vi "myRIO_BRig_RT_v0,53__PortC.vi"() -> ()   [LabVIEW 2014]
uses:
  myRIO_BRig_RT__Case_Exp_stateList.ctl
  myRIO_BRig_RT__Case_NonExp_stateList.ctl
  <vilib>/Platform/TimedLoop/XDataNode/timing_clust.ctl
  <vilib>/Platform/TimedLoop/XDataNode/nitl_modes.ctl
  <vilib>/Platform/TimedLoop/XDataNode/wakeup.ctl
  <vilib>/WebDAVClient/Advanced/SessionHandle.ctl
  <vilib>/myRIO/Common/Instrument Driver Framework/myRIO v1.0/UART/vis/myRIO v1.0 Close UART.vi
  <vilib>/FPGAPlugInAG/myRIO-1900/niLvFpga_Open_myRIO-1900.vi
  <vilib>/rvi/interface/common/dynamic/niFpgaDynamicAddResources.vi
  <vilib>/Utility/error.llb/Error Cluster From Error Code.vi
  <vilib>/rvi/errors/niLvFpgaAdjustHostInterfaceError.vi
  <vilib>/FPGAPlugInAG/Dynamic/niLvFpga_Close_Dynamic.vi
  <vilib>/myRIO/Common/Instrument Driver Framework/Utilities/vis/FPGA Ref Manager.vi
  <vilib>/myRIO/Common/Instrument Driver Framework/myRIO v1.0/myRIO v1.0 Reset FPGA.vi
  <vilib>/myRIO/Common/Instrument Driver Framework/myRIO v1.0/IRQ/vis/myRIO v1.0 IRQ Info FGV.vi
  <vilib>/myRIO/Common/Instrument Driver Framework/myRIO v1.0/IRQ/vis/myRIO v1.0 Timer IRQ Info FGV.vi
  <vilib>/myRIO/Common/Instrument Driver Framework/myRIO v1.0/IRQ/vis/myRIO v1.0 ISR Agent.vi
  <vilib>/rvi/interface/nirviOpenFPGA/nirviOpenFPGA.xnode
  myRIO_BRig_FPGA_v3,41__PortC__v2__build.lvbitx
  myRIO_BRig_FPGA_v3,41__PortC__v2.vi
  <vilib>/rvi/interface/nirviReadWriteControl/nirviReadWriteControl.xnode
  <vilib>/Platform/TimedLoop/XDataNode/XDataNode.xnode
  <vilib>/rvi/interface/nirviCloseFPGA/nirviCloseFPGA.xnode
  <vilib>/Platform/TimedLoop/XDataNode/XDNodeRunTimeDep.lvlib
  <vilib>/rvi/interface/Simulation/niFpgaSimulationCallBeginRW.vi
  <vilib>/myRIO/Instrument Drivers/Utilities/Utilities.lvlib
  <vilib>/WebDAVClient/NI_WebDAV.lvlib
  NiFpgaLv.dll
panel:
  in  "Recording_p2":bool
  in  "Recording":bool
  out "error out 3":errorcluster
  out "error out 2":errorcluster
  in  "laser_power":dbl
  in  "f_millisec2count":dbl=117.0
  in  "laser_Tshutter":dbl=2.0
  in  "laser_Freq":dbl=10.0
  in  "laser_Tpeak":dbl=2.0
  in  "laser_duration":u16
  out "error out":errorcluster
  in  "LC_Cue1_All_Count":u16
  in  "LC_Cue1_First_Count":u16
  in  "LC_Cue1_All_delayOpt":bool
  in  "LC_ENL1_All_delayOpt":bool
  in  "LC_ENL1_All_Count":u16
  in  "LC_ENL1_First_Count":u16
  in  "LC_Cue1_First_delayOpt":bool
  in  "LC_ENL1_First_delayOpt":bool
  in  "Tcycle_Cue_max":u16=1000 caption="Max [ms]" min=5 max=5000 step=5
  in  "Tcycle_Cue_min":u16=1000 caption="Min [ms]" min=5 max=5000 step=5
  in  "SendData":bool
  out "cSpout":enum16{"Left", "Right"}(ring) caption="Left or Right Spout"
  out "A4":u32 caption="LickCounter_Right"
  out "A2":u32 caption="LickCounter_Left"
  in  "laserResponse_wrong_LED":bool
  out "error_initTrial":errorcluster
  out "error_Selection_pre":errorcluster
  out "error_Selection":errorcluster
  out "SelectWrong":bool
  out "SelectReward":bool
  in  "Left(F)_or_Right(T)":bool
  in  "ignoreWrong":bool
  in  "SelectionState":bool
  in  "laserResponse_wrong":bool
  in  "laserResponse_reward":bool
  in  "laserResponse_reward_LED":bool
  out "nRewards_Right":u16 caption="# Rewards Total (Right)"
  out "nRewards_Left":u16 caption="# Rewards Total (Left)"
  out "nRewards_cur":u16 caption="# Rewards in Current Block"
  out "TpB_target":u16 caption="Target Trials Per Block"
  out "cState_NonExp":T1 caption="NonExperimental State"
  out "iBlock":u16 caption="Current Block"
  out "cState":T2 caption="Experimental State"
  out "iTrial":u16 caption="Current Trial"
  in  "warmupType":bool
  in  "TestConnection":bool
  in  "warmup":bool caption="WarmUp"
  in  "Host Filename Prefix":string="Exp1_TM2"
  out "Connected To Host?":bool
  in  "Host Password":string="sabalab"
  in  "Host UserName":string="Test2"
  in  "sp_RightSpout":u16(slide)=2 max=2 step=1 scale=0.0..2.0
  in  "sp_LeftSpout":u16(slide)=2 max=2 step=1 scale=0.0..2.0
  in  "BUR_max":u16 caption="Count Reward Structure  (0 = off)"
  in  "LC_Wrong_Probability":u16
  in  "LC_Wrong_Trial":u16(slide) max=2 step=1 scale=0.0..2.0
  in  "LC_Wrong_Block":u16(slide) max=2 step=1 scale=0.0..2.0
  in  "LC_Wrong_OnOff":bool
  in  "LC_Reward_Probability":u16
  in  "LC_Reward_Trial":u16(slide) max=2 step=1 scale=0.0..2.0
  in  "LC_Reward_Block":u16(slide) max=2 step=1 scale=0.0..2.0
  in  "LC_Reward_OnOff":bool
  in  "LC_Cue1_All_Probability":u16
  in  "LC_Cue1_All_Block":u16(slide) max=2 step=1 scale=0.0..2.0
  in  "LC_Cue1_All_OnOff":bool
  in  "LC_Cue1_First_Probability":u16
  in  "LC_Cue1_First_Block":u16(slide) max=2 step=1 scale=0.0..2.0
  in  "LC_Cue1_First_OnOff":bool
  in  "LC_ENL1_All_Probability":u16 max=100 step=1
  in  "LC_ENL1_All_Block":u16(slide) max=2 step=1 scale=0.0..2.0
  in  "LC_ENL1_All_OnOff":bool
  in  "LC_ENL1_First_Probability":u16 max=100 step=1
  in  "LC_ENL1_First_Block":u16(slide) max=2 step=1 scale=0.0..2.0
  in  "Tcycle_Timeout":u16=1000 caption="Timeout Time [ms]" min=10 max=10000 step=1
  in  "Tcycle_Wrong":u16=1000 caption="Wrong Time [ms]" min=10 max=10000 step=1
  in  "Tcycle_Selection":u16=1000 caption="Answer Time [ms]" min=1 max=10000 step=1
  in  "Tcycle_RewardPost":u16=1000 caption="Consumption Time [ms]" min=250 max=10000 step=250
  in  "Tcycle_Reward_L":u16=500 caption="Reward Time [ms]" min=1 max=1000 step=1
  in  "Tcycle_Reward_R":u16=500 caption="Reward Time [ms]" min=1 max=1000 step=1
  in  "TpB_Max_R":u16=4 caption="Max TrialsPerBlock" min=1 max=12 step=1
  in  "TpB_Min_R":u16=4 caption="Min TrialsPerBlock" min=1 max=12 step=1
  in  "TpB_Max_L":u16=4 caption="Max TrialsPerBlock" min=1 max=12 step=1
  in  "TpB_Min_L":u16=4 caption="Min TrialsPerBlock" min=1 max=12 step=1
  in  "BUR_min":u16 caption="Count Reward Structure  (0 = off)"
  in  "TrialUntilReward":bool caption="Ignore Wrong \nSelection"
  in  "CueCycles":u16=1 caption="Cue Structure" min=1 max=1 step=1
  in  "MTrig_Laser_Tcycle":u16=10 caption="Time [ms]"
  in  "MTrig_Laser_trig":bool
  in  "MTrig_Audio_trig__R":bool caption="Trigger Audio"
  in  "MTrig_Audio_trig__L":bool caption="Trigger Audio"
  in  "RewCalib_Trig_R":bool caption="Calibrate_R"
  in  "RewCalib_Trig_L":bool caption="Calibrate_L"
  in  "MTrig_Solenoid_Tcycle__R":u16=300 caption="Time [ms]"
  in  "MTrig_Solenoid_Tcycle__L":u16=300 caption="Time [ms]"
  in  "MTrig_Solenoid_trig__R":bool caption="Solenoid"
  in  "MTrig_Solenoid_trig__L":bool caption="Solenoid"
  in  "STOP_abort":bool caption="Stop LabView\n(Stops myRio and FPGA)"
  in  "STOP_endBlock":bool caption="Stop Experiment\n@ End of Block"
  in  "STOP_endTrial":bool caption="Stop Experiment\n@ End of Trial"
  in  "START":bool caption="Start Experiment"
  in  "Tcycle_CuePenalty":u16=1000 caption="Penalty [ms]" min=1 max=10000 step=1
  in  "Audio_Amp__R":u16=100 caption="Amp"
  in  "Audio_Freq__R":u16=5 caption="Freq [kHz]" max=14 step=1
  in  "Audio_Amp__L":u16=100 caption="Amp"
  in  "Audio_Freq__L":u16=5 caption="Freq [kHz]" max=14 step=1
  in  "LC_Wrong_Tdelay":u16
  in  "LC_Cue1_All_Tdelay":u16
  in  "LC_ENL1_All_Tdelay":u16
  in  "LC_Reward_Tdelay":u16
  in  "LC_Cue1_First_Tdelay":u16
  in  "LC_ENL1_First_Tdelay":u16
  in  "LC_ENL1_First_OnOff":bool
  in  "Tcycle_ENLPenalty":u16=100 caption="Penalty [ms]" min=10 max=10000 step=10
  in  "Tcycle_ENL_max":u16=1000 caption="Max [ms]" min=250 max=10000 step=250
  in  "Tcycle_ENL_min":u16=1000 caption="Min [ms]" min=250 max=10000 step=250
  # "Manual Control"
  # "Task Structure"
  # "Task Timing"
  # "Laser Control\n\n                                                    On/Off      Block        Probability [%]   Delay [ms]                              Count"
  # "Manual Solenoid Trigger\nLeft              Right"
  # "Master Structure"
  # "Enforced NonLick"
  # "Enforced NonLick 1"
  # "from end"
  # "Time = Cue Min"
  # "Min\n \n  \nMax"
  # "Switch Trial"
  # "from start"
  # "(1) = Switching\n(2) = Two Choice"
  # "from end"
  # "NonSwitch Trials"
  # "Cue"
  # "from start"
  # "Cue 1"
  # "from end"
  # "Switch Trial"
  # "from start"
  # "Cue then reward"
  # "Min"
  # "Max"
  # "from end"
  # "Cue with reward"
  # "NonSwitch Trials"
  # "Trial Per Block Structure\n       Left                    Right"
  # "from start"
  # "Spout Selection Control"
  # "Manual Speaker Trigger\nLeft              Right"
  # "Selection Reward"
  # "Answer Time\n         [ms]\n\n  \nWrong Choice Penalty\n         [ms]\n \n \nChoice Timeout Penalty\n         [ms]"
  # "Selection Wrong"
  # "Cue Control"
  # "Left              Right"
  # "State"
  # "Manual Laser Trigger"
  # "Freq [kHz]\n \n \nAmp\n \n\n \n\nSpeaker\nSetting"
  # "Reward Control\n                 Left              Right"
  # "Min = 1\nMax = 32k"
  # "Reward Time\n         [ms]"
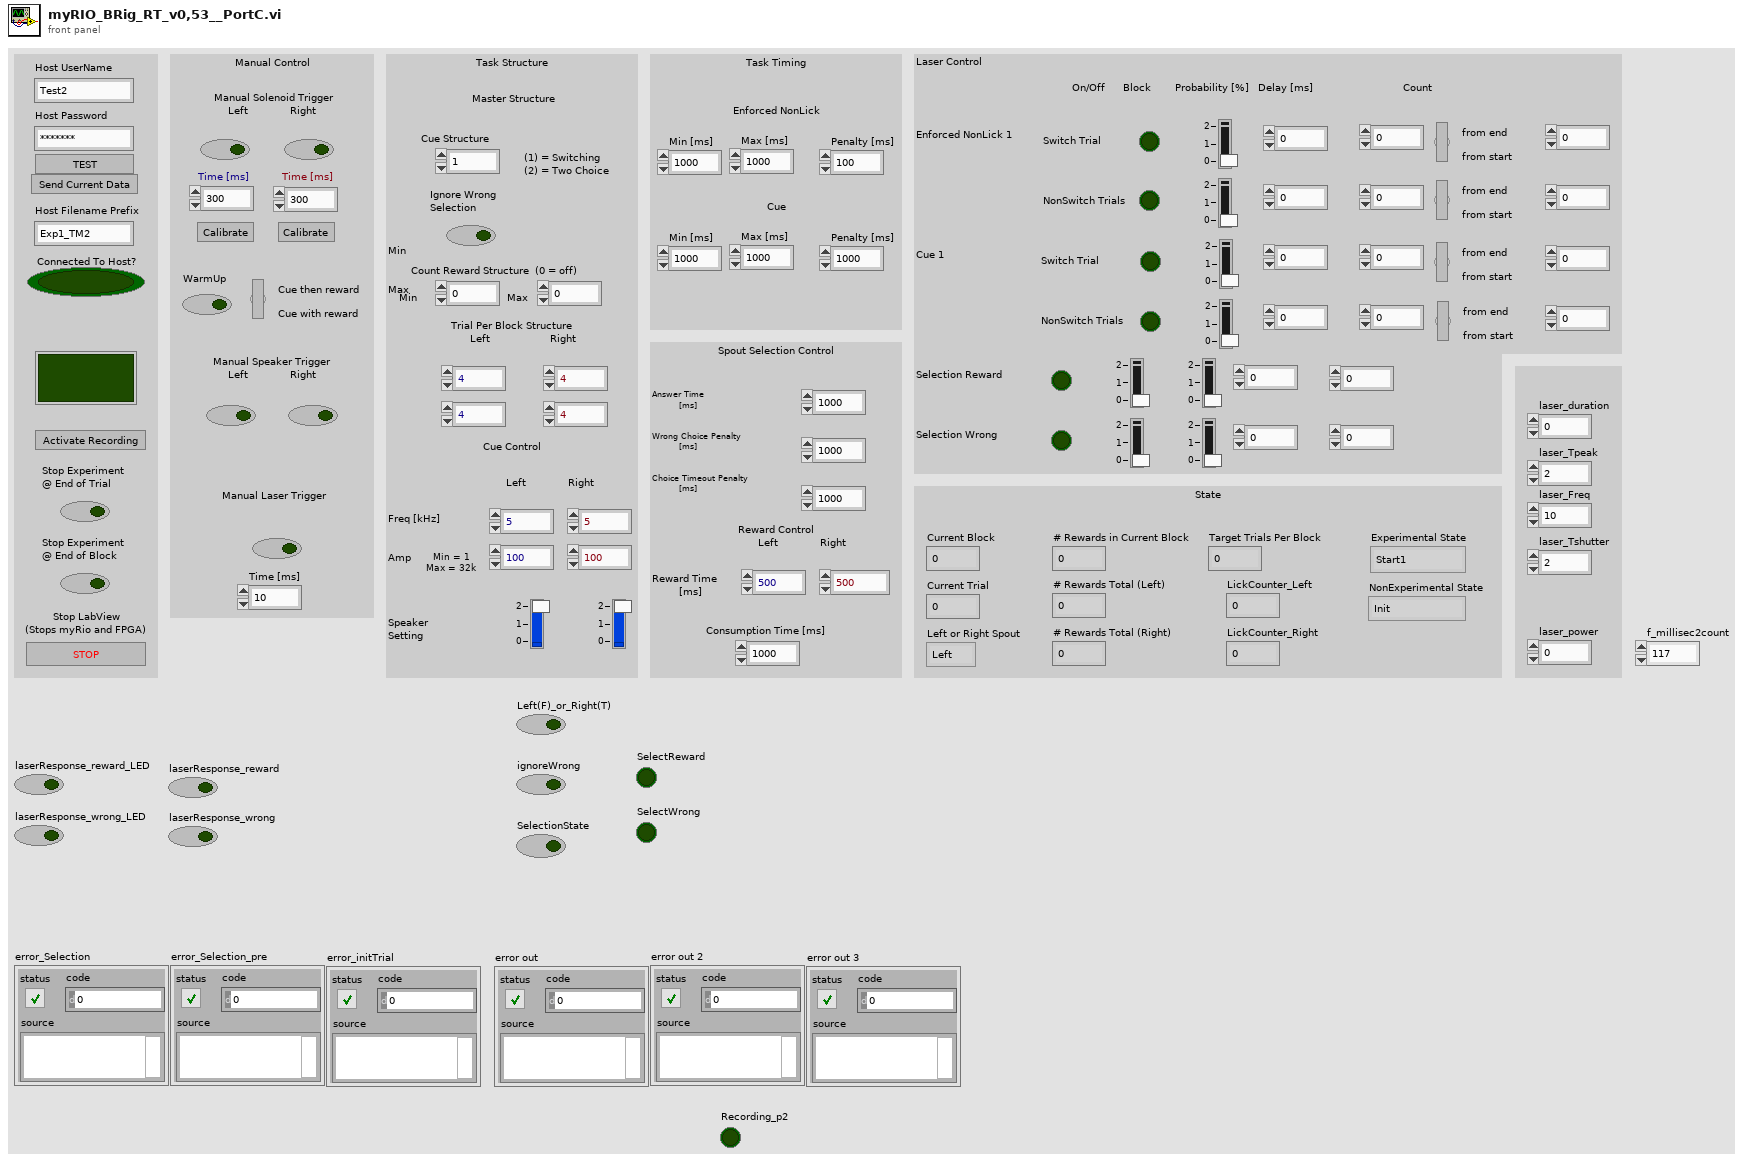
[diagram p1: front panel]
types:
  T1 = typedef "myRIO_BRig_RT__Case_NonExp_stateList.ctl" = enum16{"Init", "UploadSettings_pre", "UploadSettings_Read_dataExp", "UploadSettings_dataExp_1", "UploadSettings_Read_dataLC", "UploadSettings_dataLC_1", "UploadSettings_dataLC_2", "UploadSettings_Read_dataMTrig", "UploadSettings_dataMTrig_1", "UploadSettings_post", "Idle_pre", "IdleEmpty", "IdleEmpty2", "IdleEmpty3", "IdleEmpty4", "Idle", "Idle_2", "Idle_3", "Idle_4", "Idle_post", "Cue_pre__pre", "Cue_pre", "Cue", "Cue_post", "RewardCalibration_pre", "DispenseWater_pre__pre", "DispenseWater_pre", "DispenseWater", "DispenseWater_post", "TestConnection", "SendData", "End"}
  T2 = typedef "myRIO_BRig_RT__Case_Exp_stateList.ctl" = enum16{"Start1", "Start2", "Start3", "saveSettings1", "saveSettings2", "saveSettings3", "saveSettings4_LC_ENL", "saveSettings5_LC_Cue", "saveSettings6_LC_Other", "setSettings_Audio", "setSettings_Laser", "initBlock_pre", "initBlock", "initBlock2", "initBlock_post", "initTrial_pre", "initTrial", "initTrial2", "initTrial3", "initTrial4", "initTrial_LC_ENL1", "initTrial_LC_Cue1", "initTrial_post", "ENL1_pre", "ENL1", "ENL1_post", "ENL1Penalty_pre", "ENL1Penalty", "ENL2_pre", "ENL2", "ENL2Penalty_pre", "ENL2Penalty", "Cue1_pre", "Cue1", "Cue1_post", "Cue1Penalty_pre", "Cue1Penalty", "Cue2_pre", "Cue2", "Cue2Penalty_pre", "Cue2Penalty", "Selection_pre", "Selection", "Select_post", "SelectReward_pre", "SelectReward", "SelectRewardPost_pre", "SelectRewardPost", "SelectWrong_pre", "SelectWrong", "SelectWrong_post", "SelectTimeout_pre", "SelectTimeout", "SelectTimeout_post", "endTrial_pre", "endTrial1", "endTrial2", "endTrial3", "endTrial_post", "endBlock_pre", "endBlock", "endBlock_post", "endExp", "commConnect", "commUpload_pre", "commUpload_dataBlock", "commUpload_dataCurrent", "commUpload_dataExp", "commUpload_dataLC", "commUpload_dataTrial", "commUpload_post", "saveData_pre", "saveData_dataBlock", "saveData_dataCurrent", "saveData_dataExp", "saveData_dataLC", "saveData_dataTrial", "saveData_post", "empty_endBlock1", "empty_endBlock2", "empty_endTrial1", "empty_endTrial2", "empty_endTrial3", "empty_endTrial4", "empty_endTrial5"}
  T3 = typedef "XDNodeRunTimeDep.lvlib/timing_clust.ctl" = cluster{"Expected End [f-1]":u64, "Actual End [f-1]":u64, "Finished Late? [f-1]":bool, "Expected End [i-1]":u64, "Actual End [i-1]":u64, "Finished Late? [i-1]":bool, "Expected Start [i]":u64, "Actual Start [i]":u64, "Expected Start [f]":u64, "Actual Start [f]":u64, "Source Name":string, "Structure Name":string, "Period":i64, "Deadline":i64, "Offset":i64, "Start":i64, "Priority":i32, "Timeout":i32, "Mode":T4, "Wakeup Reason":T5, "Error":errorcluster, "Source Type":string, "Secondary Source Type":string, "Global End Time":u64, "Global Start Time":u64, "Frame Duration":u64, "Iteration Duration":u64, "Assigned CPU":i32, "I/O Scan Engine Mode":u32}
  T4 = typedef "XDNodeRunTimeDep.lvlib/nitl_modes.ctl" = enum32{"No Change", "Process missed periods, maintain original phase", "Discard missed periods, maintain original phase", "Process missed periods, ignore original phase", "Discard missed periods, ignore original phase"}
  T5 = typedef "XDNodeRunTimeDep.lvlib/wakeup.ctl" = enum32{"Normal", "Aborted", "Asynchronous wakeup", "Timing source error", "Timed loop error", "Timeout"}
  T6 = typedef "NI_WebDAV.lvlib/SessionHandle.ctl" = refnum<k1>
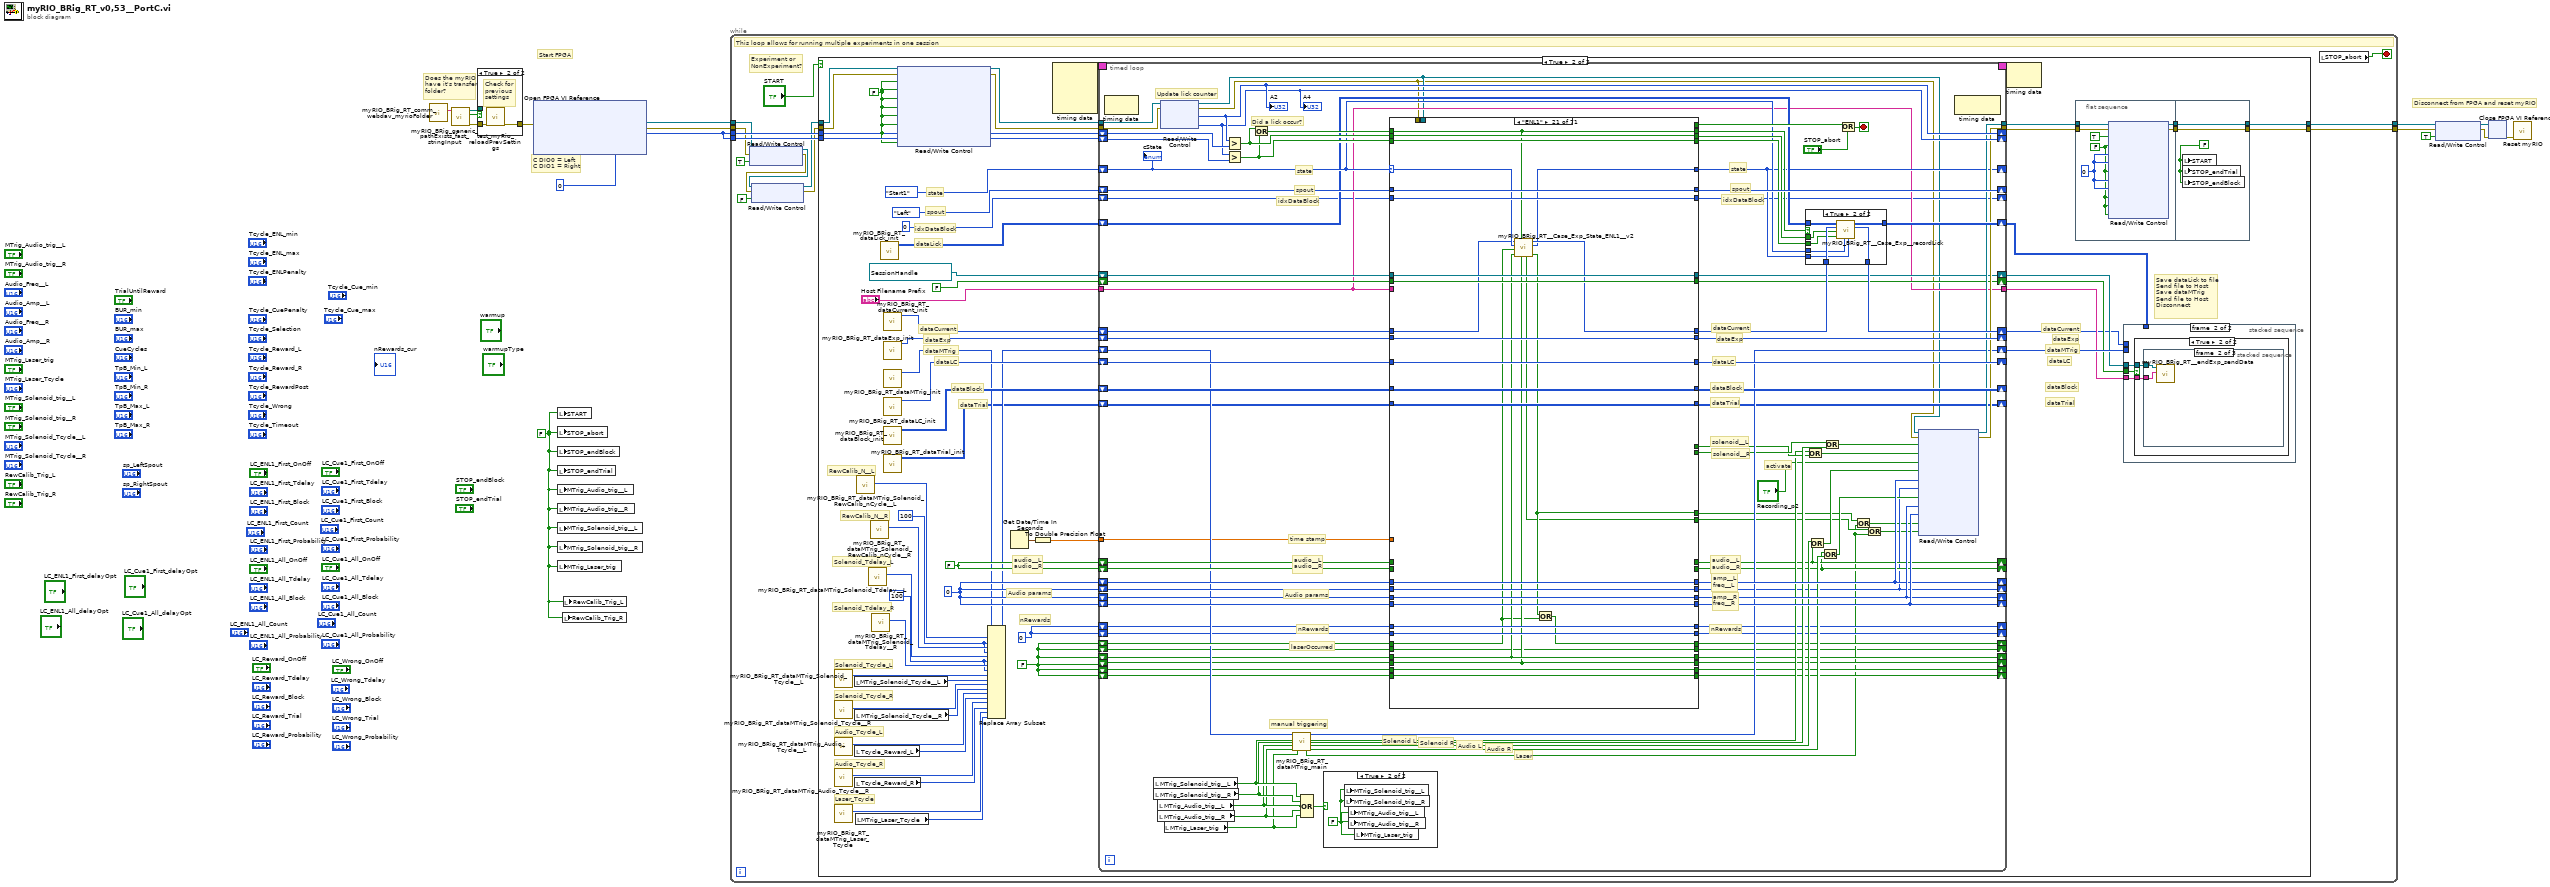
[diagram p0: block diagram]
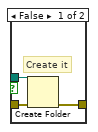
[diagram p2: hidden frame]
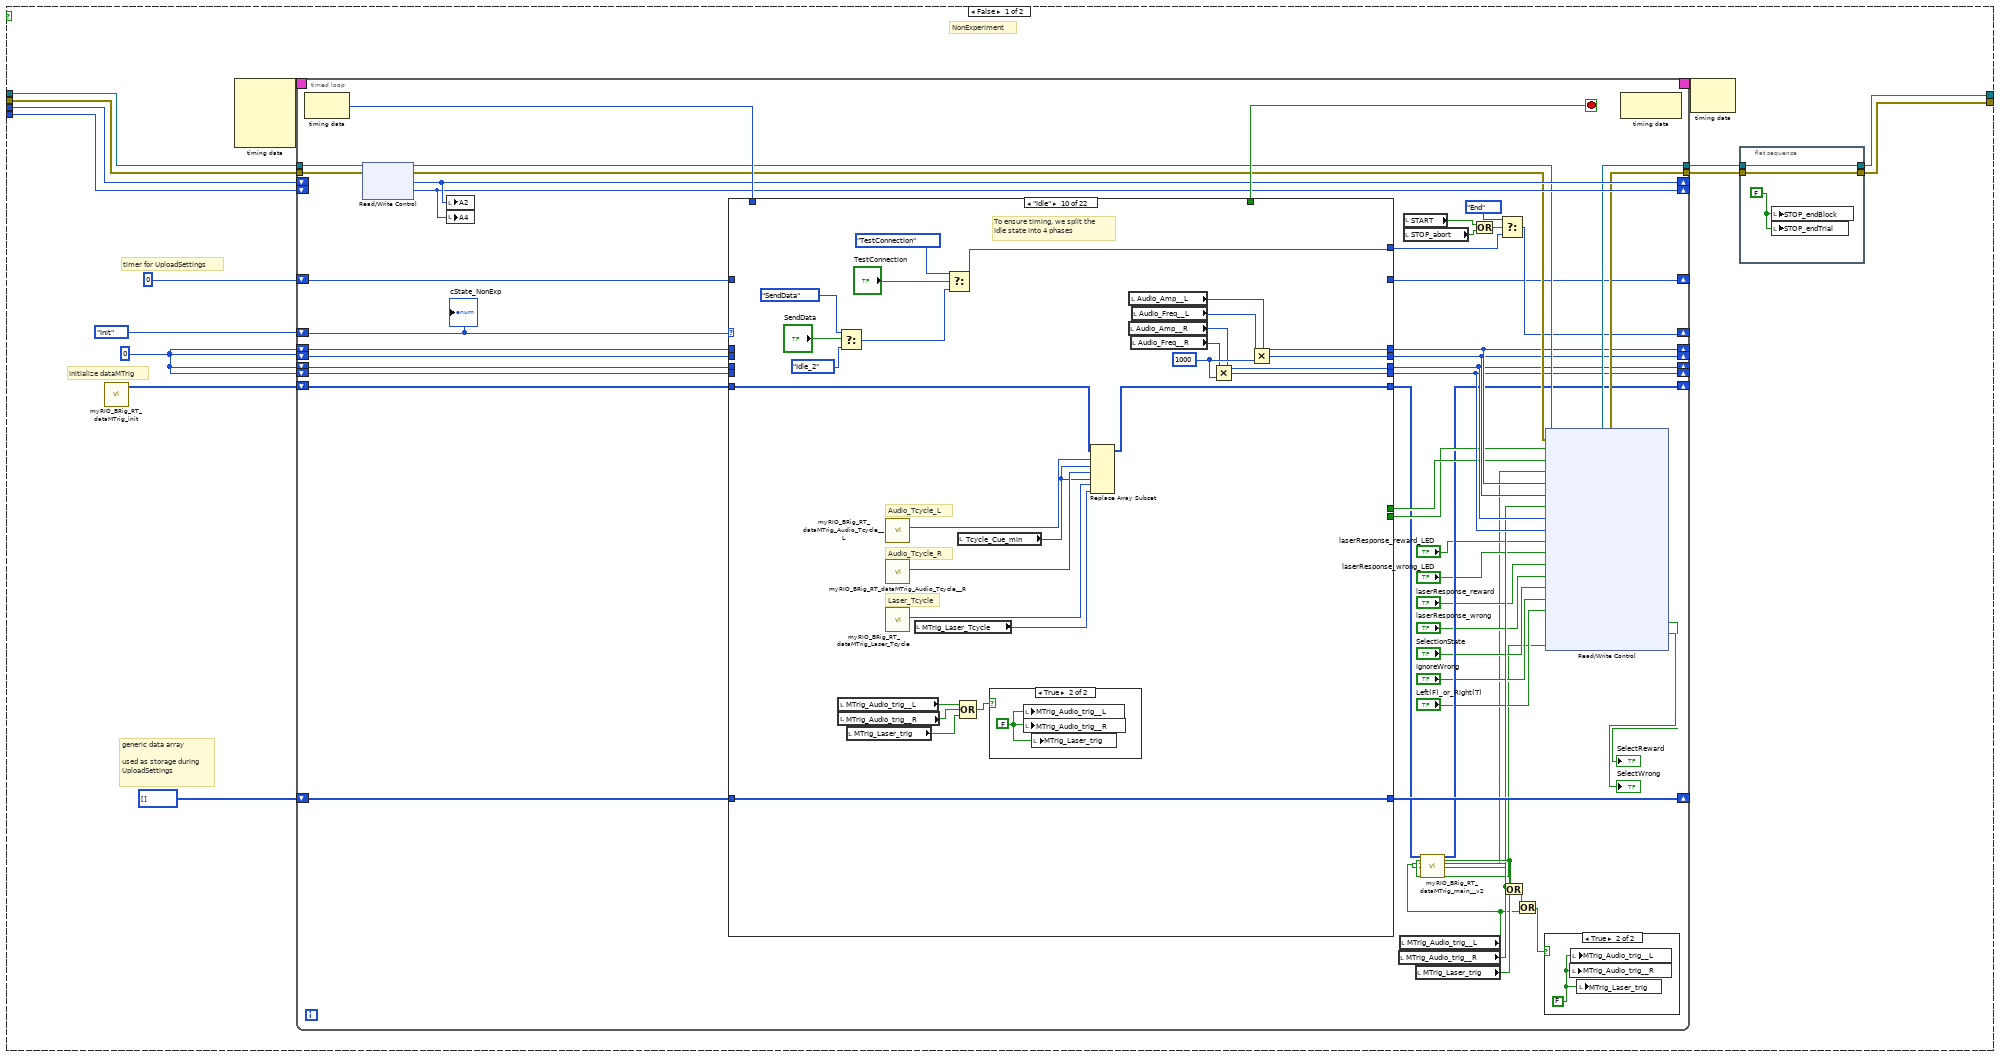
[diagram p3: hidden frame]
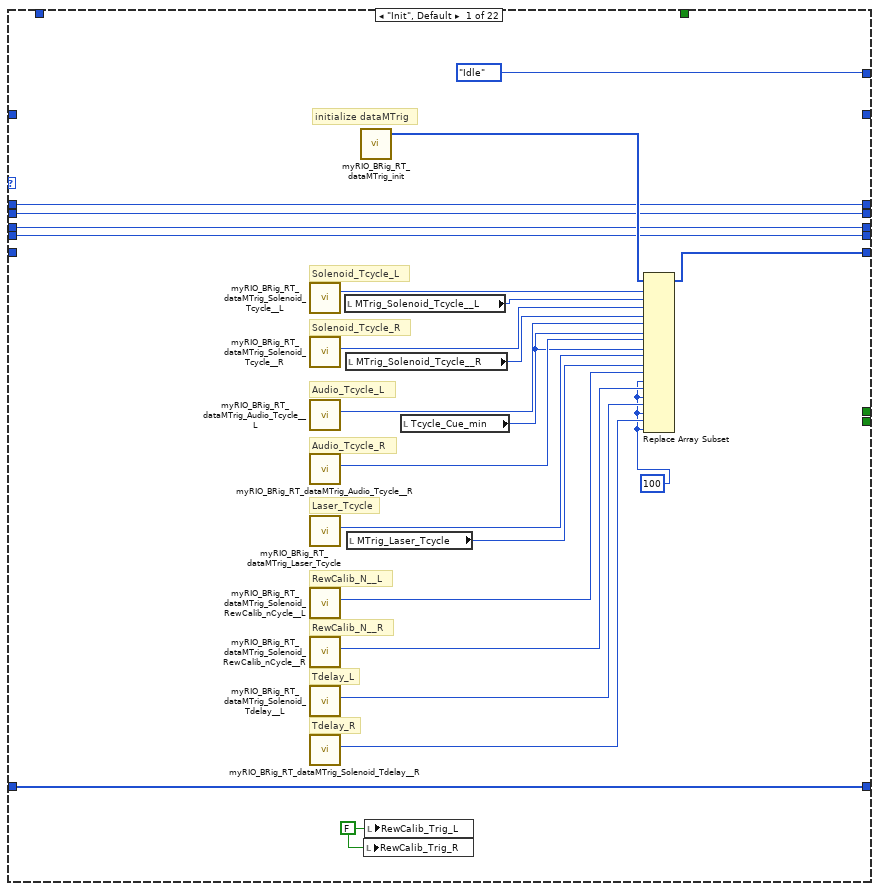
[diagram p5: hidden frame]
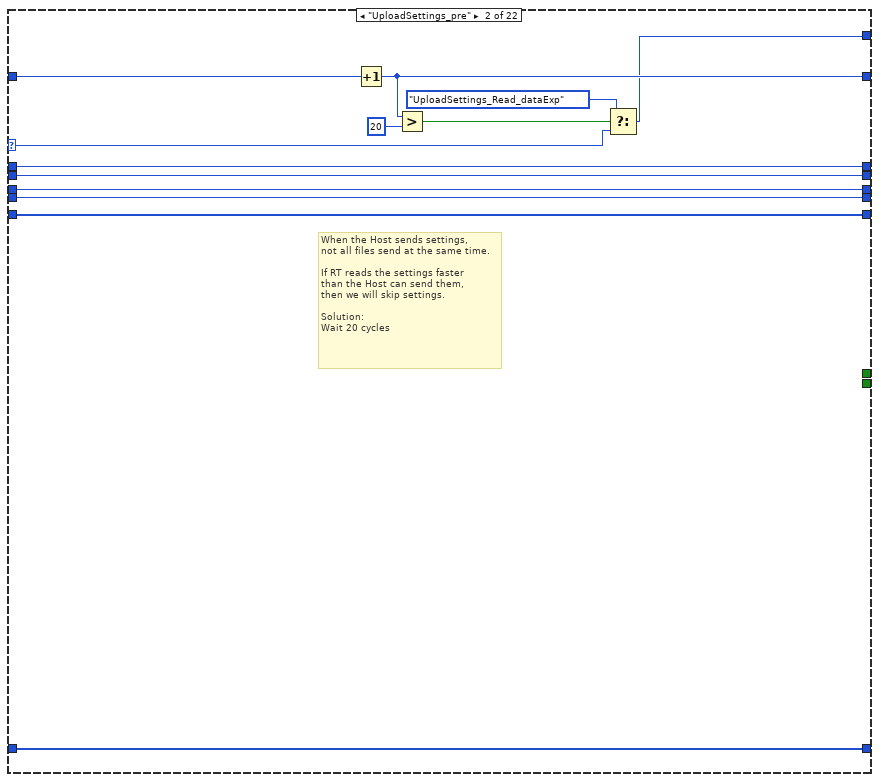
[diagram p6: hidden frame]
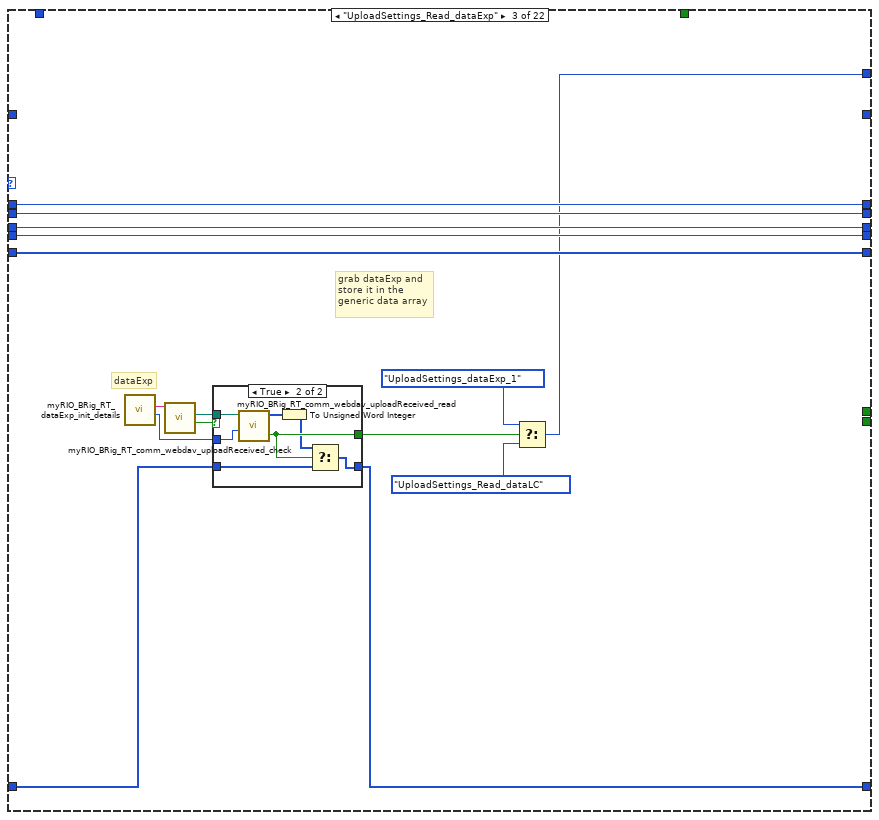
[diagram p7: hidden frame]
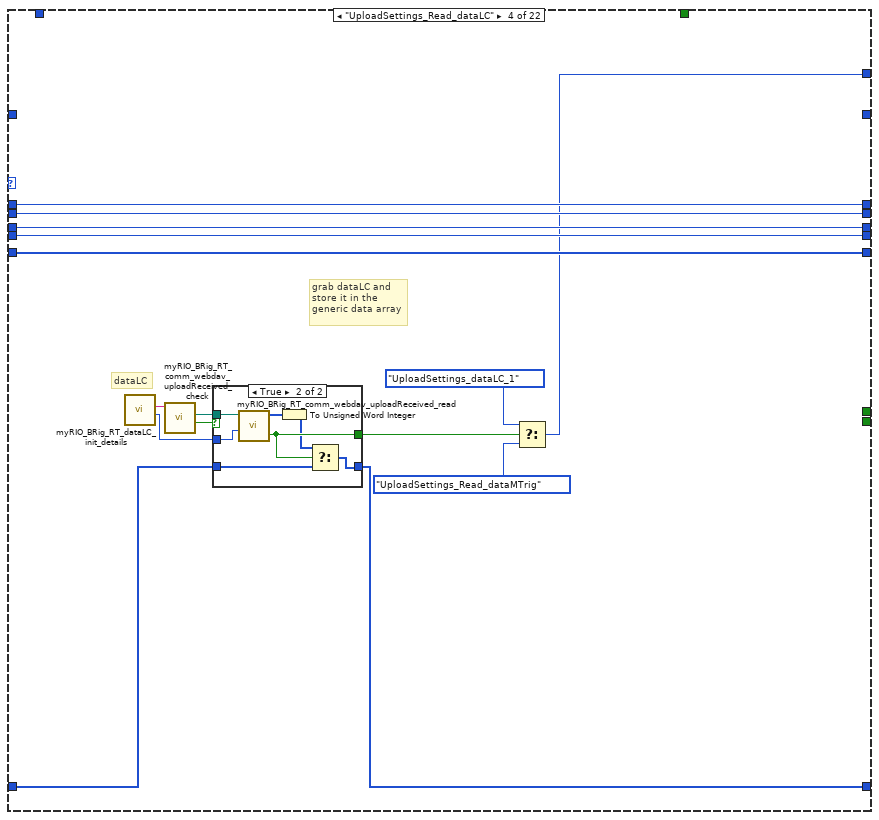
[diagram p9: hidden frame]
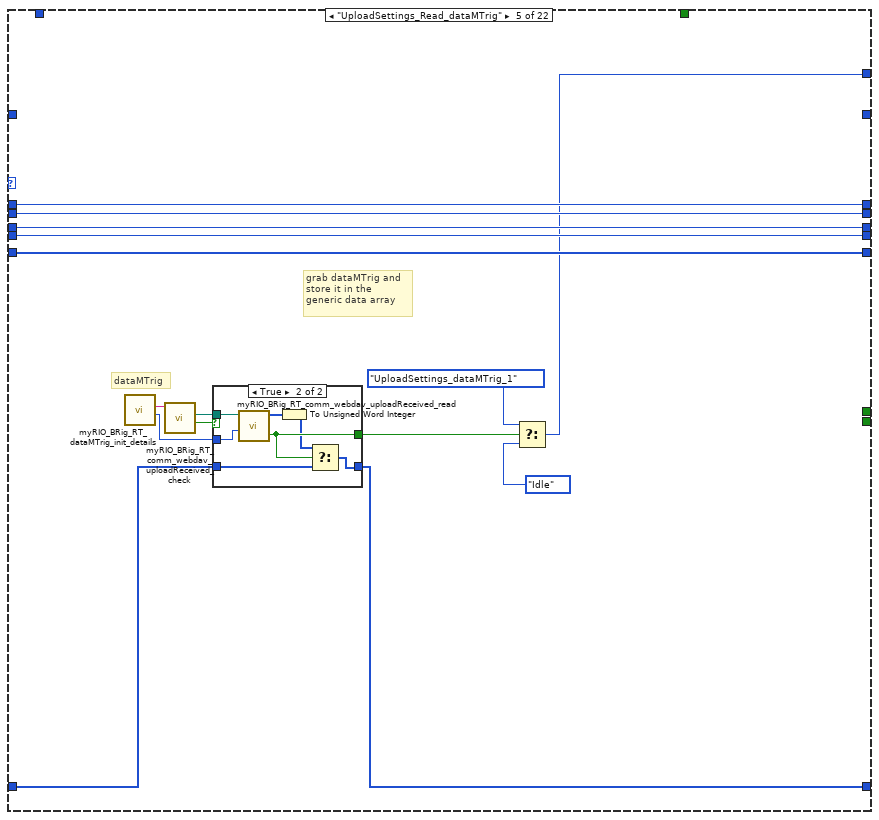
[diagram p11: hidden frame]
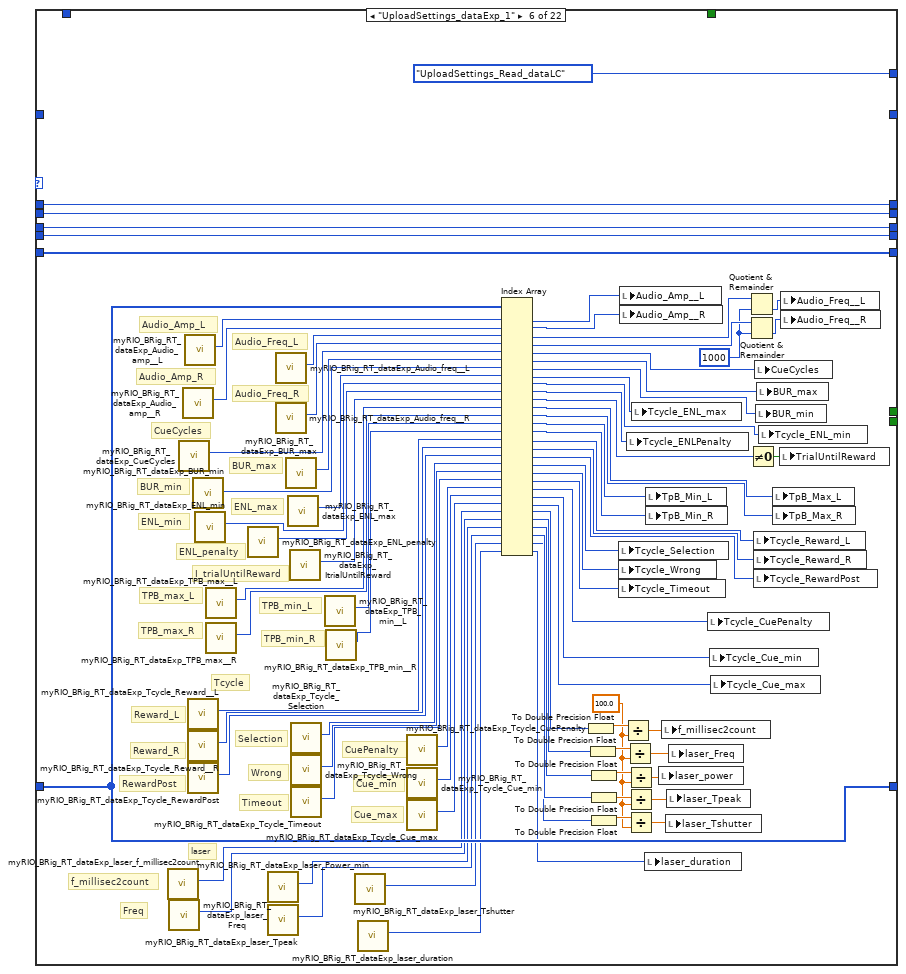
[diagram p13: hidden frame]
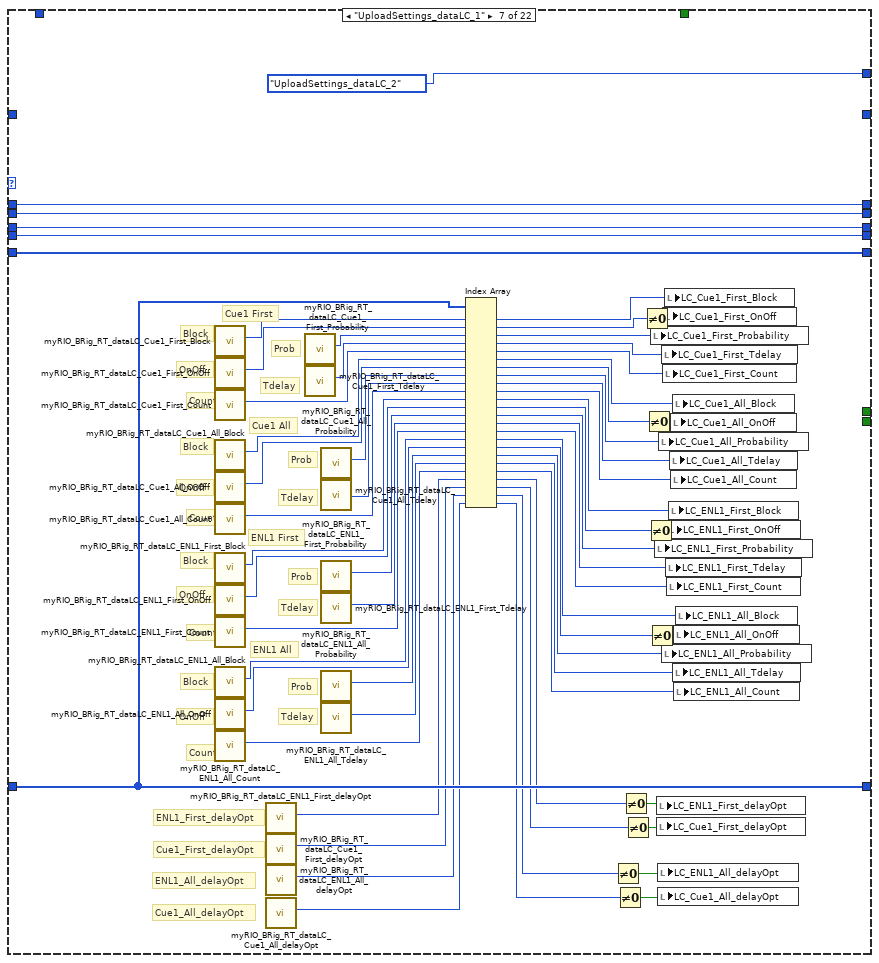
[diagram p14: hidden frame]
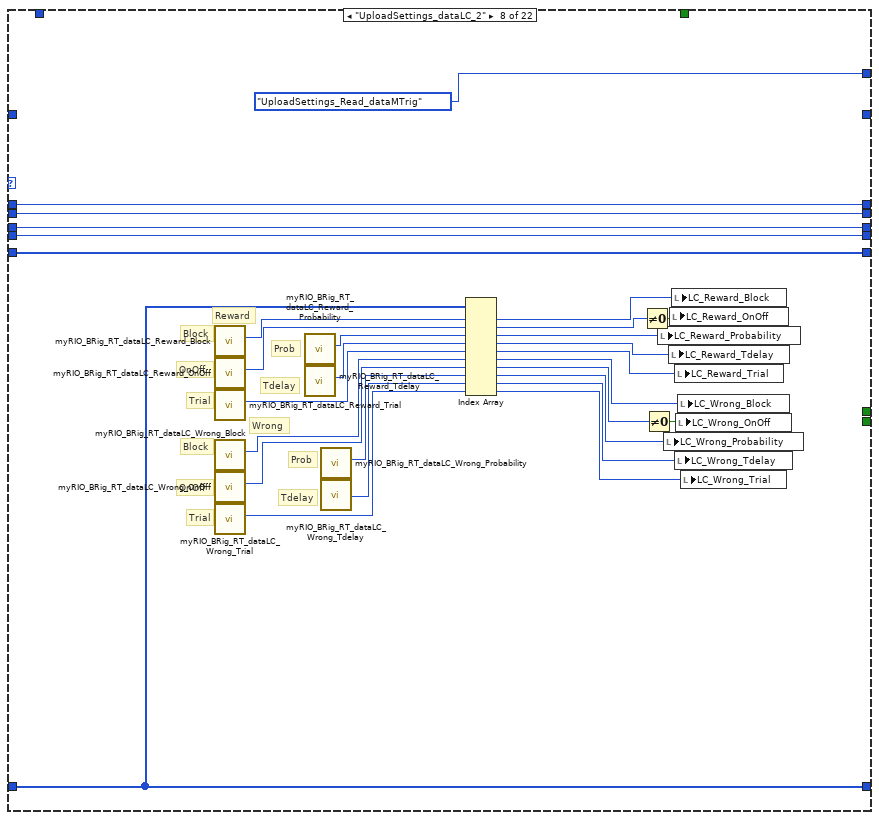
[diagram p15: hidden frame]
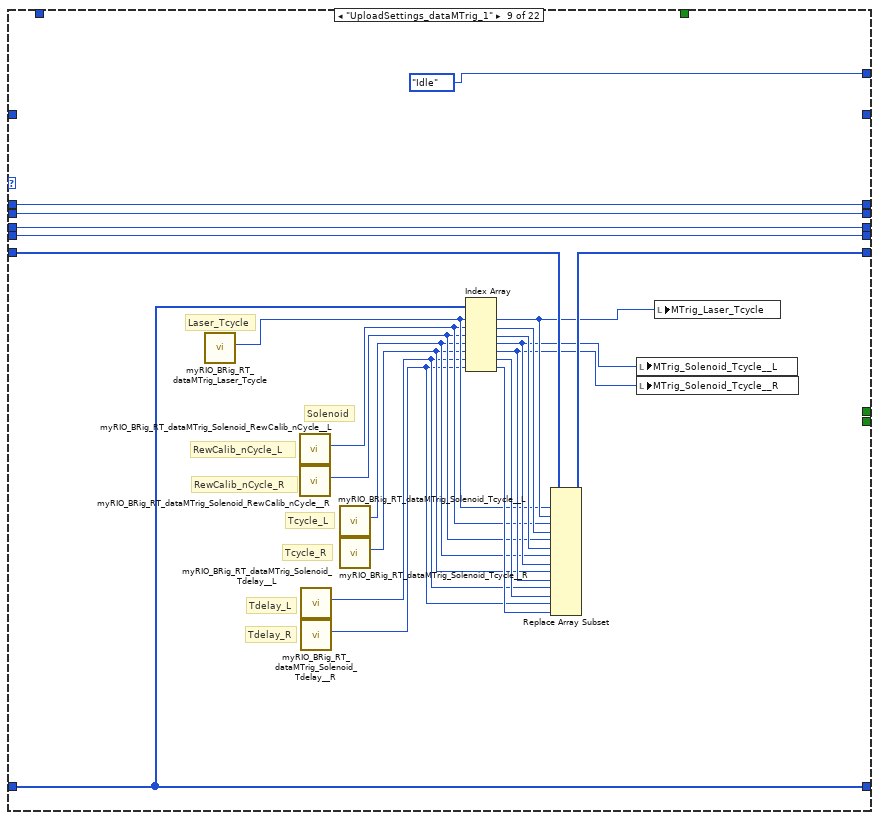
[diagram p16: hidden frame]
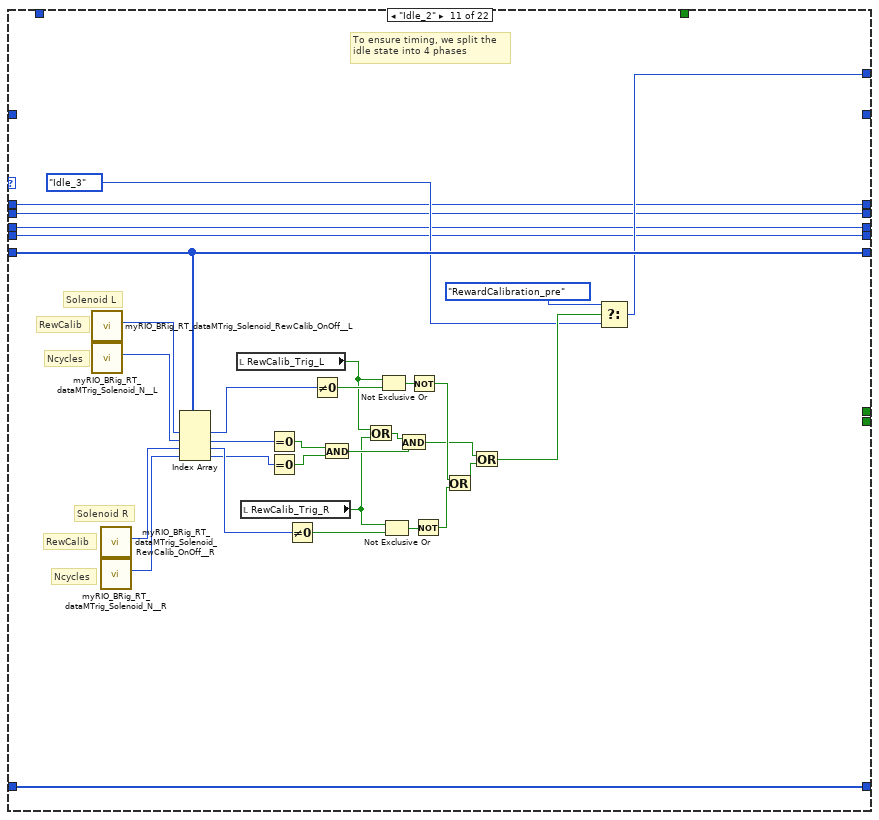
[diagram p18: hidden frame]
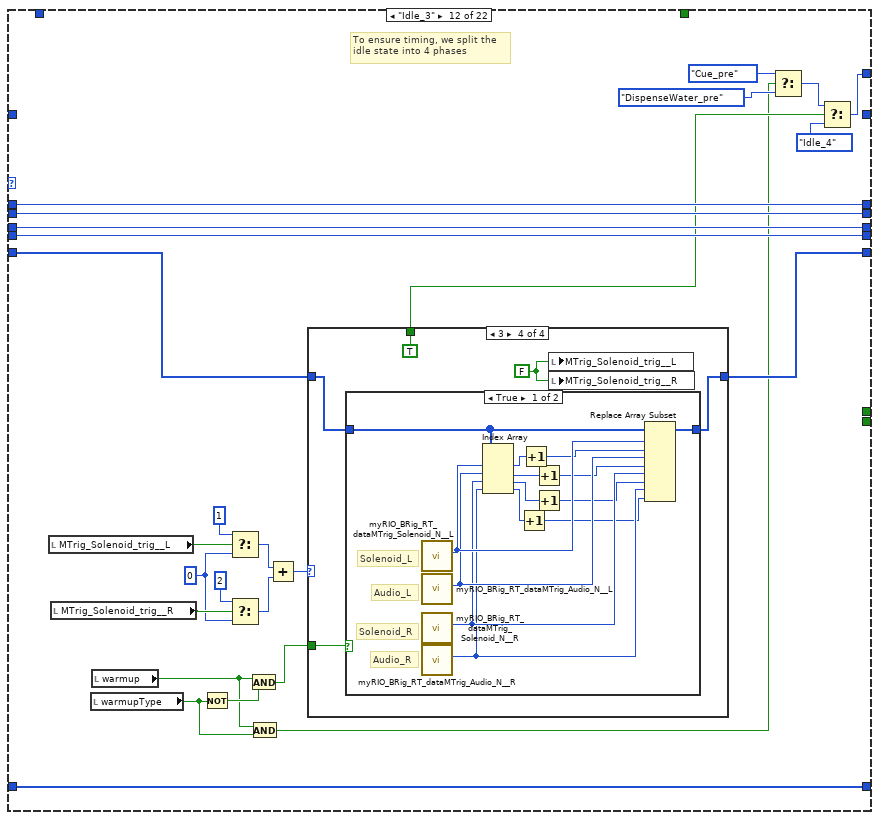
[diagram p19: hidden frame]
diagram:
  w9 = u32 0
  w6 = FALSE
  # "Does the myRIO\nhave it's transfer\nfolder?"
  # "C DIO0 = Left\nC DIO1 = Right"
  # "Start FPGA"
  # "Disconnect from FPGA and reset myRIO"
  n1 = call "myRIO_BRig_RT_comm_webdav_myrioFolder.vi"() -> ("output_myrioFolder"=w4:string)  [unwired: 11 in]
  n2 = call "myRIO_BRig_generic_pathExists_fast_stringInput.vi"("input_filePath"=w4) -> ("output_error"=w3:errorcluster, "output_Iexist"=w2:bool, "output_filePath"=w1:path)  [unwired: 8 in]
  n3 = case shown="True" w2 {
    tunnel: w1 -> [w18 _]
    tunnel: w3 -> [w17 w20]
    tunnel: [w16 w19] -> w5
    frame False {
      # "Create it"
      n4 = Create Folder(path (use dialog)=w18, error in=w17) -> (error out=w16:errorcluster)  [unwired: 1 in, 2 out]
    }
    frame True {
      # "Check for\nprevious\nsettings"
      n5 = call "test_myRio_reloadPrevSettings.vi"("input_error"=w20) -> ("output_error"=w19:errorcluster)  [unwired: 10 in]
    }
  }
  n6 = xnode "Open FPGA VI Reference"("error in"=w5) -> ("FPGA VI Reference Out"=w11:refnum<k20>, "error out"=w10:errorcluster)  [unwired: 1 in]
  n7 = local write "START"(w6) -> ()
  n8 = local write "STOP_abort"(w6) -> ()
  n9 = local write "STOP_endBlock"(w6) -> ()
  n10 = local write "STOP_endTrial"(w6) -> ()
  n11 = local write "MTrig_Audio_trig__L"(w6) -> ()
  n12 = local write "MTrig_Audio_trig__R"(w6) -> ()
  n13 = local write "MTrig_Solenoid_trig__L"(w6) -> ()
  n14 = local write "MTrig_Solenoid_trig__R"(w6) -> ()
  n15 = local write "MTrig_Laser_trig"(w6) -> ()
  n16 = local write "RewCalib_Trig_R"(w6) -> ()
  n17 = local write "RewCalib_Trig_L"(w6) -> ()
  n18 = while {
    tunnel: w11 -> [w24]
    tunnel: w10 -> [w29]
    tunnel: w9 -> [w32]
    tunnel: w9 -> [w31]
    tunnel: [w22] -> w8
    tunnel: [w21] -> w7
    stop <- w30 stop-if-true
    # "Experiment or\nNonExperiment?"
    # "This loop allows for running multiple experiments in one session"
    n19 = xnode "Read/Write Control"("FPGA VI Reference In"=w24, "error in"=w29, "Counts_Reset"=TRUE) -> ("FPGA VI Reference Out"=w26:refnum<k20>, "error out"=w27:errorcluster)
    n20 = xnode "Read/Write Control"("FPGA VI Reference In"=w26, "error in"=w27, "Counts_Reset"=FALSE) -> ("FPGA VI Reference Out"=w23:refnum<k20>, "error out"=w25:errorcluster)
    n21 = case shown="True" "START" {
      tunnel: w32 -> [w45 w932]
      tunnel: w31 -> [w44 w931]
      tunnel: w25 -> [w42 w882]
      tunnel: w23 -> [w43 w881]
      tunnel: [w40 w928] -> w22
      tunnel: [w38 w923] -> w21
      frame False {
        w37 = u16 0 ("Audio_Amp__L")
        # "generic data array\n\nused as storage during\nUploadSettings"
        # "timer for UploadSettings"
        # "initialize dataMTrig"
        # "NonExperiment"
        n22 = call "myRIO_BRig_RT_dataMTrig_init.vi"() -> ("output_dataMTrig"=w46:u16[])  [unwired: 5 in]
        n23 = node-c288() -> (w49:T3)  [unwired: 4 in]
        n24 = timed-loop {
          timing: w49 -> [_]
          timing-out: [_] -> w48
          shift-right: [w78] -> _
          shift-left: w46 -> [w102]
          shift-right: [w67] -> _
          shift-left: myRIO_BRig_RT__Case_NonExp_stateList."Init" ("Enum") -> [w92]
          shift-right: [w100] -> _
          shift-left: w45 -> [_]
          shift-right: [w99] -> _
          shift-left: w44 -> [_]
          tunnel: [w95] -> w41
          tunnel: [w93] -> w39
          tunnel: w42 -> [w98]
          tunnel: w43 -> [w97]
          shift-right: [w91] -> _
          shift-left: u16[] [] ("output_data") -> [w90]
          shift-right: [w85] -> _
          shift-left: w37 -> [w89]
          shift-right: [w84] -> _
          shift-left: w37 -> [w88]
          shift-right: [w83] -> _
          shift-left: w37 -> [w87]
          shift-right: [w82] -> _
          shift-left: w37 -> [w86]
          shift-right: [w53] -> _
          shift-left: u16 0 ("Audio_Amp__L") -> [w54]
          stop <- w103 stop-if-true
          n25 = node-c288() -> (w101:i64)  [unwired: 1 in]
          n26 = xnode "Read/Write Control"("FPGA VI Reference In"=w97, "error in"=w98) -> ("FPGA VI Reference Out"=w96:refnum<k20>, "error out"=w94:errorcluster, "A2_LickL"=w100:u32, "A4_LickR"=w99:u32)
          n27 = local write "A2"(w100) -> ()
          n28 = local write "A4"(w99) -> ()
          n29 = case shown="\"Idle\"" w92 {
            selector: w92 -> [_ w136 _ _ _ _ _ _ _ _ _ _ _ _ w591 _ _ w776 _ _ _ w873]
            tunnel: [myRIO_BRig_RT__Case_NonExp_stateList."Idle" ("Enum") w134 w141 w164 w187 myRIO_BRig_RT__Case_NonExp_stateList."UploadSettings_Read_dataLC" ("Enum") myRIO_BRig_RT__Case_NonExp_stateList."UploadSettings_dataLC_2" ("Enum") myRIO_BRig_RT__Case_NonExp_stateList."UploadSettings_Read_dataMTrig" ("f") myRIO_BRig_RT__Case_NonExp_stateList."Idle" ("Enum") w417 w438 w471 w562 myRIO_BRig_RT__Case_NonExp_stateList."Cue" ("t") w590 myRIO_BRig_RT__Case_NonExp_stateList."DispenseWater_pre" ("Enum") w718 w774 w801 myRIO_BRig_RT__Case_NonExp_stateList."Idle" ("Enum") myRIO_BRig_RT__Case_NonExp_stateList."Idle" ("Enum") w873] -> w68
            tunnel: [w119 w129 w151 w174 w197 w291 w354 w383 w403 w428 w453 w482 w560 w578 w604 w628 w755 w781 w812 w855 w865 w871] -> w79
            tunnel: [_ _ _ _ _ _ _ _ _ _ _ _ _ _ _ _ _ _ _ _ _ TRUE] -> w103
            tunnel: w102 -> [_ w129 w151 w174 w197 w291 w354 w383 w404 w427 w453 w483 w560 w579 w604 w614 w751 w782 w813 w855 w865 w871]
            tunnel: w101 -> [_ _ _ _ _ _ _ _ _ _ _ _ _ _ _ _ _ w786 _ _ _ _]
            tunnel: [w108 w128 w142 w165 w188 w235 w306 w355 w384 w412 w433 w465 w555 w566 w589 w605 w703 w759 w794 w843 w859 w866] -> w91
            tunnel: w90 -> [w108 w128 w143 w166 w189 w235 w306 w355 w384 w412 w433 w465 w555 w566 w589 w605 w703 w759 w794 w843 w859 w866]
            tunnel: [w112 w132 w154 w177 w200 w288 w352 w358 w401 w423 w436 w475 w557 w586 w601 w608 w757 w792 w819 w846 w862 w869] -> w84
            tunnel: [w110 w130 w152 w175 w198 w286 w350 w356 w399 w422 w434 w477 w559 w584 w603 w606 w756 w790 w817 w844 w860 w867] -> w82
            tunnel: [w113 w133 w155 w178 w201 w289 w353 w359 w402 w421 w437 w474 w556 w588 w600 w609 w758 w793 w820 w847 w863 w870] -> w85
            tunnel: [w111 w131 w153 w176 w199 w287 w351 w357 w400 w420 w435 w476 w558 w585 w602 w607 w756 w791 w818 w845 w861 w868] -> w83
            tunnel: w89 -> [w113 w133 w155 w178 w201 w289 w353 w359 w402 _ w437 w474 w556 w588 w600 w609 w758 w793 w820 w847 w863 w870]
            tunnel: w88 -> [w112 w132 w154 w177 w200 w288 w352 w358 w401 _ w436 w475 w557 w586 w601 w608 w757 w792 w819 w846 w862 w869]
            tunnel: w87 -> [w111 w131 w153 w176 w199 w287 w351 w357 w400 _ w435 w476 w558 w585 w602 w607 w756 w791 w818 w845 w861 w868]
            tunnel: w86 -> [w110 w130 w152 w175 w198 w286 w350 w356 w399 _ w434 w477 w559 w584 w603 w606 _ w790 w817 w844 w860 w867]
            tunnel: [_ _ _ _ _ _ _ _ _ _ _ _ _ _ _ _ _ w783 _ _ _ _] -> w81
            tunnel: [_ _ _ _ _ _ _ _ _ _ _ _ _ _ _ _ _ w765 _ _ _ _] -> w80
            tunnel: w54 -> [_ w140 _ _ _ _ _ _ _ _ _ _ _ _ _ _ _ _ _ _ _ _]
            tunnel: [_ w139 _ _ _ _ _ _ _ _ _ _ _ _ _ _ _ _ _ _ _ _] -> w53
            frame "Init", Default {
              w109 = FALSE ("RewCalib_Trig_L")
              w105 = u16 100 ("new element/subarray")
              # "Tdelay_R"
              # "Tdelay_L"
              # "RewCalib_N__R"
              # "RewCalib_N__L"
              # "Solenoid_Tcycle_R"
              # "Solenoid_Tcycle_L"
              # "Laser_Tcycle"
              # "Audio_Tcycle_R"
              # "Audio_Tcycle_L"
              # "initialize dataMTrig"
              n30 = call "myRIO_BRig_RT_dataMTrig_Solenoid_Tcycle__L.vi"() -> ("output_Solenoid_Tcycle__L"=w121:i32)  [unwired: 11 in]
              n31 = call "myRIO_BRig_RT_dataMTrig_Solenoid_Tcycle__R.vi"() -> ("output_Solenoid_Tcycle__R"=w122:i32)  [unwired: 11 in]
              n32 = call "myRIO_BRig_RT_dataMTrig_Audio_Tcycle__L.vi"() -> ("output_Audio_Tcycle__L"=w123:i32)  [unwired: 11 in]
              n33 = call "myRIO_BRig_RT_dataMTrig_Audio_Tcycle__R.vi"() -> ("output_Audio_Tcycle__R"=w124:i32)  [unwired: 11 in]
              n34 = call "myRIO_BRig_RT_dataMTrig_Laser_Tcycle.vi"() -> ("output_Laser_Tcycle"=w125:i32)  [unwired: 11 in]
              n35 = call "myRIO_BRig_RT_dataMTrig_Solenoid_RewCalib_nCycle__L.vi"() -> ("output_Solenoid_RewCalib_nCycle__L"=w117:i32)  [unwired: 11 in]
              n36 = call "myRIO_BRig_RT_dataMTrig_Solenoid_RewCalib_nCycle__R.vi"() -> ("output_Solenoid_RewCalib_nCycle__R"=w116:i32)  [unwired: 11 in]
              n37 = call "myRIO_BRig_RT_dataMTrig_Solenoid_Tdelay__L.vi"() -> ("output_Solenoid_Tdelay__L"=w115:i32)  [unwired: 11 in]
              n38 = call "myRIO_BRig_RT_dataMTrig_Solenoid_Tdelay__R.vi"() -> ("output_Solenoid_Tdelay__R"=w114:i32)  [unwired: 11 in]
              n39 = local read "MTrig_Solenoid_Tcycle__L"() -> (w126:u16)
              n40 = local read "MTrig_Solenoid_Tcycle__R"() -> (w127:u16)
              n41 = local read "MTrig_Laser_Tcycle"() -> (w106:u16)
              n42 = call "myRIO_BRig_RT_dataMTrig_init.vi"() -> ("output_dataMTrig"=w120:u16[])  [unwired: 5 in]
              n43 = local write "RewCalib_Trig_R"(w109) -> ()
              n44 = local write "RewCalib_Trig_L"(w109) -> ()
              n45 = local read "Tcycle_Cue_min"() -> (w107:u16)
              n46 = Replace Array Subset(array=w120, new element #1=w126, index #1=w121, new element #2=w127, index #2=w122, new element #3=w107, index #3=w123, new element #4=w107, index #4=w124, new element #5=w106, index #5=w125, new element #6=w105, index #6=w117, new element #7=w105, index #7=w116, new element #8=w105, index #8=w115, new element #9=w105, index #9=w114) -> (w119:u16[])
            }
            frame "UploadSettings_pre" {
              # "When the Host sends settings,\nnot all files send at the same time.\n\nIf RT reads the settings faster\nthan the Host can send them,\nthen we will skip settings.\n\nSolution:\nWait 20 cycles"
              n47 = Increment(x=w140) -> (x+1=w139:u16)
              n48 = Greater?(x=w139, y=u16 20) -> (0:w137:bool)
              n49 = Select(t=myRIO_BRig_RT__Case_NonExp_stateList."UploadSettings_Read_dataExp", s=w137, f=w136) -> (s? t:f=w134:T1)
            }
            frame "UploadSettings_Read_dataExp" {
              # "grab dataExp and\nstore it in the\ngeneric data array"
              # "dataExp"
              n50 = call "myRIO_BRig_RT_dataExp_init_details.vi"() -> ("output_dataSize"=w147:i32, "output_dataName"=w150:string)  [unwired: 10 in]
              n51 = call "myRIO_BRig_RT_comm_webdav_uploadReceived_check.vi"("input_dataName"=w150) -> ("output_Iexist"=w149:bool, "output_dataPath"=w148:path)  [unwired: 9 in]
              n52 = case shown="True" w149 {
                tunnel: w148 -> [_ w163]
                tunnel: w147 -> [_ w162]
                tunnel: [_ w161] -> w146
                tunnel: w143 -> [w156 w160]
                tunnel: [w156 w157] -> w142
                frame False {
                }
                frame True {
                  n53 = call "myRIO_BRig_RT_comm_webdav_uploadReceived_read.vi"("input_dataSize"=w162, "input_filePath"=w163) -> ("output_Ivalid"=w161:bool, "output_data"=w159:i64[])  [unwired: 8 in]
                  n54 = To Unsigned Word Integer(number=w159) -> (unsigned 16bit integer=w158:u16[])
                  n55 = Select(t=w158, s=w161, f=w160) -> (s? t:f=w157:u16[])
                }
              }
              n56 = Select(t=myRIO_BRig_RT__Case_NonExp_stateList."UploadSettings_dataExp_1", s=w146, f=myRIO_BRig_RT__Case_NonExp_stateList."UploadSettings_Read_dataLC" ("t")) -> (s? t:f=w141:T1)
            }
            frame "UploadSettings_Read_dataLC" {
              # "grab dataLC and\nstore it in the\ngeneric data array"
              # "dataLC"
              n57 = call "myRIO_BRig_RT_dataLC_init_details.vi"() -> ("output_dataSize"=w170:i32, "output_dataName"=w173:string)  [unwired: 10 in]
              n58 = call "myRIO_BRig_RT_comm_webdav_uploadReceived_check.vi"("input_dataName"=w173) -> ("output_Iexist"=w172:bool, "output_dataPath"=w171:path)  [unwired: 9 in]
              n59 = case shown="True" w172 {
                tunnel: w171 -> [_ w186]
                tunnel: w170 -> [_ w185]
                tunnel: [_ w184] -> w169
                tunnel: w166 -> [w179 w183]
                tunnel: [w179 w180] -> w165
                frame False {
                }
                frame True {
                  n60 = call "myRIO_BRig_RT_comm_webdav_uploadReceived_read.vi"("input_dataSize"=w185, "input_filePath"=w186) -> ("output_Ivalid"=w184:bool, "output_data"=w182:i64[])  [unwired: 8 in]
                  n61 = To Unsigned Word Integer(number=w182) -> (unsigned 16bit integer=w181:u16[])
                  n62 = Select(t=w181, s=w184, f=w183) -> (s? t:f=w180:u16[])
                }
              }
              n63 = Select(t=myRIO_BRig_RT__Case_NonExp_stateList."UploadSettings_dataLC_1", s=w169, f=myRIO_BRig_RT__Case_NonExp_stateList."UploadSettings_Read_dataMTrig" ("t")) -> (s? t:f=w164:T1)
            }
            frame "UploadSettings_Read_dataMTrig" {
              # "grab dataMTrig and\nstore it in the\ngeneric data array"
              # "dataMTrig"
              n64 = call "myRIO_BRig_RT_dataMTrig_init_details.vi"() -> ("output_dataSize"=w193:i32, "output_dataName"=w196:string)  [unwired: 10 in]
              n65 = call "myRIO_BRig_RT_comm_webdav_uploadReceived_check.vi"("input_dataName"=w196) -> ("output_Iexist"=w195:bool, "output_dataPath"=w194:path)  [unwired: 9 in]
              n66 = case shown="True" w195 {
                tunnel: w194 -> [_ w209]
                tunnel: w193 -> [_ w208]
                tunnel: [_ w207] -> w192
                tunnel: w189 -> [w202 w206]
                tunnel: [w202 w203] -> w188
                frame False {
                }
                frame True {
                  n67 = call "myRIO_BRig_RT_comm_webdav_uploadReceived_read.vi"("input_dataSize"=w208, "input_filePath"=w209) -> ("output_Ivalid"=w207:bool, "output_data"=w205:i64[])  [unwired: 8 in]
                  n68 = To Unsigned Word Integer(number=w205) -> (unsigned 16bit integer=w204:u16[])
                  n69 = Select(t=w204, s=w207, f=w206) -> (s? t:f=w203:u16[])
                }
              }
              n70 = Select(t=myRIO_BRig_RT__Case_NonExp_stateList."UploadSettings_dataMTrig_1", s=w192, f=myRIO_BRig_RT__Case_NonExp_stateList."Idle" ("t")) -> (s? t:f=w187:T1)
            }
            frame "UploadSettings_dataExp_1" {
              w218 = 100.0 ("y")
              w236 = u16 1000 ("y")
              # "Freq"
              # "f_millisec2count"
              # "laser"
              # "Cue_max"
              # "Cue_min"
              # "CuePenalty"
              # "Timeout"
              # "Wrong"
              # "Selection"
              # "RewardPost"
              # "Reward_R"
              # "Reward_L"
              # "Tcycle"
              # "TPB_min_R"
              # "TPB_min_L"
              # "TPB_max_R"
              # "TPB_max_L"
              # "I_trialUntilReward"
              # "ENL_penalty"
              # "ENL_min"
              # "ENL_max"
              # "BUR_max"
              # "BUR_min"
              # "CueCycles"
              # "Audio_Freq_R"
              # "Audio_Freq_L"
              # "Audio_Amp_R"
              # "Audio_Amp_L"
              n71 = call "myRIO_BRig_RT_dataExp_laser_f_millisec2count.vi"() -> ("output_laser_f_millisec2count"=w232:i32)  [unwired: 11 in]
              n72 = call "myRIO_BRig_RT_dataExp_laser_Freq.vi"() -> ("output_laser_Freq"=w231:i32)  [unwired: 11 in]
              n73 = call "myRIO_BRig_RT_dataExp_CueCycles.vi"() -> ("output_CueCycles"=w279:i32)  [unwired: 11 in]
              n74 = call "myRIO_BRig_RT_dataExp_Audio_amp__R.vi"() -> ("output_Audio_amp__R"=w283:i32)  [unwired: 11 in]
              n75 = call "myRIO_BRig_RT_dataExp_Audio_amp__L.vi"() -> ("output_Audio_amp__L"=w285:i32)  [unwired: 11 in]
              n76 = call "myRIO_BRig_RT_dataExp_Tcycle_Reward__L.vi"() -> ("output_Tcycle_Reward__L"=w256:i32)  [unwired: 11 in]
              n77 = call "myRIO_BRig_RT_dataExp_Tcycle_Reward__R.vi"() -> ("output_Tcycle_Reward__R"=w255:i32)  [unwired: 11 in]
              n78 = call "myRIO_BRig_RT_dataExp_Tcycle_RewardPost.vi"() -> ("output_Tcycle_RewardPost"=w254:i32)  [unwired: 11 in]
              n79 = call "myRIO_BRig_RT_dataExp_BUR_min.vi"() -> ("output_BUR_min"=w276:i32)  [unwired: 11 in]
              n80 = call "myRIO_BRig_RT_dataExp_ENL_min.vi"() -> ("output_ENL_min"=w272:i32)  [unwired: 11 in]
              n81 = call "myRIO_BRig_RT_dataExp_TPB_max__L.vi"() -> ("output_TPB_max__L"=w264:i32)  [unwired: 11 in]
              n82 = call "myRIO_BRig_RT_dataExp_TPB_max__R.vi"() -> ("output_TPB_max__R"=w263:i32)  [unwired: 11 in]
              n83 = call "myRIO_BRig_RT_dataExp_ENL_penalty.vi"() -> ("output_ENL_penalty"=w271:i32)  [unwired: 11 in]
              n84 = call "myRIO_BRig_RT_dataExp_laser_Power_min.vi"() -> ("output_laser_Power_min"=w230:i32)  [unwired: 11 in]
              n85 = call "myRIO_BRig_RT_dataExp_laser_Tpeak.vi"() -> ("output_laser_Tpeak"=w229:i32)  [unwired: 11 in]
              n86 = call "myRIO_BRig_RT_dataExp_Audio_freq__L.vi"() -> ("output_Audio_freq__L"=w281:i32)  [unwired: 11 in]
              n87 = call "myRIO_BRig_RT_dataExp_Audio_freq__R.vi"() -> ("output_Audio_freq__R"=w280:i32)  [unwired: 11 in]
              n88 = call "myRIO_BRig_RT_dataExp_BUR_max.vi"() -> ("output_BUR_max"=w277:i32)  [unwired: 11 in]
              n89 = call "myRIO_BRig_RT_dataExp_ENL_max.vi"() -> ("output_ENL_max"=w273:i32)  [unwired: 11 in]
              n90 = call "myRIO_BRig_RT_dataExp_ItrialUntilReward.vi"() -> ("output_I_trialUntilReward"=w267:i32)  [unwired: 11 in]
              n91 = call "myRIO_BRig_RT_dataExp_Tcycle_Selection.vi"() -> ("output_Tcycle_Selection"=w253:i32)  [unwired: 11 in]
              n92 = call "myRIO_BRig_RT_dataExp_Tcycle_Wrong.vi"() -> ("output_Tcycle_Wrong"=w252:i32)  [unwired: 11 in]
              n93 = call "myRIO_BRig_RT_dataExp_Tcycle_Timeout.vi"() -> ("output_Tcycle_Timeout"=w251:i32)  [unwired: 11 in]
              n94 = call "myRIO_BRig_RT_dataExp_TPB_min__L.vi"() -> ("output_TPB_min__L"=w262:i32)  [unwired: 11 in]
              n95 = call "myRIO_BRig_RT_dataExp_TPB_min__R.vi"() -> ("output_TPB_min__R"=w261:i32)  [unwired: 11 in]
              n96 = call "myRIO_BRig_RT_dataExp_laser_Tshutter.vi"() -> ("output_laser_Tshutter"=w228:i32)  [unwired: 11 in]
              n97 = call "myRIO_BRig_RT_dataExp_laser_duration.vi"() -> ("output_laser_duration"=w227:i32)  [unwired: 11 in]
              n98 = call "myRIO_BRig_RT_dataExp_Tcycle_CuePenalty.vi"() -> ("output_Tcycle_CuePenalty"=w244:i32)  [unwired: 11 in]
              n99 = call "myRIO_BRig_RT_dataExp_Tcycle_Cue_min.vi"() -> ("output_Tcycle_Cue_min"=w243:i32)  [unwired: 11 in]
              n100 = call "myRIO_BRig_RT_dataExp_Tcycle_Cue_max.vi"() -> ("output_Tcycle_Cue_max"=w242:i32)  [unwired: 11 in]
              n101 = Index Array(array=w235, index #1=w285, index #2=w283, index #3=w281, index #4=w280, index #5=w279, index #6=w277, index #7=w276, index #8=w273, index #9=w272, index #10=w271, index #11=w267, index #12=w264, index #13=w263, index #14=w262, index #15=w261, index #16=w256, index #17=w255, index #18=w254, index #19=w253, index #20=w252, index #21=w251, index #22=w244, index #23=w243, index #24=w242, index #25=w232, index #26=w231, index #27=w230, index #28=w229, index #29=w228, index #30=w227) -> (element #1=w284:u16, element #2=w282:u16, element #3=w239:u16, element #4=w238:u16, element #5=w278:u16, element #6=w275:u16, element #7=w274:u16, element #8=w270:u16, element #9=w269:u16, element #10=w268:u16, element #11=w265:u16, element #12=w260:u16, element #13=w259:u16, element #14=w258:u16, element #15=w257:u16, element #16=w250:u16, element #17=w249:u16, element #18=w248:u16, element #19=w247:u16, element #20=w246:u16, element #21=w245:u16, element #22=w241:u16, element #23=w234:u16, element #24=w233:u16, element #25=w226:u16, element #26=w217:u16, element #27=w216:u16, element #28=w215:u16, element #29=w214:u16, element #30=w210:u16)
              n102 = To Double Precision Float(number=w226) -> (double precision float=w225:dbl)
              n103 = To Double Precision Float(number=w217) -> (double precision float=w223:dbl)
              n104 = To Double Precision Float(number=w216) -> (double precision float=w221:dbl)
              n105 = To Double Precision Float(number=w215) -> (double precision float=w220:dbl)
              n106 = To Double Precision Float(number=w214) -> (double precision float=w219:dbl)
              n107 = local write "Tcycle_Selection"(w247) -> ()
              n108 = local write "Tcycle_Wrong"(w246) -> ()
              n109 = local write "Tcycle_Timeout"(w245) -> ()
              n110 = local write "Audio_Amp__L"(w284) -> ()
              n111 = local write "Audio_Amp__R"(w282) -> ()
              n112 = Divide(x=w225, y=w218) -> (x/y=w224:dbl)
              n113 = Divide(x=w223, y=w218) -> (x/y=w222:dbl)
              n114 = Divide(x=w221, y=w218) -> (x/y=w213:dbl)
              n115 = Divide(x=w220, y=w218) -> (x/y=w212:dbl)
              n116 = Divide(x=w219, y=w218) -> (x/y=w211:dbl)
              n117 = local write "Tcycle_ENLPenalty"(w268) -> ()
              n118 = local write "Tcycle_ENL_max"(w270) -> ()
              n119 = local write "laser_duration"(w210) -> ()
              n120 = local write "TpB_Min_L"(w258) -> ()
              n121 = local write "TpB_Min_R"(w257) -> ()
              n122 = local write "laser_power"(w213) -> ()
              n123 = local write "f_millisec2count"(w224) -> ()
              n124 = local write "laser_Tshutter"(w211) -> ()
              n125 = local write "laser_Tpeak"(w212) -> ()
              n126 = local write "laser_Freq"(w222) -> ()
              n127 = local write "Tcycle_CuePenalty"(w241) -> ()
              n128 = local write "Tcycle_Cue_min"(w234) -> ()
              n129 = local write "Tcycle_Cue_max"(w233) -> ()
              n130 = Quotient & Remainder(x=w239, y=w236) -> (floor(x/y)=w240:u16)  [unwired: 1 out]
              n131 = Quotient & Remainder(x=w238, y=w236) -> (floor(x/y)=w237:u16)  [unwired: 1 out]
              n132 = Not Equal To 0?(x=w265) -> (x != 0?=w266:bool)
              n133 = local write "Tcycle_Reward_L"(w250) -> ()
              n134 = local write "Tcycle_Reward_R"(w249) -> ()
              n135 = local write "Tcycle_RewardPost"(w248) -> ()
              n136 = local write "CueCycles"(w278) -> ()
              n137 = local write "BUR_min"(w274) -> ()
              n138 = local write "BUR_max"(w275) -> ()
              n139 = local write "Tcycle_ENL_min"(w269) -> ()
              n140 = local write "TpB_Max_L"(w260) -> ()
              n141 = local write "TpB_Max_R"(w259) -> ()
              n142 = local write "TrialUntilReward"(w266) -> ()
              n143 = local write "Audio_Freq__L"(w240) -> ()
              n144 = local write "Audio_Freq__R"(w237) -> ()
            }
            frame "UploadSettings_dataLC_1" {
              # "Cue1_All_delayOpt"
              # "ENL1_All_delayOpt"
              # "Cue1_First_delayOpt"
              # "ENL1_First_delayOpt"
              # "ENL1 First"
              # "Cue1 All"
              # "Cue1 First"
              # "Count"
              # "Tdelay"
              # "Prob"
              # "OnOff"
              # "Block"
              # "ENL1 All"
              # "Count"
              # "Tdelay"
              # "Prob"
              # "OnOff"
              # "Block"
              # "Count"
              # "Tdelay"
              # "Prob"
              # "Block"
              # "OnOff"
              # "Count"
              # "Tdelay"
              # "Prob"
              # "OnOff"
              # "Block"
              n145 = call "myRIO_BRig_RT_dataLC_Cue1_First_Block.vi"() -> ("output_Cue1_First_Block"=w348:i32)  [unwired: 11 in]
              n146 = call "myRIO_BRig_RT_dataLC_Cue1_First_OnOff.vi"() -> ("output_Cue1_First_OnOff"=w346:i32)  [unwired: 11 in]
              n147 = call "myRIO_BRig_RT_dataLC_Cue1_First_Count.vi"() -> ("output_Cue1_First_Count"=w343:i32)  [unwired: 11 in]
              n148 = call "myRIO_BRig_RT_dataLC_Cue1_All_Block.vi"() -> ("output_Cue1_All_Block"=w330:i32)  [unwired: 11 in]
              n149 = call "myRIO_BRig_RT_dataLC_Cue1_All_OnOff.vi"() -> ("output_Cue1_All_OnOff"=w329:i32)  [unwired: 11 in]
              n150 = call "myRIO_BRig_RT_dataLC_Cue1_All_Count.vi"() -> ("output_Cue1_All_Count"=w340:i32)  [unwired: 11 in]
              n151 = call "myRIO_BRig_RT_dataLC_ENL1_First_Block.vi"() -> ("output_ENL1_First_Block"=w328:i32)  [unwired: 11 in]
              n152 = call "myRIO_BRig_RT_dataLC_ENL1_First_OnOff.vi"() -> ("output_ENL1_First_OnOff"=w339:i32)  [unwired: 11 in]
              n153 = call "myRIO_BRig_RT_dataLC_ENL1_First_Count.vi"() -> ("output_ENL1_First_Count"=w336:i32)  [unwired: 11 in]
              n154 = call "myRIO_BRig_RT_dataLC_ENL1_All_Block.vi"() -> ("output_ENL1_All_Block"=w335:i32)  [unwired: 11 in]
              n155 = call "myRIO_BRig_RT_dataLC_ENL1_All_OnOff.vi"() -> ("output_ENL1_All_OnOff"=w334:i32)  [unwired: 11 in]
              n156 = call "myRIO_BRig_RT_dataLC_ENL1_All_Count.vi"() -> ("output_ENL1_All_Count"=w331:i32)  [unwired: 11 in]
              n157 = call "myRIO_BRig_RT_dataLC_ENL1_First_delayOpt.vi"() -> ("output_ENL1_First_delayOpt"=w305:i32)  [unwired: 11 in]
              n158 = call "myRIO_BRig_RT_dataLC_Cue1_First_delayOpt.vi"() -> ("output_Cue1_First_delayOpt"=w304:i32)  [unwired: 11 in]
              n159 = call "myRIO_BRig_RT_dataLC_ENL1_All_delayOpt.vi"() -> ("output_ENL1_All_delayOpt"=w297:i32)  [unwired: 11 in]
              n160 = call "myRIO_BRig_RT_dataLC_Cue1_All_delayOpt.vi"() -> ("output_Cue1_All_delayOpt"=w296:i32)  [unwired: 11 in]
              n161 = call "myRIO_BRig_RT_dataLC_Cue1_First_Probability.vi"() -> ("output_Cue1_First_Probability"=w345:i32)  [unwired: 11 in]
              n162 = call "myRIO_BRig_RT_dataLC_Cue1_First_Tdelay.vi"() -> ("output_Cue1_First_Tdelay"=w344:i32)  [unwired: 11 in]
              n163 = call "myRIO_BRig_RT_dataLC_Cue1_All_Probability.vi"() -> ("output_Cue1_All_Probability"=w342:i32)  [unwired: 11 in]
              n164 = call "myRIO_BRig_RT_dataLC_Cue1_All_Tdelay.vi"() -> ("output_Cue1_All_Tdelay"=w341:i32)  [unwired: 11 in]
              n165 = call "myRIO_BRig_RT_dataLC_ENL1_First_Probability.vi"() -> ("output_ENL1_First_Probability"=w338:i32)  [unwired: 11 in]
              n166 = call "myRIO_BRig_RT_dataLC_ENL1_First_Tdelay.vi"() -> ("output_ENL1_First_Tdelay"=w337:i32)  [unwired: 11 in]
              n167 = call "myRIO_BRig_RT_dataLC_ENL1_All_Probability.vi"() -> ("output_ENL1_All_Probability"=w333:i32)  [unwired: 11 in]
              n168 = call "myRIO_BRig_RT_dataLC_ENL1_All_Tdelay.vi"() -> ("output_ENL1_All_Tdelay"=w332:i32)  [unwired: 11 in]
              n169 = Index Array(array=w306, index #1=w348, index #2=w346, index #3=w345, index #4=w344, index #5=w343, index #6=w330, index #7=w329, index #8=w342, index #9=w341, index #10=w340, index #11=w328, index #12=w339, index #13=w338, index #14=w337, index #15=w336, index #16=w335, index #17=w334, index #18=w333, index #19=w332, index #20=w331, index #21=w305, index #22=w304, index #23=w297, index #24=w296) -> (element #1=w347:u16, element #2=w326:u16, element #3=w325:u16, element #4=w324:u16, element #5=w323:u16, element #6=w319:u16, element #7=w318:u16, element #8=w317:u16, element #9=w316:u16, element #10=w315:u16, element #11=w314:u16, element #12=w313:u16, element #13=w312:u16, element #14=w311:u16, element #15=w298:u16, element #16=w310:u16, element #17=w309:u16, element #18=w308:u16, element #19=w307:u16, element #20=w299:u16, element #21=w302:u16, element #22=w300:u16, element #23=w293:u16, element #24=w292:u16)
              n170 = Not Equal To 0?(x=w293) -> (x != 0?=w295:bool)
              n171 = Not Equal To 0?(x=w292) -> (x != 0?=w294:bool)
              n172 = Not Equal To 0?(x=w302) -> (x != 0?=w303:bool)
              n173 = Not Equal To 0?(x=w300) -> (x != 0?=w301:bool)
              n174 = Not Equal To 0?(x=w326) -> (x != 0?=w327:bool)
              n175 = Not Equal To 0?(x=w318) -> (x != 0?=w322:bool)
              n176 = Not Equal To 0?(x=w313) -> (x != 0?=w321:bool)
              n177 = Not Equal To 0?(x=w309) -> (x != 0?=w320:bool)
              n178 = local write "LC_Cue1_First_Probability"(w325) -> ()
              n179 = local write "LC_ENL1_First_Probability"(w312) -> ()
              n180 = local write "LC_ENL1_First_delayOpt"(w303) -> ()
              n181 = local write "LC_Cue1_First_delayOpt"(w301) -> ()
              n182 = local write "LC_ENL1_All_delayOpt"(w295) -> ()
              n183 = local write "LC_Cue1_All_delayOpt"(w294) -> ()
              n184 = local write "LC_Cue1_All_Probability"(w317) -> ()
              n185 = local write "LC_Cue1_First_Tdelay"(w324) -> ()
              n186 = local write "LC_ENL1_All_Probability"(w308) -> ()
              n187 = local write "LC_Cue1_First_OnOff"(w327) -> ()
              n188 = local write "LC_Cue1_First_Count"(w323) -> ()
              n189 = local write "LC_Cue1_First_Block"(w347) -> ()
              n190 = local write "LC_ENL1_First_Tdelay"(w311) -> ()
              n191 = local write "LC_ENL1_First_OnOff"(w321) -> ()
              n192 = local write "LC_ENL1_First_Count"(w298) -> ()
              n193 = local write "LC_ENL1_First_Block"(w314) -> ()
              n194 = local write "LC_Cue1_All_Tdelay"(w316) -> ()
              n195 = local write "LC_Cue1_All_OnOff"(w322) -> ()
              n196 = local write "LC_Cue1_All_Count"(w315) -> ()
              n197 = local write "LC_Cue1_All_Block"(w319) -> ()
              n198 = local write "LC_ENL1_All_Tdelay"(w307) -> ()
              n199 = local write "LC_ENL1_All_OnOff"(w320) -> ()
              n200 = local write "LC_ENL1_All_Count"(w299) -> ()
              n201 = local write "LC_ENL1_All_Block"(w310) -> ()
            }
            frame "UploadSettings_dataLC_2" {
              # "Wrong"
              # "Reward"
              # "Trial"
              # "Tdelay"
              # "Prob"
              # "Block"
              # "OnOff"
              # "Trial"
              # "Tdelay"
              # "Prob"
              # "OnOff"
              # "Block"
              n202 = call "myRIO_BRig_RT_dataLC_Reward_Block.vi"() -> ("output_Reward_Block"=w381:i32)  [unwired: 11 in]
              n203 = call "myRIO_BRig_RT_dataLC_Reward_OnOff.vi"() -> ("output_Reward_OnOff"=w379:i32)  [unwired: 11 in]
              n204 = call "myRIO_BRig_RT_dataLC_Reward_Trial.vi"() -> ("output_Reward_Trial"=w376:i32)  [unwired: 11 in]
              n205 = call "myRIO_BRig_RT_dataLC_Wrong_Block.vi"() -> ("output_Wrong_Block"=w372:i32)  [unwired: 11 in]
              n206 = call "myRIO_BRig_RT_dataLC_Wrong_OnOff.vi"() -> ("output_Wrong_OnOff"=w371:i32)  [unwired: 11 in]
              n207 = call "myRIO_BRig_RT_dataLC_Wrong_Trial.vi"() -> ("output_Wrong_Trial"=w373:i32)  [unwired: 11 in]
              n208 = call "myRIO_BRig_RT_dataLC_Reward_Probability.vi"() -> ("output_Reward_Probability"=w378:i32)  [unwired: 11 in]
              n209 = call "myRIO_BRig_RT_dataLC_Reward_Tdelay.vi"() -> ("output_Reward_Tdelay"=w377:i32)  [unwired: 11 in]
              n210 = call "myRIO_BRig_RT_dataLC_Wrong_Probability.vi"() -> ("output_Wrong_Probability"=w375:i32)  [unwired: 11 in]
              n211 = call "myRIO_BRig_RT_dataLC_Wrong_Tdelay.vi"() -> ("output_Wrong_Tdelay"=w374:i32)  [unwired: 11 in]
              n212 = Index Array(array=w355, index #1=w381, index #2=w379, index #3=w378, index #4=w377, index #5=w376, index #6=w372, index #7=w371, index #8=w375, index #9=w374, index #10=w373) -> (element #1=w380:u16, element #2=w369:u16, element #3=w368:u16, element #4=w367:u16, element #5=w366:u16, element #6=w364:u16, element #7=w363:u16, element #8=w362:u16, element #9=w361:u16, element #10=w360:u16)
              n213 = Not Equal To 0?(x=w369) -> (x != 0?=w370:bool)
              n214 = Not Equal To 0?(x=w363) -> (x != 0?=w365:bool)
              n215 = local write "LC_Reward_Probability"(w368) -> ()
              n216 = local write "LC_Wrong_Probability"(w362) -> ()
              n217 = local write "LC_Reward_Tdelay"(w367) -> ()
              n218 = local write "LC_Reward_OnOff"(w370) -> ()
              n219 = local write "LC_Reward_Block"(w380) -> ()
              n220 = local write "LC_Reward_Trial"(w366) -> ()
              n221 = local write "LC_Wrong_Tdelay"(w361) -> ()
              n222 = local write "LC_Wrong_OnOff"(w365) -> ()
              n223 = local write "LC_Wrong_Block"(w364) -> ()
              n224 = local write "LC_Wrong_Trial"(w360) -> ()
            }
            frame "UploadSettings_dataMTrig_1" {
              # "Tdelay_R"
              # "Tdelay_L"
              # "Tcycle_R"
              # "Tcycle_L"
              # "RewCalib_nCycle_R"
              # "RewCalib_nCycle_L"
              # "Solenoid"
              # "Laser_Tcycle"
              n225 = call "myRIO_BRig_RT_dataMTrig_Laser_Tcycle.vi"() -> ("output_Laser_Tcycle"=w391:i32)  [unwired: 11 in]
              n226 = call "myRIO_BRig_RT_dataMTrig_Solenoid_RewCalib_nCycle__L.vi"() -> ("output_Solenoid_RewCalib_nCycle__L"=w390:i32)  [unwired: 11 in]
              n227 = call "myRIO_BRig_RT_dataMTrig_Solenoid_RewCalib_nCycle__R.vi"() -> ("output_Solenoid_RewCalib_nCycle__R"=w389:i32)  [unwired: 11 in]
              n228 = call "myRIO_BRig_RT_dataMTrig_Solenoid_Tdelay__L.vi"() -> ("output_Solenoid_Tdelay__L"=w386:i32)  [unwired: 11 in]
              n229 = call "myRIO_BRig_RT_dataMTrig_Solenoid_Tdelay__R.vi"() -> ("output_Solenoid_Tdelay__R"=w385:i32)  [unwired: 11 in]
              n230 = call "myRIO_BRig_RT_dataMTrig_Solenoid_Tcycle__L.vi"() -> ("output_Solenoid_Tcycle__L"=w388:i32)  [unwired: 11 in]
              n231 = call "myRIO_BRig_RT_dataMTrig_Solenoid_Tcycle__R.vi"() -> ("output_Solenoid_Tcycle__R"=w387:i32)  [unwired: 11 in]
              n232 = Index Array(array=w384, index #1=w391, index #2=w390, index #3=w389, index #4=w388, index #5=w387, index #6=w386, index #7=w385) -> (element #1=w398:u16, element #2=w397:u16, element #3=w396:u16, element #4=w395:u16, element #5=w394:u16, element #6=w393:u16, element #7=w392:u16)
              n233 = Replace Array Subset(array=w404, new element #1=w398, index #1=w391, new element #2=w397, index #2=w390, new element #3=w396, index #3=w389, new element #4=w395, index #4=w388, new element #5=w394, index #5=w387, new element #6=w393, index #6=w386, new element #7=w392, index #7=w385) -> (w403:u16[])
              n234 = local write "MTrig_Solenoid_Tcycle__L"(w395) -> ()
              n235 = local write "MTrig_Solenoid_Tcycle__R"(w394) -> ()
              n236 = local write "MTrig_Laser_Tcycle"(w398) -> ()
            }
            frame "Idle" {
              w424 = u16 1000 ("y")
              # "To ensure timing, we split the\nidle state into 4 phases"
              # "Laser_Tcycle"
              # "Audio_Tcycle_R"
              # "Audio_Tcycle_L"
              n237 = local read "MTrig_Audio_trig__L"() -> (w413:bool)
              n238 = local read "MTrig_Audio_trig__R"() -> (w415:bool)
              n239 = Select(t=myRIO_BRig_RT__Case_NonExp_stateList."SendData" ("Enum"), s="SendData", f=myRIO_BRig_RT__Case_NonExp_stateList."Idle_2" ("Enum")) -> (s? t:f=w408:T1)
              n240 = local read "MTrig_Laser_trig"() -> (w414:bool)
              n241 = call "myRIO_BRig_RT_dataMTrig_Audio_Tcycle__L.vi"() -> ("output_Audio_Tcycle__L"=w431:i32)  [unwired: 11 in]
              n242 = call "myRIO_BRig_RT_dataMTrig_Audio_Tcycle__R.vi"() -> ("output_Audio_Tcycle__R"=w430:i32)  [unwired: 11 in]
              n243 = call "myRIO_BRig_RT_dataMTrig_Laser_Tcycle.vi"() -> ("output_Laser_Tcycle"=w429:i32)  [unwired: 11 in]
              n244 = local read "MTrig_Laser_Tcycle"() -> (w406:u16)
              n245 = Select(t=myRIO_BRig_RT__Case_NonExp_stateList."TestConnection" ("Enum"), s="TestConnection", f=w408) -> (s? t:f=w417:T1)
              n246 = local read "Tcycle_Cue_min"() -> (w407:u16)
              n247 = Compound Arithmetic op=OR(w413, w415, w414) -> (w416:bool)
              n248 = case shown="True" w416 {
                frame False {
                }
                frame True {
                  w432 = FALSE
                  n249 = local write "MTrig_Audio_trig__L"(w432) -> ()
                  n250 = local write "MTrig_Audio_trig__R"(w432) -> ()
                  n251 = local write "MTrig_Laser_trig"(w432) -> ()
                }
              }
              n252 = Replace Array Subset(array=w427, new element #1=w407, index #1=w431, new element #2=w407, index #2=w430, new element #3=w406, index #3=w429) -> (w428:u16[])
              n253 = local read "Audio_Amp__R"() -> (w420:u16)
              n254 = local read "Audio_Amp__L"() -> (w421:u16)
              n255 = local read "Audio_Freq__R"() -> (w418:u16)
              n256 = local read "Audio_Freq__L"() -> (w419:u16)
              n257 = Multiply(x=w418, y=w424) -> (x*y=w422:u16)
              n258 = Multiply(x=w419, y=w424) -> (x*y=w423:u16)
            }
            frame "Idle_2" {
              # "To ensure timing, we split the\nidle state into 4 phases"
              # "Ncycles"
              # "Ncycles"
              # "RewCalib"
              # "RewCalib"
              # "Solenoid R"
              # "Solenoid L"
              n259 = call "myRIO_BRig_RT_dataMTrig_Solenoid_RewCalib_OnOff__L.vi"() -> ("output_Solenoid_RewCalib_OnOff__L"=w462:i32)  [unwired: 11 in]
              n260 = call "myRIO_BRig_RT_dataMTrig_Solenoid_N__L.vi"() -> ("output_Solenoid_N__L"=w450:i32)  [unwired: 11 in]
              n261 = call "myRIO_BRig_RT_dataMTrig_Solenoid_RewCalib_OnOff__R.vi"() -> ("output_Solenoid_RewCalib_OnOff__R"=w447:i32)  [unwired: 11 in]
              n262 = call "myRIO_BRig_RT_dataMTrig_Solenoid_N__R.vi"() -> ("output_Solenoid_N__R"=w446:i32)  [unwired: 11 in]
              n263 = Index Array(array=w453, index #1=w462, index #2=w450, index #3=w447, index #4=w446) -> (element #1=w449:u16, element #2=w444:u16, element #3=w445:u16, element #4=w443:u16)
              n264 = local read "RewCalib_Trig_L"() -> (w442:bool)
              n265 = local read "RewCalib_Trig_R"() -> (w441:bool)
              n266 = Equal To 0?(x=w444) -> (x = 0?=w452:bool)
              n267 = Equal To 0?(x=w443) -> (x = 0?=w451:bool)
              n268 = Not Equal To 0?(x=w445) -> (x != 0?=w463:bool)
              n269 = Not Equal To 0?(x=w449) -> (x != 0?=w464:bool)
              n270 = And(x=w452, y=w451) -> (x .and. y?=w456:bool)
              n271 = Or(x=w442, y=w441) -> (x .or. y?=w457:bool)
              n272 = Not Exclusive Or(1:w464, 2:w442) -> (0:w459:bool)
              n273 = Not Exclusive Or(1:w463, 2:w441) -> (0:w461:bool)
              n274 = And(x=w457, y=w456) -> (x .and. y?=w439:bool)
              n275 = Not(x=w459) -> (.not. x?=w458:bool)
              n276 = Not(x=w461) -> (.not. x?=w460:bool)
              n277 = Or(x=w458, y=w460) -> (x .or. y?=w440:bool)
              n278 = Or(x=w439, y=w440) -> (x .or. y?=w455:bool)
              n279 = Select(t=myRIO_BRig_RT__Case_NonExp_stateList."RewardCalibration_pre" ("Enum"), s=w455, f=myRIO_BRig_RT__Case_NonExp_stateList."Idle_3" ("Enum")) -> (s? t:f=w438:T1)
            }
            frame "Idle_3" {
              w487 = u8 0 ("f")
              # "To ensure timing, we split the\nidle state into 4 phases"
              n280 = local read "MTrig_Solenoid_trig__L"() -> (w473:bool)
              n281 = local read "MTrig_Solenoid_trig__R"() -> (w488:bool)
              n282 = local read "warmupType"() -> (w479:bool)
              n283 = local read "warmup"() -> (w480:bool)
              n284 = Not(x=w479) -> (.not. x?=w481:bool)
              n285 = Select(t=u8 1, s=w473, f=w487) -> (s? t:f=w486:u8)
              n286 = Select(t=u8 2, s=w488, f=w487) -> (s? t:f=w485:u8)
              n287 = And(x=w480, y=w481) -> (x .and. y?=w478:bool)
              n288 = And(x=w480, y=w479) -> (x .and. y?=w468:bool)
              n289 = Add(x=w486, y=w485) -> (x+y=w484:u8)
              n290 = case shown="3" w484 {
                tunnel: w483 -> [w491 w495 w513 w531]
                tunnel: [w491 w494 w512 w530] -> w482
                tunnel: w478 -> [_ w493 w511 w529]
                tunnel: [_ TRUE TRUE TRUE] -> w470
                frame 0, Default {
                }
                frame 1 {
                  n291 = case shown="True" w493 {
                    tunnel: w495 -> [w504 w509]
                    tunnel: [w503 w508] -> w494
                    frame True {
                      # "Audio_L"
                      # "Solenoid_L"
                      n292 = call "myRIO_BRig_RT_dataMTrig_Solenoid_N__L.vi"() -> ("output_Solenoid_N__L"=w500:i32)  [unwired: 11 in]
                      n293 = call "myRIO_BRig_RT_dataMTrig_Audio_N__L.vi"() -> ("output_Audio_N__L"=w498:i32)  [unwired: 11 in]
                      n294 = Index Array(array=w504, index #1=w500, index #2=w498) -> (element #1=w502:u16, element #2=w501:u16)
                      n295 = Increment(x=w502) -> (x+1=w499:u16)
                      n296 = Increment(x=w501) -> (x+1=w497:u16)
                      n297 = Replace Array Subset(array=w504, new element #1=w499, index #1=w500, new element #2=w497, index #2=w498) -> (w503:u16[])
                    }
                    frame False {
                      # "Solenoid_L"
                      n298 = call "myRIO_BRig_RT_dataMTrig_Solenoid_N__L.vi"() -> ("output_Solenoid_N__L"=w506:i32)  [unwired: 11 in]
                      n299 = Index Array(array=w509, index=w506) -> (element=w507:u16)
                      n300 = Increment(x=w507) -> (x+1=w505:u16)
                      n301 = Replace Array Subset(array=w509, new element=w505, index=w506) -> (w508:u16[])
                    }
                  }
                  n302 = local write "MTrig_Solenoid_trig__L"(FALSE) -> ()
                }
                frame 2 {
                  n303 = case shown="True" w511 {
                    tunnel: w513 -> [w522 w527]
                    tunnel: [w521 w526] -> w512
                    frame True {
                      # "Audio_R"
                      # "Solenoid_R"
                      n304 = call "myRIO_BRig_RT_dataMTrig_Solenoid_N__R.vi"() -> ("output_Solenoid_N__R"=w518:i32)  [unwired: 11 in]
                      n305 = call "myRIO_BRig_RT_dataMTrig_Audio_N__R.vi"() -> ("output_Audio_N__R"=w517:i32)  [unwired: 11 in]
                      n306 = Index Array(array=w522, index #1=w518, index #2=w517) -> (element #1=w520:u16, element #2=w519:u16)
                      n307 = Increment(x=w519) -> (x+1=w515:u16)
                      n308 = Increment(x=w520) -> (x+1=w516:u16)
                      n309 = Replace Array Subset(array=w522, new element #1=w516, index #1=w518, new element #2=w515, index #2=w517) -> (w521:u16[])
                    }
                    frame False {
                      # "Solenoid_R"
                      n310 = call "myRIO_BRig_RT_dataMTrig_Solenoid_N__R.vi"() -> ("output_Solenoid_N__R"=w523:i32)  [unwired: 11 in]
                      n311 = Index Array(array=w527, index=w523) -> (element=w525:u16)
                      n312 = Increment(x=w525) -> (x+1=w524:u16)
                      n313 = Replace Array Subset(array=w527, new element=w524, index=w523) -> (w526:u16[])
                    }
                  }
                  n314 = local write "MTrig_Solenoid_trig__R"(FALSE) -> ()
                }
                frame 3 {
                  w532 = FALSE
                  n315 = case shown="True" w529 {
                    tunnel: w531 -> [w546 w554]
                    tunnel: [w545 w553] -> w530
                    frame True {
                      # "Audio_R"
                      # "Solenoid_R"
                      # "Audio_L"
                      # "Solenoid_L"
                      n316 = call "myRIO_BRig_RT_dataMTrig_Solenoid_N__L.vi"() -> ("output_Solenoid_N__L"=w540:i32)  [unwired: 11 in]
                      n317 = call "myRIO_BRig_RT_dataMTrig_Audio_N__L.vi"() -> ("output_Audio_N__L"=w538:i32)  [unwired: 11 in]
                      n318 = call "myRIO_BRig_RT_dataMTrig_Solenoid_N__R.vi"() -> ("output_Solenoid_N__R"=w536:i32)  [unwired: 11 in]
                      n319 = call "myRIO_BRig_RT_dataMTrig_Audio_N__R.vi"() -> ("output_Audio_N__R"=w535:i32)  [unwired: 11 in]
                      n320 = Index Array(array=w546, index #1=w540, index #2=w538, index #3=w536, index #4=w535) -> (element #1=w544:u16, element #2=w543:u16, element #3=w542:u16, element #4=w541:u16)
                      n321 = Increment(x=w541) -> (x+1=w533:u16)
                      n322 = Increment(x=w544) -> (x+1=w539:u16)
                      n323 = Increment(x=w543) -> (x+1=w537:u16)
                      n324 = Increment(x=w542) -> (x+1=w534:u16)
                      n325 = Replace Array Subset(array=w546, new element #1=w539, index #1=w540, new element #2=w537, index #2=w538, new element #3=w534, index #3=w536, new element #4=w533, index #4=w535) -> (w545:u16[])
                    }
                    frame False {
                      # "Solenoid_R"
                      # "Solenoid_L"
                      n326 = call "myRIO_BRig_RT_dataMTrig_Solenoid_N__L.vi"() -> ("output_Solenoid_N__L"=w550:i32)  [unwired: 11 in]
                      n327 = call "myRIO_BRig_RT_dataMTrig_Solenoid_N__R.vi"() -> ("output_Solenoid_N__R"=w547:i32)  [unwired: 11 in]
                      n328 = Index Array(array=w554, index #1=w550, index #2=w547) -> (element #1=w552:u16, element #2=w551:u16)
                      n329 = Increment(x=w552) -> (x+1=w549:u16)
                      n330 = Increment(x=w551) -> (x+1=w548:u16)
                      n331 = Replace Array Subset(array=w554, new element #1=w549, index #1=w550, new element #2=w548, index #2=w547) -> (w553:u16[])
                    }
                  }
                  n332 = local write "MTrig_Solenoid_trig__L"(w532) -> ()
                  n333 = local write "MTrig_Solenoid_trig__R"(w532) -> ()
                }
              }
              n334 = Select(t=myRIO_BRig_RT__Case_NonExp_stateList."Cue_pre", s=w468, f=myRIO_BRig_RT__Case_NonExp_stateList."DispenseWater_pre" ("Enum")) -> (s? t:f=w466:T1)
              n335 = Select(t=w466, s=w470, f=myRIO_BRig_RT__Case_NonExp_stateList."Idle_4" ("Enum")) -> (s? t:f=w471:T1)
            }
            frame "Idle_4" {
              # "use dataMTrig as it is one of the last to transfer"
              # "To ensure timing, we split the\nidle state into 4 phases"
              n336 = call "myRIO_BRig_RT_comm_webdav_uploadReceived_check_v2,0.vi"("input_dataName"="dataMTrig") -> ("output_Iexist"=w564:bool)  [unwired: 9 in, 1 out]
              n337 = Select(t=myRIO_BRig_RT__Case_NonExp_stateList."UploadSettings_pre" ("Enum"), s=w564, f=myRIO_BRig_RT__Case_NonExp_stateList."Idle") -> (s? t:f=w562:T1)
            }
            frame "Cue_pre" {
              w572 = u16 1 ("t")
              w571 = u16 0 ("new element/subarray")
              w568 = u16 0 ("new element/subarray")
              # "Ncycle"
              # "count"
              # "Audio_R"
              # "Solenoid_R"
              # "Solenoid_L"
              # "Ncycle"
              # "count"
              # "Audio_L"
              n338 = call "myRIO_BRig_RT_dataMTrig_Solenoid_N__L.vi"() -> ("output_Solenoid_N__L"=w583:i32)  [unwired: 11 in]
              n339 = call "myRIO_BRig_RT_dataMTrig_Solenoid_N__R.vi"() -> ("output_Solenoid_N__R"=w582:i32)  [unwired: 11 in]
              n340 = Index Array(array=w579, index #1=w583, index #2=w582) -> (element #1=w581:u16, element #2=w580:u16)
              n341 = Not Equal To 0?(x=w580) -> (x != 0?=w573:bool)
              n342 = Not Equal To 0?(x=w581) -> (x != 0?=w575:bool)
              n343 = Select(t=w572, s=w575, f=w571) -> (s? t:f=w574:u16)
              n344 = Select(t=w572, s=w573, f=w571) -> (s? t:f=w567:u16)
              n345 = call "myRIO_BRig_RT_dataMTrig_Audio_c__L.vi"() -> ("output_Audio_c__L"=w577:i32)  [unwired: 11 in]
              n346 = call "myRIO_BRig_RT_dataMTrig_Audio_N__L.vi"() -> ("output_Audio_N__L"=w576:i32)  [unwired: 11 in]
              n347 = call "myRIO_BRig_RT_dataMTrig_Audio_c__R.vi"() -> ("output_Audio_c__R"=w570:i32)  [unwired: 11 in]
              n348 = call "myRIO_BRig_RT_dataMTrig_Audio_N__R.vi"() -> ("output_Audio_N__R"=w569:i32)  [unwired: 11 in]
              n349 = Replace Array Subset(array=w579, new element #1=w568, index #1=w577, new element #2=w574, index #2=w576, new element #3=w568, index #3=w570, new element #4=w567, index #4=w569) -> (w578:u16[])
            }
            frame "Cue" {
              # "Ncycle"
              # "Audio_R"
              # "Ncycle"
              # "Audio_L"
              n350 = call "myRIO_BRig_RT_dataMTrig_Audio_N__L.vi"() -> ("output_Audio_N__L"=w599:i32)  [unwired: 11 in]
              n351 = call "myRIO_BRig_RT_dataMTrig_Audio_N__R.vi"() -> ("output_Audio_N__R"=w598:i32)  [unwired: 11 in]
              n352 = Index Array(array=w604, index #1=w599, index #2=w598) -> (element #1=w597:u16, element #2=w596:u16)
              n353 = Equal To 0?(x=w597) -> (x = 0?=w595:bool)
              n354 = Equal To 0?(x=w596) -> (x = 0?=w594:bool)
              n355 = And(x=w595, y=w594) -> (x .and. y?=w593:bool)
              n356 = Select(t=myRIO_BRig_RT__Case_NonExp_stateList."DispenseWater_pre", s=w593, f=w591) -> (s? t:f=w590:T1)
            }
            frame "RewardCalibration_pre" {
              (unwired) FALSE
              w610 = FALSE
              w621 = u8 0
              w637 = u8 0
              # "Are we starting a RewardCalibration?\nOr are we stopping a RewardCalibration?\nOr is a RewardCalibration over?"
              # "RewCalib\nOnOff"
              # "N"
              # "Solenoid R"
              # "RewCalib\nOnOff"
              # "N"
              # "Solenoid L"
              n357 = local read "RewCalib_Trig_L"() -> (w644:bool)
              n358 = local read "RewCalib_Trig_R"() -> (w613:bool)
              n359 = call "myRIO_BRig_RT_dataMTrig_Solenoid_N__R.vi"() -> ("output_Solenoid_N__R"=w615:i32)  [unwired: 11 in]
              n360 = call "myRIO_BRig_RT_dataMTrig_Solenoid_RewCalib_OnOff__R.vi"() -> ("output_Solenoid_RewCalib_OnOff__R"=w612:i32)  [unwired: 11 in]
              n361 = call "myRIO_BRig_RT_dataMTrig_Solenoid_N__L.vi"() -> ("output_Solenoid_N__L"=w630:i32)  [unwired: 11 in]
              n362 = call "myRIO_BRig_RT_dataMTrig_Solenoid_RewCalib_OnOff__L.vi"() -> ("output_Solenoid_RewCalib_OnOff__L"=w631:i32)  [unwired: 11 in]
              n363 = Index Array(array=w614, index #1=w615, index #2=w612) -> (element #1=w625:u16, element #2=w620:u16)
              n364 = Index Array(array=w614, index #1=w630, index #2=w631) -> (element #1=w641:u16, element #2=w636:u16)
              n365 = Equal To 0?(x=w625) -> (x = 0?=w626:bool)
              n366 = Not Equal To 0?(x=w620) -> (x != 0?=w623:bool)
              n367 = Equal To 0?(x=w641) -> (x = 0?=w642:bool)
              n368 = Not Equal To 0?(x=w636) -> (x != 0?=w639:bool)
              n369 = local write "MTrig_Solenoid_trig__L"(w610) -> ()
              n370 = local write "MTrig_Solenoid_trig__R"(w610) -> ()
              n371 = Select(t=u8 1, s=w613, f=w621) -> (s? t:f=w617:u8)
              n372 = Select(t=u8 1, s=w644, f=w637) -> (s? t:f=w633:u8)
              n373 = Select(t=u8 2, s=w626, f=w621) -> (s? t:f=w618:u8)
              n374 = Select(t=u8 4, s=w623, f=w621) -> (s? t:f=w619:u8)
              n375 = Select(t=u8 2, s=w642, f=w637) -> (s? t:f=w634:u8)
              n376 = Select(t=u8 4, s=w639, f=w637) -> (s? t:f=w635:u8)
              n377 = Compound Arithmetic op=ADD(w617, w618, w619) -> (w616:u8)
              n378 = Compound Arithmetic op=ADD(w633, w634, w635) -> (w632:u8)
              n379 = case shown="7" w632 {
                tunnel: w614 -> [w674 w679 w681 w686 w691 w693 w696 w701]
                tunnel: [w674 w680 w681 w687 w692 w693 w697 w702] -> w629
                tunnel: w631 -> [_ w677 _ w684 w689 _ w695 w700]
                tunnel: w630 -> [_ w678 _ w685 w690 _ _ _]
                frame 0, Default {
                }
                frame 1 {
                  n380 = Replace Array Subset(array=w679, new element #1=u16 100 ("new element/subarray"), index #1=w678, new element #2=u16 1 ("new element/subarray"), index #2=w677) -> (w680:u16[])
                }
                frame 2 {
                }
                frame 3 {
                  n381 = Replace Array Subset(array=w686, new element #1=u16 100 ("new element/subarray"), index #1=w685, new element #2=u16 1 ("new element/subarray"), index #2=w684) -> (w687:u16[])
                }
                frame 4 {
                  w688 = u16 0 ("new element/subarray")
                  n382 = Replace Array Subset(array=w691, new element #1=w688, index #1=w690, new element #2=w688, index #2=w689) -> (w692:u16[])
                }
                frame 5 {
                }
                frame 6 {
                  n383 = Replace Array Subset(array=w696, new element=u16 0 ("new element/subarray"), index=w695) -> (w697:u16[])
                }
                frame 7 {
                  n384 = local write "RewCalib_Trig_L"(FALSE ("RewCalib_Trig_L")) -> ()
                  n385 = Replace Array Subset(array=w701, new element=u16 0 ("new element/subarray"), index=w700) -> (w702:u16[])
                }
              }
              n386 = case shown="7" w616 {
                tunnel: w629 -> [w645 w650 w652 w657 w662 w664 w667 w672]
                tunnel: [w645 w651 w652 w658 w663 w664 w668 w673] -> w628
                tunnel: w612 -> [_ w648 _ w655 w660 _ w666 w671]
                tunnel: w615 -> [_ w649 _ w656 w661 _ _ _]
                frame 0, Default {
                }
                frame 1 {
                  n387 = Replace Array Subset(array=w650, new element #1=u16 100 ("new element/subarray"), index #1=w649, new element #2=u16 1 ("new element/subarray"), index #2=w648) -> (w651:u16[])
                }
                frame 2 {
                }
                frame 3 {
                  n388 = Replace Array Subset(array=w657, new element #1=u16 100 ("new element/subarray"), index #1=w656, new element #2=u16 1 ("new element/subarray"), index #2=w655) -> (w658:u16[])
                }
                frame 4 {
                  w659 = u16 0 ("new element/subarray")
                  n389 = Replace Array Subset(array=w662, new element #1=w659, index #1=w661, new element #2=w659, index #2=w660) -> (w663:u16[])
                }
                frame 5 {
                }
                frame 6 {
                  n390 = Replace Array Subset(array=w667, new element=u16 0 ("new element/subarray"), index=w666) -> (w668:u16[])
                }
                frame 7 {
                  n391 = local write "RewCalib_Trig_R"(FALSE ("RewCalib_Trig_L")) -> ()
                  n392 = Replace Array Subset(array=w672, new element=u16 0 ("new element/subarray"), index=w671) -> (w673:u16[])
                }
              }
            }
            frame "DispenseWater_pre" {
              w709 = u16 0 ("t")
              w752 = u16 0 ("new element/subarray")
              # "just trust me on this one"
              # "RewCalib\nOnOff"
              # "RewCalib\nOnOff"
              # "nCycle"
              # "Solenoid__R"
              # "Tdelay"
              # "delay"
              # "nCycle"
              # "Solenoid__L"
              # "Tdelay"
              # "delay"
              # "Solenoid__R"
              # "count"
              # "Solenoid_Tcycle_R"
              # "Solenoid_Tcycle_L"
              # "Solenoid__L"
              # "count"
              n393 = call "myRIO_BRig_RT_dataMTrig_Solenoid_RewCalib_OnOff__L.vi"() -> ("output_Solenoid_RewCalib_OnOff__L"=w716:i32)  [unwired: 11 in]
              n394 = call "myRIO_BRig_RT_dataMTrig_Solenoid_N__L.vi"() -> ("output_Solenoid_N__L"=w707:i32)  [unwired: 11 in]
              n395 = call "myRIO_BRig_RT_dataMTrig_Solenoid_delay__L.vi"() -> ("output_Solenoid_delay__L"=w750:i32)  [unwired: 11 in]
              n396 = call "myRIO_BRig_RT_dataMTrig_Solenoid_Tdelay__L.vi"() -> ("output_Solenoid_Tdelay__L"=w749:i32)  [unwired: 11 in]
              n397 = call "myRIO_BRig_RT_dataMTrig_Solenoid_N__R.vi"() -> ("output_Solenoid_N__R"=w705:i32)  [unwired: 11 in]
              n398 = call "myRIO_BRig_RT_dataMTrig_Solenoid_delay__R.vi"() -> ("output_Solenoid_delay__R"=w739:i32)  [unwired: 11 in]
              n399 = call "myRIO_BRig_RT_dataMTrig_Solenoid_Tdelay__R.vi"() -> ("output_Solenoid_Tdelay__R"=w738:i32)  [unwired: 11 in]
              n400 = call "myRIO_BRig_RT_dataMTrig_Solenoid_RewCalib_OnOff__R.vi"() -> ("output_Solenoid_RewCalib_OnOff__R"=w712:i32)  [unwired: 11 in]
              n401 = Index Array(array=w751, index #1=w707, index #2=w750, index #3=w749, index #4=w705, index #5=w739, index #6=w738, index #7=w716, index #8=w712) -> (element #1=w708:u16, element #2=w748:u16, element #3=w743:u16, element #4=w711:u16, element #5=w733:u16, element #6=w732:u16, element #7=w717:u16, element #8=w714:u16)
              n402 = Equal To 0?(x=w748) -> (x = 0?=w747:bool)
              n403 = Equal To 0?(x=w733) -> (x = 0?=w737:bool)
              n404 = local read "RewCalib_Trig_L"() -> (w728:bool)
              n405 = local read "RewCalib_Trig_R"() -> (w723:bool)
              n406 = Not Equal To 0?(x=w708) -> (x != 0?=w746:bool)
              n407 = Not Equal To 0?(x=w711) -> (x != 0?=w736:bool)
              n408 = local read "MTrig_Solenoid_Tcycle__L"() -> (w745:u16)
              n409 = local read "MTrig_Solenoid_Tcycle__R"() -> (w731:u16)
              n410 = Not Equal To 0?(x=w717) -> (x != 0?=w727:bool)
              n411 = Not Equal To 0?(x=w714) -> (x != 0?=w725:bool)
              n412 = Not(x=w728) -> (.not. x?=w726:bool)
              n413 = Not(x=w723) -> (.not. x?=w724:bool)
              n414 = And(x=w727, y=w726) -> (x .and. y?=w722:bool)
              n415 = And(x=w725, y=w724) -> (x .and. y?=w721:bool)
              n416 = call "myRIO_BRig_RT_dataMTrig_Solenoid_c__L.vi"() -> ("output_Solenoid_c__L"=w754:i32)  [unwired: 11 in]
              n417 = call "myRIO_BRig_RT_dataMTrig_Solenoid_c__R.vi"() -> ("output_Solenoid_c__R"=w753:i32)  [unwired: 11 in]
              n418 = Select(t=w745, s=w746, f=u16 0) -> (s? t:f=w742:u16)
              n419 = Or(x=w722, y=w721) -> (x .or. y?=w710:bool)
              n420 = Select(t=w731, s=w736, f=u16 0) -> (s? t:f=w734:u16)
              n421 = Select(t=w742, s=w747, f=w743) -> (s? t:f=w740:u16)
              n422 = Select(t=w734, s=w737, f=w732) -> (s? t:f=w729:u16)
              n423 = call "myRIO_BRig_RT_dataMTrig_Solenoid_Tcycle__L.vi"() -> ("output_Solenoid_Tcycle__L"=w741:i32)  [unwired: 11 in]
              n424 = call "myRIO_BRig_RT_dataMTrig_Solenoid_Tcycle__R.vi"() -> ("output_Solenoid_Tcycle__R"=w730:i32)  [unwired: 11 in]
              n425 = Select(t=w709, s=w710, f=w708) -> (s? t:f=w706:u16)
              n426 = Select(t=w709, s=w710, f=w711) -> (s? t:f=w704:u16)
              n427 = Select(t=myRIO_BRig_RT__Case_NonExp_stateList."Idle" ("Enum"), s=w710, f=myRIO_BRig_RT__Case_NonExp_stateList."DispenseWater" ("Enum")) -> (s? t:f=w718:T1)
              n428 = Select(t=w709, s=w710, f=w717) -> (s? t:f=w715:u16)
              n429 = Select(t=w709, s=w710, f=w714) -> (s? t:f=w713:u16)
              n430 = Replace Array Subset(array=w751, new element #1=w752, index #1=w754, new element #2=w752, index #2=w753, new element #3=w740, index #3=w741, new element #4=w729, index #4=w730, new element #5=w715, index #5=w716, new element #6=w713, index #6=w712, new element #7=w706, index #7=w707, new element #8=w704, index #8=w705) -> (w755:u16[])
            }
            frame "DispenseWater" {
              # "D"
              # "C"
              # "B"
              # "A"
              # "(A) Add COUNT and INCREMENT\n(B) Is (A) smaller than Tcycle?\n(C) Are we dispensing water or in the delay phase?\n(D) If (A) is smaller than Tcycle   AND   if we are dispensing water\n      then send TRUE to solenoid"
              # "delay"
              # "Tcycle"
              # "Solenoid__R"
              # "count"
              # "delay"
              # "Tcycle"
              # "Solenoid__L"
              # "count"
              n431 = To Unsigned Word Integer(number=w786) -> (unsigned 16bit integer=w768:u16)
              n432 = call "myRIO_BRig_RT_dataMTrig_Solenoid_delay__R.vi"() -> ("output_Solenoid_delay__R"=w772:i32)  [unwired: 11 in]
              n433 = call "myRIO_BRig_RT_dataMTrig_Solenoid_c__R.vi"() -> ("output_Solenoid_c__R"=w771:i32)  [unwired: 11 in]
              n434 = call "myRIO_BRig_RT_dataMTrig_Solenoid_Tcycle__R.vi"() -> ("output_Solenoid_Tcycle__R"=w773:i32)  [unwired: 11 in]
              n435 = call "myRIO_BRig_RT_dataMTrig_Solenoid_delay__L.vi"() -> ("output_Solenoid_delay__L"=w788:i32)  [unwired: 11 in]
              n436 = call "myRIO_BRig_RT_dataMTrig_Solenoid_c__L.vi"() -> ("output_Solenoid_c__L"=w780:i32)  [unwired: 11 in]
              n437 = call "myRIO_BRig_RT_dataMTrig_Solenoid_Tcycle__L.vi"() -> ("output_Solenoid_Tcycle__L"=w789:i32)  [unwired: 11 in]
              n438 = Index Array(array=w782, index #1=w780, index #2=w789, index #3=w788, index #4=w771, index #5=w773, index #6=w772) -> (element #1=w787:u16, element #2=w777:u16, element #3=w785:u16, element #4=w767:u16, element #5=w764:u16, element #6=w763:u16)
              n439 = Add(x=w787, y=w768) -> (x+y=w778:u16)
              n440 = Add(x=w767, y=w768) -> (x+y=w769:u16)
              n441 = Less?(x=w778, y=w777) -> (x < y?=w761:bool)
              n442 = Equal To 0?(x=w785) -> (x = 0?=w784:bool)
              n443 = Less?(x=w769, y=w764) -> (x < y?=w762:bool)
              n444 = Equal To 0?(x=w763) -> (x = 0?=w770:bool)
              n445 = And(x=w761, y=w784) -> (x .and. y?=w783:bool)
              n446 = Or(x=w761, y=w762) -> (x .or. y?=w760:bool)
              n447 = And(x=w762, y=w770) -> (x .and. y?=w765:bool)
              n448 = Select(t=w778, s=w761, f=w777) -> (s? t:f=w779:u16)
              n449 = Select(t=w769, s=w762, f=w764) -> (s? t:f=w766:u16)
              n450 = Replace Array Subset(array=w782, new element #1=w779, index #1=w780, new element #2=w766, index #2=w771) -> (w781:u16[])
              n451 = Select(t=w776, s=w760, f=myRIO_BRig_RT__Case_NonExp_stateList."DispenseWater_post" ("Enum")) -> (s? t:f=w774:T1)
            }
            frame "DispenseWater_post" {
              # "nCycle"
              # "delay"
              # "Solenoid__R"
              # "nCycle"
              # "delay"
              # "Solenoid__L"
              n452 = call "myRIO_BRig_RT_dataMTrig_Solenoid_N__L.vi"() -> ("output_Solenoid_N__L"=w811:i32)  [unwired: 11 in]
              n453 = call "myRIO_BRig_RT_dataMTrig_Solenoid_delay__L.vi"() -> ("output_Solenoid_delay__L"=w810:i32)  [unwired: 11 in]
              n454 = call "myRIO_BRig_RT_dataMTrig_Solenoid_N__R.vi"() -> ("output_Solenoid_N__R"=w807:i32)  [unwired: 11 in]
              n455 = call "myRIO_BRig_RT_dataMTrig_Solenoid_delay__R.vi"() -> ("output_Solenoid_delay__R"=w806:i32)  [unwired: 11 in]
              n456 = Index Array(array=w813, index #1=w811, index #2=w810, index #3=w807, index #4=w806) -> (element #1=w815:u16, element #2=w814:u16, element #3=w798:u16, element #4=w800:u16)
              n457 = Not Equal To 0?(x=w815) -> (x != 0?=w816:bool)
              n458 = Not Equal To 0?(x=w798) -> (x != 0?=w799:bool)
              n459 = case shown="True" w799 {
                selector: w799 -> [_ w824]
                tunnel: w798 -> [w822 w830]
                tunnel: w800 -> [_ w831]
                tunnel: [w822 w828] -> w797
                tunnel: [u16 0 w827] -> w796
                tunnel: [_ w824] -> w795
                frame False {
                }
                frame True {
                  n460 = Equal To 0?(x=w831) -> (x = 0?=w823:bool)
                  n461 = Decrement(x=w830) -> (x-1=w829:u16)
                  n462 = Select(t=w829, s=w823, f=w830) -> (s? t:f=w828:u16)
                  n463 = Select(t=u16 1, s=w823, f=u16 0) -> (s? t:f=w827:u16)
                }
              }
              n464 = case shown="True" w816 {
                selector: w816 -> [_ w835]
                tunnel: w815 -> [w833 w841]
                tunnel: w814 -> [_ w842]
                tunnel: [w833 w839] -> w809
                tunnel: [u16 0 w838] -> w808
                tunnel: [_ w835] -> w805
                frame False {
                }
                frame True {
                  n465 = Equal To 0?(x=w842) -> (x = 0?=w834:bool)
                  n466 = Decrement(x=w841) -> (x-1=w840:u16)
                  n467 = Select(t=w840, s=w834, f=w841) -> (s? t:f=w839:u16)
                  n468 = Select(t=u16 1, s=w834, f=u16 0) -> (s? t:f=w838:u16)
                }
              }
              n469 = Or(x=w805, y=w795) -> (x .or. y?=w804:bool)
              n470 = Replace Array Subset(array=w813, new element #1=w809, index #1=w811, new element #2=w808, index #2=w810, new element #3=w797, index #3=w807, new element #4=w796, index #4=w806) -> (w812:u16[])
              n471 = Select(t=myRIO_BRig_RT__Case_NonExp_stateList."DispenseWater_pre" ("Enum"), s=w804, f=myRIO_BRig_RT__Case_NonExp_stateList."Idle" ("Enum")) -> (s? t:f=w801:T1)
            }
            frame "TestConnection" {
              n472 = local read "Host Password"() -> (w853:string)
              n473 = local read "Host UserName"() -> (w854:string)
              n474 = call "myRIO_BRig_RT_comm_webdav_testConnect.vi"("input_password"=w853, "input_username"=w854) -> ("output_Iconnected"=w851:bool)  [unwired: 9 in]
              n475 = Select(t="Connection accepted!" ("message"), s=w851, f="Error!") -> (s? t:f=w849:string)
              n476 = One Button Dialog(message=w849) -> ()  [unwired: 1 in, 1 out]
            }
            frame "SendData" {
              n477 = local read "Host Filename Prefix"() -> (w856:string)
              n478 = local read "Host Password"() -> (w857:string)
              n479 = local read "Host UserName"() -> (w858:string)
              n480 = call "myRIO_BRig_RT_comm_webdav_sendData_all.vi"("Host Filename Prefix"=w856, "Host Password"=w857, "Host UserName"=w858) -> ()  [unwired: 9 in]
            }
            frame "End" {
            }
          }
          n481 = local read "MTrig_Audio_trig__R"() -> (w76:bool)
          n482 = local read "MTrig_Audio_trig__L"() -> (w75:bool)
          n483 = local read "START"() -> (w71:bool)
          n484 = local read "STOP_abort"() -> (w70:bool)
          n485 = local read "MTrig_Laser_trig"() -> (w77:bool)
          n486 = call "myRIO_BRig_RT_dataMTrig_main__v2.vi"("input_dataMTrig"=w79, "input_Audio_trig_L"=w75, "input_Audio_trig_R"=w76, "input_Laser_trig"=w77) -> ("output_dataMTrig"=w78:u16[], "output_Audio_L"=w55:bool, "output_Audio_R"=w66:bool, "output_Laser"=w58:bool)  [unwired: 12 in]
          n487 = Or(x=w71, y=w70) -> (x .or. y?=w69:bool)
          n488 = Select(t=myRIO_BRig_RT__Case_NonExp_stateList."End" ("Enum"), s=w69, f=w68) -> (s? t:f=w67:T1)
          n489 = Or(x=w76, y=w77) -> (x .or. y?=w74:bool)
          n490 = Or(x=w74, y=w75) -> (x .or. y?=w73:bool)
          n491 = case shown="True" w73 {
            frame False {
            }
            frame True {
              w104 = FALSE
              n492 = local write "MTrig_Audio_trig__R"(w104) -> ()
              n493 = local write "MTrig_Audio_trig__L"(w104) -> ()
              n494 = local write "MTrig_Laser_trig"(w104) -> ()
            }
          }
          n495 = xnode "Read/Write Control"("FPGA VI Reference In"=w96, "error in"=w94, "A1_SR"=w80, "A3_SL"=w81, "audioTrigger_L"=w55, "audioAmp_L"=w85, "audioFreq_L_Hz"=w84, "audioTrigger_R"=w66, "audioAmp_R"=w83, "audioFreq_R_Hz"=w82, "laserResponse_reward_LED"="laserResponse_reward_LED", "laserResponse_wrong_LED"="laserResponse_wrong_LED", "laserResponse_reward"="laserResponse_reward", "laserResponse_wrong"="laserResponse_wrong", "SelectionState"="SelectionState", "ignoreWrong"="ignoreWrong", "Left(F)_or_Right(T)"="Left(F)_or_Right(T)", "laserMTrig"=w58) -> ("FPGA VI Reference Out"=w95:refnum<k20>, "error out"=w93:errorcluster, "SelectReward"=→"SelectReward":bool, "SelectWrong"=→"SelectWrong":bool)
          n496 = node-c288() -> ()  [unwired: 1 in, 1 out]
          "cState_NonExp" <- w92
        }
        n497 = node-c288(w48) -> ()  [unwired: 1 out]
        n498 = flat-sequence {
          tunnel: w41 -> [w52]
          tunnel: [w52] -> w40
          tunnel: w39 -> [w51]
          tunnel: [w51] -> w38
          frame #0 {
            w50 = FALSE
            n499 = local write "STOP_endBlock"(w50) -> ()
            n500 = local write "STOP_endTrial"(w50) -> ()
          }
        }
      }
      frame True {
        w880 = FALSE ("SelectionState")
        w885 = u16 0 ("idxDataBlock")
        w887 = u16 100 ("new element/subarray")
        w888 = u16 100 ("new element/subarray")
        w908 = T6 refnum items=["Session NI_WebDAV"] ("output_hSession")
        w917 = FALSE
        w918 = u16 0
        w879 = FALSE
        # "audio__L\naudio__R"
        # "Audio params"
        # "nRewards"
        # "idxDataBlock"
        # "Solenoid_Tdelay_R"
        # "Solenoid_Tdelay_L"
        # "RewCalib_N__R"
        # "RewCalib_N__L"
        # "Save dataLick to file\nSend file to Host\nSave dataMTrig\nSend file to Host\nDisconnect"
        # "dataTrial"
        # "dataTrial"
        # "Solenoid_Tcycle_R"
        # "Solenoid_Tcycle_L"
        # "Laser_Tcycle"
        # "Audio_Tcycle_R"
        # "Audio_Tcycle_L"
        # "dataLick"
        # "dataLC"
        # "dataLC"
        # "dataBlock"
        # "dataBlock"
        # "dataMTrig"
        # "dataMTrig"
        # "dataExp"
        # "dataCurrent"
        # "dataExp"
        # "dataCurrent"
        # "spout"
        # "state"
        n501 = call "myRIO_BRig_RT_dataMTrig_Solenoid_Tcycle__L.vi"() -> ("output_Solenoid_Tcycle__L"=w914:i32)  [unwired: 11 in]
        n502 = call "myRIO_BRig_RT_dataMTrig_Solenoid_Tcycle__R.vi"() -> ("output_Solenoid_Tcycle__R"=w913:i32)  [unwired: 11 in]
        n503 = call "myRIO_BRig_RT_dataMTrig_Audio_Tcycle__L.vi"() -> ("output_Audio_Tcycle__L"=w912:i32)  [unwired: 11 in]
        n504 = call "myRIO_BRig_RT_dataMTrig_Audio_Tcycle__R.vi"() -> ("output_Audio_Tcycle__R"=w911:i32)  [unwired: 11 in]
        n505 = call "myRIO_BRig_RT_dataMTrig_Laser_Tcycle.vi"() -> ("output_Laser_Tcycle"=w910:i32)  [unwired: 11 in]
        n506 = local read "MTrig_Solenoid_Tcycle__L"() -> (w893:u16)
        n507 = local read "MTrig_Solenoid_Tcycle__R"() -> (w892:u16)
        n508 = local read "Tcycle_Reward_L"() -> (w889:u16)
        n509 = local read "Tcycle_Reward_R"() -> (w890:u16)
        n510 = local read "MTrig_Laser_Tcycle"() -> (w891:u16)
        n511 = call "myRIO_BRig_RT_dataMTrig_Solenoid_RewCalib_nCycle__L.vi"() -> ("output_Solenoid_RewCalib_nCycle__L"=w896:i32)  [unwired: 11 in]
        n512 = call "myRIO_BRig_RT_dataMTrig_Solenoid_Tdelay__L.vi"() -> ("output_Solenoid_Tdelay__L"=w898:i32)  [unwired: 11 in]
        n513 = call "myRIO_BRig_RT_dataMTrig_Solenoid_RewCalib_nCycle__R.vi"() -> ("output_Solenoid_RewCalib_nCycle__R"=w897:i32)  [unwired: 11 in]
        n514 = call "myRIO_BRig_RT_dataMTrig_Solenoid_Tdelay__R.vi"() -> ("output_Solenoid_Tdelay__R"=w899:i32)  [unwired: 11 in]
        n515 = call "myRIO_BRig_RT_dataLick_init.vi"() -> ("output_dataLick"=w920:u16[][])  [unwired: 11 in]
        n516 = call "myRIO_BRig_RT_dataCurrent_init.vi"() -> ("output_dataCurrent"=w927:u16[])  [unwired: 11 in]
        n517 = call "myRIO_BRig_RT_dataExp_init.vi"() -> ("output_dataExp"=w926:u16[])  [unwired: 11 in]
        n518 = call "myRIO_BRig_RT_dataMTrig_init.vi"() -> ("output_dataMTrig"=w916:u16[])  [unwired: 5 in]
        n519 = call "myRIO_BRig_RT_dataLC_init.vi"() -> ("output_dataLC"=w924:u16[])  [unwired: 11 in]
        n520 = call "myRIO_BRig_RT_dataBlock_init.vi"() -> ("output_dataBlock"=w925:u16[][])  [unwired: 11 in]
        n521 = call "myRIO_BRig_RT_dataTrial_init.vi"() -> ("output_dataTrial"=w909:u16[][])  [unwired: 11 in]
        n522 = xnode "Read/Write Control"("FPGA VI Reference In"=w881, "error in"=w882, "SelectionState"=w880, "laserResponse_reward"=w880, "laserResponse_wrong"=w880, "laserResponse_reward_LED"=w880, "laserResponse_wrong_LED"=w880, "Left(F)_or_Right(T)"=w880, "ignoreWrong"=w880, "SelectionState"=w880) -> ("FPGA VI Reference Out"=w883:refnum<k20>, "error out"=w884:errorcluster)
        n523 = Replace Array Subset(array=w916, new element #1=w888, index #1=w896, new element #2=w888, index #2=w897, new element #3=w887, index #3=w898, new element #4=w887, index #4=w899, new element #5=w893, index #5=w914, new element #6=w892, index #6=w913, new element #7=w889, index #7=w912, new element #8=w890, index #8=w911, new element #9=w891, index #9=w910) -> (w915:u16[])
        n524 = Get Date/Time In Seconds() -> (seconds since 1Jan1904=w895:timestamp)
        n525 = To Double Precision Float(number=w895) -> (double precision float=w894:dbl)
        n526 = node-c288() -> (w935:T3)  [unwired: 4 in]
        n527 = timed-loop {
          timing: w935 -> [_]
          timing-out: [_] -> w934
          shift-right: [w1013] -> _
          shift-left: myRIO_BRig_RT__Case_Exp_stateList."Start1" ("Enum") -> [w1044]
          shift-right: [w1065] -> _
          shift-left: enum16{"Left", "Right"}."Left" -> [w1067]
          tunnel: w883 -> [w1064]
          tunnel: w884 -> [w1063]
          shift-right: [w1058] -> _
          shift-left: w932 -> [w1062]
          shift-right: [w1057] -> _
          shift-left: w931 -> [w1061]
          tunnel: [w1038] -> w929
          tunnel: [w1039] -> w930
          shift-right: [w1040] -> w900
          shift-left: w927 -> [w1005]
          shift-right: [w1056] -> _
          shift-left: w926 -> [w1000]
          shift-right: [w1027] -> w904
          shift-left: w915 -> [w1028]
          shift-right: [w1054] -> _
          shift-left: w925 -> [w1055]
          shift-right: [w1052] -> _
          shift-left: w924 -> [w1053]
          shift-right: [w986] -> _
          shift-left: w879 -> [w1051]
          shift-right: [w1042] -> w906
          shift-left: w920 -> [w1043]
          shift-right: [w1029] -> _
          shift-left: w918 -> [w1037]
          shift-right: [w997] -> _
          shift-left: w918 -> [w1036]
          shift-right: [w1030] -> _
          shift-left: w918 -> [w1035]
          shift-right: [w1031] -> _
          shift-left: w918 -> [w1034]
          shift-right: [w998] -> _
          shift-left: w917 -> [w1032]
          shift-right: [w999] -> _
          shift-left: w917 -> [w1033]
          shift-right: [w1011] -> _
          shift-left: w909 -> [w1012]
          shift-right: [w1010] -> w902
          shift-left: w908 -> [w1008]
          shift-right: [w1009] -> w903
          shift-left: FALSE ("output_Iconnected") -> [w1007]
          tunnel: "Host Filename Prefix" -> [w1006]
          tunnel: [w1006] -> w901
          shift-right: [w981] -> _
          shift-left: w879 -> [w1004]
          tunnel: w894 -> [w1001]
          shift-right: [w995] -> _
          shift-left: 0 ("idxDataBlock") -> [w996]
          shift-right: [w992] -> _
          shift-left: w885 -> [w994]
          shift-right: [w991] -> _
          shift-left: w885 -> [w993]
          shift-right: [w980] -> _
          shift-left: w879 -> [w987]
          shift-right: [w983] -> _
          shift-left: w879 -> [w985]
          shift-right: [w982] -> _
          shift-left: w879 -> [w984]
          shift-right: [w973] -> _
          shift-left: w879 -> [w974]
          stop <- w1050 stop-if-true
          # "Laser"
          # "Audio R"
          # "Audio L"
          # "Solenoid R"
          # "Solenoid L"
          # "manual triggering"
          # "dataTrial"
          # "dataBlock"
          # "nRewards"
          # "laserOccurred"
          # "dataExp"
          # "dataCurrent"
          # "audio__L\naudio__R"
          # "time stamp"
          # "Audio params"
          # "nRewards"
          # "idxDataBlock"
          # "idxDataBlock"
          # "activate"
          # "audio__L\naudio__R"
          # "amp__R\nfreq__R"
          # "amp__L\nfreq__L"
          # "dataLC"
          # "solenoid__R"
          # "solenoid__L"
          # "Did a lick occur?"
          # "Update lick counter"
          # "spout"
          # "spout"
          # "state"
          # "state"
          n528 = node-c288() -> ()  [unwired: 1 in, 1 out]
          n529 = local read "MTrig_Solenoid_trig__L"() -> (w1025:bool)
          n530 = local read "MTrig_Solenoid_trig__R"() -> (w1024:bool)
          n531 = local read "MTrig_Audio_trig__L"() -> (w1023:bool)
          n532 = local read "MTrig_Audio_trig__R"() -> (w1022:bool)
          n533 = xnode "Read/Write Control"("FPGA VI Reference In"=w1064, "error in"=w1063) -> ("FPGA VI Reference Out"=w990:refnum<k20>, "error out"=w989:errorcluster, "A2_LickL"=w1058:u32, "A4_LickR"=w1057:u32)
          "A2" <- w1058
          "A4" <- w1057
          n534 = local read "MTrig_Laser_trig"() -> (w1021:bool)
          n535 = Greater?(x=w1058, y=w1062) -> (0:w1060:bool)
          n536 = Greater?(x=w1057, y=w1061) -> (0:w1059:bool)
          n537 = Or(x=w1060, y=w1059) -> (x .or. y?=w1066:bool)
          n538 = call "myRIO_BRig_RT_dataMTrig_main.vi"("input_dataMTrig"=w1028, "input_Solenoid_trig_L"=w1025, "input_Solenoid_trig_R"=w1024, "input_Audio_trig_L"=w1023, "input_Audio_trig_R"=w1022, "input_Laser_trig"=w1021) -> ("output_Laser"=w978:bool, "output_dataMTrig"=w1027:u16[], "output_Solenoid_L"=w1015:bool, "output_Solenoid_R"=w1017:bool, "output_Audio_L"=w1019:bool, "output_Audio_R"=w1020:bool)  [unwired: 8 in]
          n539 = Compound Arithmetic op=OR(w1025, w1024, w1023, w1022, w1021) -> (w1026:bool)
          n540 = case shown="True" w1026 {
            frame False {
            }
            frame True {
              w1068 = FALSE
              n541 = local write "MTrig_Solenoid_trig__L"(w1068) -> ()
              n542 = local write "MTrig_Solenoid_trig__R"(w1068) -> ()
              n543 = local write "MTrig_Audio_trig__L"(w1068) -> ()
              n544 = local write "MTrig_Audio_trig__R"(w1068) -> ()
              n545 = local write "MTrig_Laser_trig"(w1068) -> ()
            }
          }
          n546 = case shown="\"ENL1\"" w1044 {
            selector: w1044 -> [_ _ _ _ _ _ _ _ _ _ _ _ _ _ _ _ _ _ _ _ w1781 _ w1846 _ _ _ _ _ w1988 _ w2063 _ _ _ _ _ w2192 _ w2269 _ w2333 _ w2377 _ _ w2448 _ _ _ _ _ w2620 _ _ _ _ _ _ _ _ _ _ _ _ _ _ _ _ _ _ _]
            tunnel: [myRIO_BRig_RT__Case_Exp_stateList."Start2" ("Enum") myRIO_BRig_RT__Case_Exp_stateList."Start3" ("Enum") myRIO_BRig_RT__Case_Exp_stateList."saveSettings1" ("Enum") myRIO_BRig_RT__Case_Exp_stateList."saveSettings2" ("Enum") myRIO_BRig_RT__Case_Exp_stateList."saveSettings3" ("Enum") myRIO_BRig_RT__Case_Exp_stateList."saveSettings4_LC_ENL" ("Enum") myRIO_BRig_RT__Case_Exp_stateList."saveSettings5_LC_Cue" ("Enum") myRIO_BRig_RT__Case_Exp_stateList."saveSettings6_LC_Other" ("Enum") myRIO_BRig_RT__Case_Exp_stateList."setSettings_Audio" ("Enum") myRIO_BRig_RT__Case_Exp_stateList."setSettings_Laser" ("Enum") myRIO_BRig_RT__Case_Exp_stateList."commConnect" ("Enum") w1553 myRIO_BRig_RT__Case_Exp_stateList."initTrial" ("Enum") w1593 myRIO_BRig_RT__Case_Exp_stateList."initTrial3" ("Enum") myRIO_BRig_RT__Case_Exp_stateList."initTrial_LC_ENL1" ("Enum") myRIO_BRig_RT__Case_Exp_stateList."ENL1_pre" ("Enum") myRIO_BRig_RT__Case_Exp_stateList."initTrial_LC_Cue1" ("Enum") myRIO_BRig_RT__Case_Exp_stateList."initTrial4" ("Enum") w1740 w1778 myRIO_BRig_RT__Case_Exp_stateList."ENL1Penalty" ("Enum") w1847 myRIO_BRig_RT__Case_Exp_stateList."endExp" ("Enum") myRIO_BRig_RT__Case_Exp_stateList."endExp" ("Enum") myRIO_BRig_RT__Case_Exp_stateList."endExp" ("Enum") myRIO_BRig_RT__Case_Exp_stateList."endExp" ("Enum") w1942 w1987 myRIO_BRig_RT__Case_Exp_stateList."Cue1Penalty" ("Enum") w2061 myRIO_BRig_RT__Case_Exp_stateList."endExp" ("Enum") myRIO_BRig_RT__Case_Exp_stateList."endExp" ("Enum") myRIO_BRig_RT__Case_Exp_stateList."endExp" ("Enum") myRIO_BRig_RT__Case_Exp_stateList."endExp" ("Enum") w2149 w2200 myRIO_BRig_RT__Case_Exp_stateList."SelectReward" ("Enum") w2270 myRIO_BRig_RT__Case_Exp_stateList."SelectRewardPost" ("Enum") w2334 myRIO_BRig_RT__Case_Exp_stateList."SelectWrong" ("Enum") w2373 myRIO_BRig_RT__Case_Exp_stateList."endTrial1" ("Enum") myRIO_BRig_RT__Case_Exp_stateList."SelectTimeout" ("Enum") w2450 myRIO_BRig_RT__Case_Exp_stateList."endTrial1" ("Enum") myRIO_BRig_RT__Case_Exp_stateList."endTrial2" ("Enum") myRIO_BRig_RT__Case_Exp_stateList."saveData_dataBlock" ("Enum") w2533 w2603 w2620 myRIO_BRig_RT__Case_Exp_stateList."initBlock" ("Enum") w2647 myRIO_BRig_RT__Case_Exp_stateList."commUpload_dataCurrent" ("Enum") myRIO_BRig_RT__Case_Exp_stateList."commUpload_dataExp" ("Enum") myRIO_BRig_RT__Case_Exp_stateList."commUpload_dataLC" ("Enum") myRIO_BRig_RT__Case_Exp_stateList."commUpload_dataTrial" ("Enum") myRIO_BRig_RT__Case_Exp_stateList."endTrial3" ("Enum") myRIO_BRig_RT__Case_Exp_stateList."saveData_dataCurrent" ("Enum") myRIO_BRig_RT__Case_Exp_stateList."saveData_dataExp" ("Enum") myRIO_BRig_RT__Case_Exp_stateList."saveData_dataLC" ("Enum") myRIO_BRig_RT__Case_Exp_stateList."saveData_dataTrial" ("Enum") myRIO_BRig_RT__Case_Exp_stateList."commUpload_pre" ("Enum") myRIO_BRig_RT__Case_Exp_stateList."empty_endBlock2" ("Enum") myRIO_BRig_RT__Case_Exp_stateList."initBlock" ("Enum") myRIO_BRig_RT__Case_Exp_stateList."empty_endTrial2" ("Enum") myRIO_BRig_RT__Case_Exp_stateList."empty_endTrial3" ("Enum") myRIO_BRig_RT__Case_Exp_stateList."empty_endTrial4" ("Enum") myRIO_BRig_RT__Case_Exp_stateList."empty_endTrial5" ("Enum") myRIO_BRig_RT__Case_Exp_stateList."initTrial" ("Enum")] -> w1013
            tunnel: [w1094 w1113 w1135 w1192 w1236 w1293 w1345 w1397 w1441 w1465 w1525 w1529 w1561 w1594 w1610 w1631 w1665 w1689 w1715 w1756 w1794 w1824 w1851 w1867 w1889 w1908 w1927 w1961 w2009 w2034 w2060 w2081 w2102 w2121 w2140 w2160 w2218 w2243 w2266 w2281 w2331 w2355 w2388 w2409 w2429 w2461 w2484 w2496 w2515 w2557 w2576 w2619 w2636 w2650 w2684 w2705 w2726 w2747 w2768 w2796 w2816 w2843 w2863 w2888 w2907 w2926 w2945 w2964 w2983 w3002 w3021] -> w1065
            tunnel: w1067 -> [w1094 w1113 w1135 w1192 w1236 w1293 w1345 w1397 w1441 w1465 w1525 w1552 w1561 w1594 w1610 w1631 w1665 w1689 w1715 w1756 w1794 w1824 w1851 w1867 w1889 w1908 w1927 w1961 w2009 w2034 w2060 w2081 w2102 w2121 w2140 w2160 w2218 w2243 w2266 w2281 w2331 w2355 w2388 w2409 w2429 w2461 w2484 w2496 w2515 w2557 w2576 w2619 w2636 w2650 w2684 w2705 w2726 w2747 w2768 w2796 w2816 w2843 w2863 w2888 w2907 w2926 w2945 w2964 w2983 w3002 w3021]
            tunnel: w1066 -> [w1097 w1116 w1132 w1195 w1239 w1296 w1348 w1400 w1444 w1468 w1528 w1546 w1572 w1595 w1628 w1648 w1679 w1702 w1728 w1743 w1775 w1827 w1854 w1873 w1892 w1911 w1930 w1941 w1986 w2042 w2067 w2086 w2105 w2124 w2143 w2158 w2216 w2253 w2277 w2312 w2339 w2366 w2391 w2408 w2441 w2466 w2481 w2504 w2514 w2568 w2602 w2623 w2633 w2659 w2687 w2708 w2729 w2750 w2771 w2799 w2819 w2846 w2866 w2891 w2910 w2929 w2948 w2967 w2986 w3005 w3024]
            tunnel: w1060 -> [w1096 w1115 w1133 w1194 w1238 w1295 w1347 w1399 w1443 w1467 w1527 w1545 w1571 w1596 w1627 w1649 w1680 w1703 w1729 w1766 w1796 w1826 w1853 w1872 w1891 w1910 w1929 w1975 w2010 w2041 w2066 w2085 w2104 w2123 w2142 w2159 w2215 w2252 w2276 w2311 w2338 w2365 w2390 w2407 w2440 w2465 w2482 w2505 w2513 w2567 w2601 w2622 w2634 w2660 w2686 w2707 w2728 w2749 w2770 w2798 w2818 w2845 w2865 w2890 w2909 w2928 w2947 w2966 w2985 w3004 w3023]
            tunnel: w1059 -> [w1095 w1114 w1134 w1193 w1237 w1294 w1346 w1398 w1442 w1466 w1526 w1544 w1570 w1597 w1626 w1650 w1681 w1704 w1730 w1765 w1795 w1825 w1852 w1871 w1890 w1909 w1928 w1974 w2011 w2040 w2065 w2084 w2103 w2122 w2141 w2178 w2219 w2251 w2275 w2310 w2337 w2364 w2389 w2406 w2439 w2464 w2483 w2506 w2512 w2566 w2600 w2621 w2635 w2661 w2685 w2706 w2727 w2748 w2769 w2797 w2817 w2844 w2864 w2889 w2908 w2927 w2946 w2965 w2984 w3003 w3022]
            tunnel: [w1097 w1116 w1132 w1195 w1239 w1296 w1348 w1400 w1444 w1468 w1528 w1546 w1572 w1595 w1628 w1648 w1679 w1702 w1728 w1743 w1775 w1827 w1854 w1873 w1892 w1911 w1930 w1941 w1986 w2042 w2067 w2086 w2105 w2124 w2143 w2158 w2216 w2253 w2277 w2312 w2339 w2366 w2391 w2408 w2441 w2466 w2481 w2504 w2514 w2568 w2602 w2623 w2633 w2659 w2687 w2708 w2729 w2750 w2771 w2799 w2819 w2846 w2866 w2891 w2910 w2929 w2948 w2967 w2986 w3005 w3024] -> w1047
            tunnel: [w1096 w1115 w1133 w1194 w1238 w1295 w1347 w1399 w1443 w1467 w1527 w1545 w1571 w1596 w1627 w1649 w1680 w1703 w1729 w1766 w1796 w1826 w1853 w1872 w1891 w1910 w1929 w1975 w2010 w2041 w2066 w2085 w2104 w2123 w2142 w2159 w2215 w2252 w2276 w2311 w2338 w2365 w2390 w2407 w2440 w2465 w2482 w2505 w2513 w2567 w2601 w2622 w2634 w2660 w2686 w2707 w2728 w2749 w2770 w2798 w2818 w2845 w2865 w2890 w2909 w2928 w2947 w2966 w2985 w3004 w3023] -> w1046
            tunnel: [w1095 w1114 w1134 w1193 w1237 w1294 w1346 w1398 w1442 w1466 w1526 w1544 w1570 w1597 w1626 w1650 w1681 w1704 w1730 w1765 w1795 w1825 w1852 w1871 w1890 w1909 w1928 w1974 w2011 w2040 w2065 w2084 w2103 w2122 w2141 w2178 w2219 w2251 w2275 w2310 w2337 w2364 w2389 w2406 w2439 w2464 w2483 w2506 w2512 w2566 w2600 w2621 w2635 w2661 w2685 w2706 w2727 w2748 w2769 w2797 w2817 w2844 w2864 w2889 w2908 w2927 w2946 w2965 w2984 w3003 w3022] -> w1045
            tunnel: w1005 -> [w1093 w1112 w1131 w1153 w1212 w1270 w1344 w1396 w1440 w1463 w1483 w1551 w1560 w1592 w1599 w1632 w1660 w1686 w1714 w1755 w1780 w1818 w1850 w1868 w1888 w1907 w1926 w1945 w2006 w2033 w2064 w2082 w2101 w2120 w2139 w2169 w2196 w2235 w2272 w2283 w2336 w2356 w2387 w2405 w2430 w2463 w2480 w2493 w2517 w2537 w2574 w2618 w2637 w2662 w2681 w2702 w2723 w2744 w2755 w2785 w2804 w2828 w2860 w2877 w2897 w2916 w2935 w2954 w2973 w2992 w3011]
            tunnel: w1000 -> [w1092 w1111 w1130 w1190 w1234 w1290 w1342 w1394 w1438 w1456 w1521 w1550 w1569 w1591 w1607 w1636 w1667 w1692 w1718 w1758 w1793 w1817 w1848 w1870 w1887 w1906 w1925 w1963 w2008 w2031 w2059 w2083 w2100 w2119 w2138 w2171 w2217 w2249 w2274 w2304 w2332 w2357 w2385 w2404 w2432 w2460 w2479 w2503 w2520 w2536 w2593 w2617 w2638 w2663 w2680 w2701 w2722 w2743 w2756 w2793 w2813 w2824 w2859 w2885 w2904 w2923 w2942 w2961 w2980 w2999 w3018]
            tunnel: [w1093 w1112 w1131 w1153 w1212 w1269 w1344 w1396 w1440 w1463 w1506 w1535 w1560 w1580 w1599 w1632 w1660 w1685 w1713 w1759 w1779 w1819 w1849 w1868 w1888 w1907 w1926 w1970 w2005 w2032 w2062 w2082 w2101 w2120 w2139 w2172 w2191 w2250 w2271 w2305 w2335 w2358 w2386 w2405 w2433 w2462 w2480 w2492 w2516 w2537 w2572 w2618 w2637 w2662 w2681 w2702 w2723 w2744 w2755 w2785 w2804 w2828 w2860 w2877 w2897 w2916 w2935 w2954 w2973 w2992 w3011] -> w1041
            tunnel: [w1092 w1111 w1130 w1189 w1233 w1285 w1342 w1394 w1438 w1456 w1521 w1549 w1569 w1590 w1607 w1636 w1667 w1692 w1718 w1758 w1793 w1817 w1848 w1870 w1887 w1906 w1925 w1963 w2008 w2031 w2059 w2083 w2100 w2119 w2138 w2171 w2217 w2249 w2274 w2304 w2332 w2357 w2385 w2404 w2432 w2460 w2479 w2503 w2520 w2536 w2593 w2617 w2638 w2663 w2680 w2701 w2722 w2743 w2756 w2793 w2813 w2827 w2859 w2885 w2904 w2923 w2942 w2961 w2980 w2999 w3018] -> w1056
            tunnel: [_ _ _ _ _ _ _ _ _ _ _ _ _ _ _ _ _ _ _ _ _ _ _ _ _ _ _ _ _ _ _ _ _ _ _ _ _ _ w2264 _ _ _ _ _ _ _ _ _ _ _ _ _ _ _ _ _ _ _ _ _ _ _ _ _ _ _ _ _ _ _ _] -> w1016
            tunnel: [_ _ _ _ _ _ _ _ _ _ _ _ _ _ _ _ _ _ _ _ _ _ _ _ _ _ _ _ _ _ _ _ _ _ _ _ _ _ w2265 _ _ _ _ _ _ _ _ _ _ _ _ _ _ _ _ _ _ _ _ _ _ _ _ _ _ _ _ _ _ _ _] -> w1018
            tunnel: w1055 -> [w1090 w1109 w1128 w1155 w1214 w1291 w1343 w1395 w1439 w1461 w1522 w1547 w1562 w1588 w1619 w1646 w1677 w1682 w1710 w1757 w1792 w1814 w1844 w1869 w1885 w1904 w1923 w1969 w2007 w2030 w2057 w2079 w2098 w2117 w2136 w2170 w2213 w2241 w2273 w2285 w2329 w2354 w2382 w2402 w2431 w2459 w2477 w2495 w2522 w2564 w2585 w2615 w2640 w2665 w2678 w2699 w2720 w2741 w2765 w2779 w2806 w2834 w2853 w2879 w2898 w2917 w2936 w2955 w2974 w2993 w3012]
            tunnel: [w1090 w1109 w1128 w1155 w1214 w1291 w1343 w1395 w1439 w1461 w1522 w1547 w1559 w1588 w1619 w1646 w1677 w1682 w1710 w1757 w1792 w1814 w1844 w1869 w1885 w1904 w1923 w1969 w2007 w2030 w2057 w2079 w2098 w2117 w2136 w2170 w2213 w2241 w2273 w2284 w2329 w2354 w2382 w2402 w2431 w2459 w2477 w2494 w2522 w2564 w2585 w2615 w2640 w2665 w2678 w2699 w2720 w2741 w2765 w2779 w2806 w2834 w2853 w2879 w2898 w2917 w2936 w2955 w2974 w2993 w3012] -> w1054
            tunnel: w1053 -> [w1091 w1110 w1129 w1154 w1213 w1292 w1340 w1392 w1436 w1462 w1523 w1548 w1568 w1589 w1598 w1647 w1678 w1690 w1716 w1754 w1774 w1815 w1845 w1866 w1886 w1905 w1924 w1968 w1985 w2029 w2058 w2080 w2099 w2118 w2137 w2168 w2214 w2242 w2268 w2302 w2330 w2353 w2384 w2403 w2428 w2457 w2478 w2502 w2521 w2565 w2592 w2616 w2639 w2664 w2679 w2700 w2721 w2742 w2766 w2792 w2812 w2840 w2851 w2884 w2903 w2922 w2941 w2960 w2979 w2998 w3017]
            tunnel: [w1091 w1110 w1129 w1154 w1213 w1292 w1341 w1393 w1437 w1462 w1523 w1548 w1568 w1589 w1598 w1647 w1678 w1690 w1716 w1754 w1774 w1815 w1845 w1866 w1886 w1905 w1924 w1968 w1985 w2029 w2058 w2080 w2099 w2118 w2137 w2168 w2214 w2242 w2268 w2302 w2330 w2353 w2384 w2403 w2428 w2457 w2478 w2502 w2521 w2565 w2592 w2616 w2639 w2664 w2679 w2700 w2721 w2742 w2766 w2792 w2812 w2840 w2851 w2884 w2903 w2922 w2941 w2960 w2979 w2998 w3017] -> w1052
            tunnel: w1051 -> [_ _ _ _ _ _ _ _ _ _ _ _ _ _ _ _ _ _ _ w1739 w1767 w1800 w1833 _ _ _ _ _ w1979 w2016 _ _ _ _ _ _ _ _ w2267 _ _ _ w2383 _ _ w2458 _ _ _ _ _ _ _ _ _ _ _ _ _ _ _ _ _ _ _ _ _ _ _ _ _]
            tunnel: [_ _ _ _ _ _ _ _ _ _ _ _ _ _ _ _ _ _ _ _ _ _ _ _ _ _ _ _ _ _ _ _ _ _ _ _ _ _ _ _ _ _ _ _ _ _ _ _ _ _ _ TRUE _ _ _ _ _ _ _ _ _ _ _ _ _ _ _ _ _ _ _] -> w1048
            tunnel: w1037 -> [w1088 w1107 w1126 w1145 w1207 w1280 w1327 w1379 w1408 _ w1513 w1543 w1567 w1587 w1618 w1645 w1676 w1701 w1727 w1753 w1791 w1812 w1843 w1864 w1883 w1902 w1921 w1967 w2002 w2027 w2056 w2077 w2096 w2115 w2134 w2167 w2212 w2231 w2263 w2300 w2328 w2351 w2381 w2401 w2426 w2456 w2476 w2500 w2526 w2563 w2589 w2613 w2631 w2658 w2676 w2697 w2718 w2739 w2763 w2790 w2810 w2838 w2857 w2883 w2902 w2921 w2940 w2959 w2978 w2997 w3016]
            tunnel: w1036 -> [w1087 w1106 w1125 w1144 w1206 w1279 w1326 w1378 w1409 _ w1512 w1542 w1566 w1586 w1617 w1644 w1675 w1700 w1726 w1752 w1790 w1811 w1842 w1863 w1882 w1901 w1920 w1966 w2001 w2026 w2055 w2076 w2095 w2114 w2133 w2166 w2211 w2230 w2262 w2299 w2327 w2350 w2380 w2400 w2425 w2455 w2475 w2499 w2525 w2562 w2588 w2612 w2630 w2657 w2675 w2696 w2717 w2738 w2762 w2789 w2809 w2837 w2856 w2882 w2901 w2920 w2939 w2958 w2977 w2996 w3015]
            tunnel: w1035 -> [w1086 w1105 w1124 w1143 w1205 w1278 w1325 w1377 w1410 _ w1511 w1541 w1565 w1585 w1616 w1643 w1674 w1699 w1725 w1751 w1789 w1810 w1841 w1862 w1881 w1900 w1919 w1965 w2000 w2025 w2054 w2075 w2094 w2113 w2132 w2165 w2210 w2229 w2261 w2298 w2326 w2349 w2379 w2399 w2424 w2454 w2474 w2498 w2524 w2561 w2587 w2611 w2629 w2656 w2674 w2695 w2716 w2737 w2761 w2788 w2808 w2836 w2855 w2881 w2900 w2919 w2938 w2957 w2976 w2995 w3014]
            tunnel: w1034 -> [w1085 w1104 w1123 w1142 w1204 w1277 w1324 w1376 w1411 _ w1510 w1540 w1564 w1584 w1615 w1642 w1673 w1698 w1724 w1750 w1788 w1809 w1840 w1861 w1880 w1899 w1918 w1964 w1999 w2024 w2053 w2074 w2093 w2112 w2131 w2164 w2209 w2228 w2260 w2297 w2325 w2348 w2378 w2398 w2423 w2453 w2473 w2497 w2523 w2560 w2586 w2610 w2628 w2655 w2673 w2694 w2715 w2736 w2760 w2787 w2807 w2835 w2854 w2880 w2899 w2918 w2937 w2956 w2975 w2994 w3013]
            tunnel: w1033 -> [_ _ _ _ _ _ _ _ _ _ _ _ _ _ _ _ _ _ _ _ _ _ _ _ _ _ _ _ w2004 _ _ _ _ _ _ _ _ _ _ _ _ _ _ _ _ _ _ _ _ _ _ _ _ _ _ _ _ _ _ _ _ _ _ _ _ _ _ _ _ _ _]
            tunnel: w1032 -> [_ _ _ _ _ _ _ _ _ _ _ _ _ _ _ _ _ _ _ _ _ _ _ _ _ _ _ _ w2003 _ _ _ _ _ _ _ _ _ _ _ _ _ _ _ _ _ _ _ _ _ _ _ _ _ _ _ _ _ _ _ _ _ _ _ _ _ _ _ _ _ _]
            tunnel: [w1088 w1107 w1126 w1145 w1207 w1280 w1327 w1379 w1408 w1455 w1513 w1543 w1567 w1587 w1618 w1645 w1676 w1701 w1727 w1753 w1791 w1812 w1843 w1864 w1883 w1902 w1921 w1967 w2002 w2027 w2056 w2077 w2096 w2115 w2134 w2167 w2212 w2231 w2263 w2300 w2328 w2351 w2381 w2401 w2426 w2456 w2476 w2500 w2526 w2563 w2589 w2613 w2631 w2658 w2676 w2697 w2718 w2739 w2763 w2790 w2810 w2838 w2857 w2883 w2902 w2921 w2940 w2959 w2978 w2997 w3016] -> w1029
            tunnel: [w1087 w1106 w1125 w1144 w1206 w1279 w1326 w1378 w1409 w1454 w1512 w1542 w1566 w1586 w1617 w1644 w1675 w1700 w1726 w1752 w1790 w1811 w1842 w1863 w1882 w1901 w1920 w1966 w2001 w2026 w2055 w2076 w2095 w2114 w2133 w2166 w2211 w2230 w2262 w2299 w2327 w2350 w2380 w2400 w2425 w2455 w2475 w2499 w2525 w2562 w2588 w2612 w2630 w2657 w2675 w2696 w2717 w2738 w2762 w2789 w2809 w2837 w2856 w2882 w2901 w2920 w2939 w2958 w2977 w2996 w3015] -> w997
            tunnel: [w1086 w1105 w1124 w1143 w1205 w1278 w1325 w1377 w1410 w1453 w1511 w1541 w1565 w1585 w1616 w1643 w1674 w1699 w1725 w1751 w1789 w1810 w1841 w1862 w1881 w1900 w1919 w1965 w2000 w2025 w2054 w2075 w2094 w2113 w2132 w2165 w2210 w2229 w2261 w2298 w2326 w2349 w2379 w2399 w2424 w2454 w2474 w2498 w2524 w2561 w2587 w2611 w2629 w2656 w2674 w2695 w2716 w2737 w2761 w2788 w2808 w2836 w2855 w2881 w2900 w2919 w2938 w2957 w2976 w2995 w3014] -> w1030
            tunnel: [w1085 w1104 w1123 w1142 w1204 w1277 w1324 w1376 w1411 w1452 w1510 w1540 w1564 w1584 w1615 w1642 w1673 w1698 w1724 w1750 w1788 w1809 w1840 w1861 w1880 w1899 w1918 w1964 w1999 w2024 w2053 w2074 w2093 w2112 w2131 w2164 w2209 w2228 w2260 w2297 w2325 w2348 w2378 w2398 w2423 w2453 w2473 w2497 w2523 w2560 w2586 w2610 w2628 w2655 w2673 w2694 w2715 w2736 w2760 w2787 w2807 w2835 w2854 w2880 w2899 w2918 w2937 w2956 w2975 w2994 w3013] -> w1031
            tunnel: [_ _ _ _ _ _ _ _ _ _ _ _ _ _ _ _ _ _ _ _ _ _ _ _ _ _ _ w1954 w2004 _ _ _ _ _ _ _ _ _ _ _ _ _ _ _ _ _ _ _ _ _ _ _ _ _ _ _ _ _ _ _ _ _ _ _ _ _ _ _ _ _ _] -> w999
            tunnel: [_ _ _ _ _ _ _ _ _ _ _ _ _ _ _ _ _ _ _ _ _ _ _ _ _ _ _ w1953 w2003 _ _ _ _ _ _ _ _ _ _ _ _ _ _ _ _ _ _ _ _ _ _ _ _ _ _ _ _ _ _ _ _ _ _ _ _ _ _ _ _ _ _] -> w998
            tunnel: w1012 -> [w1084 w1103 w1122 w1141 w1203 w1276 w1323 w1375 w1407 w1451 w1520 w1539 w1563 w1583 w1601 w1634 w1659 w1684 w1712 w1749 w1787 w1808 w1839 w1860 w1879 w1898 w1917 w1952 w1998 w2023 w2052 w2073 w2092 w2111 w2130 w2163 w2208 w2225 w2259 w2296 w2324 w2345 w2372 w2397 w2420 w2447 w2472 w2491 w2519 w2553 w2584 w2609 w2641 w2666 w2677 w2698 w2719 w2740 w2764 w2791 w2811 w2839 w2858 w2874 w2896 w2915 w2934 w2953 w2972 w2991 w3010]
            tunnel: [w1084 w1103 w1122 w1141 w1203 w1276 w1323 w1375 w1407 w1451 w1520 w1539 w1563 w1583 w1600 w1633 w1652 w1683 w1711 w1749 w1787 w1808 w1839 w1860 w1879 w1898 w1917 w1952 w1998 w2023 w2052 w2073 w2092 w2111 w2130 w2163 w2208 w2225 w2259 w2296 w2324 w2345 w2372 w2397 w2420 w2447 w2472 w2491 w2518 w2553 w2584 w2609 w2641 w2666 w2677 w2698 w2719 w2740 w2764 w2791 w2811 w2839 w2858 w2874 w2896 w2915 w2934 w2953 w2972 w2991 w3010] -> w1011
            tunnel: [w1083 w1102 w1121 w1140 w1202 w1275 w1322 w1374 w1406 w1450 w1519 w1538 w1574 w1582 w1621 w1641 w1672 w1697 w1723 w1748 w1786 w1807 w1838 w1859 w1878 w1897 w1916 w1951 w1997 w2022 w2051 w2072 w2091 w2110 w2129 w2162 w2207 w2224 w2258 w2295 w2323 w2344 w2371 w2396 w2419 w2446 w2471 w2490 w2511 w2559 w2583 w2607 w2642 w2652 w2672 w2693 w2714 w2735 w2759 w2795 w2815 w2842 w2862 w2887 w2906 w2925 w2944 w2963 w2982 w3001 w3020] -> w1010
            tunnel: [w1082 w1101 w1120 w1139 w1201 w1274 w1321 w1373 w1405 w1449 w1518 w1537 w1573 w1581 w1620 w1640 w1671 w1696 w1722 w1747 w1785 w1806 w1837 w1858 w1877 w1896 w1915 w1950 w1996 w2021 w2050 w2071 w2090 w2109 w2128 w2161 w2206 w2223 w2257 w2294 w2322 w2343 w2370 w2395 w2418 w2445 w2470 w2489 w2510 w2558 w2582 w2608 w2624 w2649 w2682 w2703 w2724 w2745 w2767 w2794 w2814 w2841 w2861 w2886 w2905 w2924 w2943 w2962 w2981 w3000 w3019] -> w1009
            tunnel: w1008 -> [w1083 w1102 w1121 w1140 w1202 w1275 w1322 w1374 w1406 w1450 w1519 w1538 w1574 w1582 w1621 w1641 w1672 w1697 w1723 w1748 w1786 w1807 w1838 w1859 w1878 w1897 w1916 w1951 w1997 w2022 w2051 w2072 w2091 w2110 w2129 w2162 w2207 w2224 w2258 w2295 w2323 w2344 w2371 w2396 w2419 w2446 w2471 w2490 w2511 w2559 w2583 w2607 _ w2652 w2672 w2693 w2714 w2735 w2759 w2795 w2815 w2842 w2862 w2887 w2906 w2925 w2944 w2963 w2982 w3001 w3020]
            tunnel: w1007 -> [w1082 w1101 w1120 w1139 w1201 w1274 w1321 w1373 w1405 w1449 w1518 w1537 w1573 w1581 w1620 w1640 w1671 w1696 w1722 w1747 w1785 w1806 w1837 w1858 w1877 w1896 w1915 w1950 w1996 w2021 w2050 w2071 w2090 w2109 w2128 w2161 w2206 w2223 w2257 w2294 w2322 w2343 w2370 w2395 w2418 w2445 w2470 w2489 w2510 w2558 w2582 w2608 _ w2649 w2682 w2703 w2724 w2745 w2767 w2794 w2814 w2841 w2861 w2886 w2905 w2924 w2943 w2962 w2981 w3000 w3019]
            tunnel: w1006 -> [_ _ _ _ _ _ _ _ _ _ _ _ _ _ _ _ _ _ _ _ _ _ _ _ _ _ _ _ _ _ _ _ _ _ _ _ _ _ _ _ _ _ _ _ _ _ _ _ _ _ _ _ _ _ w2670 w2691 w2712 w2733 w2757 _ _ _ _ _ _ _ _ _ _ _ _]
            tunnel: w1004 -> [_ _ _ _ _ _ _ _ _ _ _ _ _ _ _ _ w1664 _ w1707 w1736 w1772 w1798 w1829 _ _ _ _ w1932 w1977 w2015 w2044 _ _ _ _ _ _ _ _ _ _ _ _ _ _ _ _ _ _ _ _ _ _ _ _ _ _ _ _ _ _ _ _ _ _ _ _ _ _ _ _]
            tunnel: w1001 -> [_ _ _ _ _ _ _ _ _ _ _ _ _ _ _ _ _ _ _ _ _ _ _ _ _ _ _ _ _ _ _ _ _ _ _ _ _ _ _ _ _ _ _ _ _ _ _ _ _ _ _ _ _ _ _ _ _ _ _ _ _ w2829 _ _ _ _ _ _ _ _ _]
            tunnel: [w1081 w1100 w1119 w1138 w1200 w1273 w1320 w1372 w1404 w1448 w1517 w1532 w1557 w1577 w1622 w1639 w1670 w1695 w1721 w1746 w1784 w1805 w1836 w1857 w1876 w1895 w1914 w1949 w1995 w2020 w2049 w2070 w2089 w2108 w2127 w2157 w2205 w2222 w2256 w2279 w2321 w2342 w2369 w2394 w2417 w2444 w2469 w2488 w2509 w2556 w2569 w2606 w2627 w2651 w2669 w2690 w2711 w2732 w2754 w2774 w2803 w2823 w2850 w2870 w2895 w2914 w2933 w2952 w2971 w2990 w3009] -> w995
            tunnel: w996 -> [w1081 w1100 w1119 w1138 w1200 w1273 w1320 w1372 w1404 w1448 w1517 w1532 _ w1577 w1622 w1639 w1670 w1695 w1721 w1746 w1784 w1805 w1836 w1857 w1876 w1895 w1914 w1949 w1995 w2020 w2049 w2070 w2089 w2108 w2127 w2157 w2205 w2222 w2256 w2279 w2321 w2342 w2369 w2394 w2417 w2444 w2469 w2488 w2509 w2556 w2570 w2606 w2627 w2651 w2669 w2690 w2711 w2732 w2754 w2774 w2803 w2823 w2850 w2870 w2895 w2914 w2933 w2952 w2971 w2990 w3009]
            tunnel: w994 -> [w1080 w1099 w1118 w1137 w1199 w1272 w1319 w1371 w1403 w1447 w1516 w1531 w1556 w1576 w1614 w1638 w1669 w1694 w1720 w1745 w1783 w1804 w1835 w1856 w1875 w1894 w1913 w1948 w1994 w2019 w2048 w2069 w2088 w2107 w2126 w2156 w2204 w2221 w2255 w2293 w2320 w2341 w2368 w2393 w2416 w2443 w2468 w2487 w2508 w2555 w2581 w2605 w2626 w2654 w2668 w2689 w2710 w2731 w2753 w2773 w2802 w2822 w2849 w2869 w2894 w2913 w2932 w2951 w2970 w2989 w3008]
            tunnel: w993 -> [w1079 w1098 w1117 w1136 w1198 w1271 w1318 w1370 w1402 w1446 w1515 w1530 w1555 w1575 w1613 w1637 w1668 w1693 w1719 w1744 w1782 w1803 w1834 w1855 w1874 w1893 w1912 w1947 w1993 w2018 w2047 w2068 w2087 w2106 w2125 w2155 w2203 w2220 w2254 w2290 w2319 w2340 w2367 w2392 w2415 w2442 w2467 w2486 w2507 w2554 w2580 w2604 w2625 w2653 w2667 w2688 w2709 w2730 w2752 w2772 w2801 w2821 w2848 w2868 w2893 w2912 w2931 w2950 w2969 w2988 w3007]
            tunnel: [w1080 w1099 w1118 w1137 w1199 w1272 w1319 w1371 w1403 w1447 w1516 w1531 w1556 w1576 w1614 w1638 w1669 w1694 w1720 w1745 w1783 w1804 w1835 w1856 w1875 w1894 w1913 w1948 w1994 w2019 w2048 w2069 w2088 w2107 w2126 w2156 w2204 w2221 w2255 w2292 w2320 w2341 w2368 w2393 w2416 w2443 w2468 w2487 w2508 w2555 w2581 w2605 w2626 w2654 w2668 w2689 w2710 w2731 w2753 w2773 w2802 w2822 w2849 w2869 w2894 w2913 w2932 w2951 w2970 w2989 w3008] -> w992
            tunnel: [w1079 w1098 w1117 w1136 w1198 w1271 w1318 w1370 w1402 w1446 w1515 w1530 w1555 w1575 w1613 w1637 w1668 w1693 w1719 w1744 w1782 w1803 w1834 w1855 w1874 w1893 w1912 w1947 w1993 w2018 w2047 w2068 w2087 w2106 w2125 w2155 w2203 w2220 w2254 w2291 w2319 w2340 w2367 w2392 w2415 w2442 w2467 w2486 w2507 w2554 w2580 w2604 w2625 w2653 w2667 w2688 w2709 w2730 w2752 w2772 w2801 w2821 w2848 w2868 w2893 w2912 w2931 w2950 w2969 w2988 w3007] -> w991
            tunnel: w990 -> [_ _ _ _ _ _ _ _ _ _ w1507 _ _ _ w1625 _ _ _ _ _ _ _ _ _ _ _ _ _ w1990 _ _ _ _ _ _ w2153 w2202 _ _ _ _ _ _ _ w2414 _ _ _ _ w2531 _ _ _ _ _ _ _ _ _ _ _ _ _ _ _ _ _ _ _ _ _]
            tunnel: w989 -> [_ _ _ _ _ _ _ _ _ _ w1508 _ _ _ w1624 _ _ _ _ _ _ _ _ _ _ _ _ _ w1989 _ _ _ _ _ _ w2154 w2201 _ _ _ _ _ _ _ w2413 _ _ _ _ w2530 _ _ _ _ _ _ _ _ _ _ _ _ _ _ _ _ _ _ _ _ _]
            tunnel: w987 -> [_ _ _ _ _ _ _ _ _ _ _ _ _ _ _ _ w1663 _ w1706 w1735 w1771 w1797 w1830 _ _ _ _ w1931 w1976 w2014 w2043 _ _ _ _ _ _ _ _ _ _ _ _ _ _ _ _ _ _ _ _ _ _ _ _ _ _ _ _ _ _ _ _ _ _ _ _ _ _ _ _]
            tunnel: [_ _ _ _ _ _ _ _ _ _ _ _ _ _ _ _ _ _ _ w1739 w1773 w1800 w1833 _ _ _ _ TRUE w1979 w2016 _ _ _ _ _ _ _ _ _ _ _ _ _ _ _ _ _ _ _ _ _ _ _ _ _ _ _ _ _ _ _ _ _ _ _ _ _ _ _ _ _] -> w986
            tunnel: w985 -> [_ _ _ _ _ _ _ _ _ _ _ _ _ _ _ _ w1662 _ _ w1738 w1777 w1802 w1831 _ _ _ _ w1939 w1984 w2013 w2046 _ _ _ _ _ _ _ _ _ _ _ _ _ _ _ _ _ _ _ _ _ _ _ _ _ _ _ _ _ _ _ _ _ _ _ _ _ _ _ _]
            tunnel: w984 -> [_ _ _ _ _ _ _ _ _ _ _ _ _ _ _ _ w1661 _ _ w1737 w1776 w1801 w1832 _ _ _ _ w1938 w1983 w2012 w2045 _ _ _ _ _ _ _ _ _ _ _ _ _ _ _ _ _ _ _ _ _ _ _ _ _ _ _ _ _ _ _ _ _ _ _ _ _ _ _ _]
            tunnel: [_ _ _ _ _ _ _ _ _ _ _ _ _ _ _ _ w1662 _ w1709 w1738 w1777 w1802 w1831 _ _ _ _ w1939 w1984 w2013 w2046 _ _ _ _ _ _ _ _ _ _ _ _ _ _ _ _ _ _ _ _ _ _ _ _ _ _ _ _ _ _ _ _ _ _ _ _ _ _ _ _] -> w983
            tunnel: [_ _ _ _ _ _ _ _ _ _ _ _ _ _ _ _ w1661 _ w1708 w1737 w1776 w1801 w1832 _ _ _ _ w1938 w1983 w2012 w2045 _ _ _ _ _ _ _ _ _ _ _ _ _ _ _ _ _ _ _ _ _ _ _ _ _ _ _ _ _ _ _ _ _ _ _ _ _ _ _ _] -> w982
            tunnel: [_ _ _ _ _ _ _ _ _ _ _ _ _ _ _ _ w1664 w1687 w1707 w1736 w1772 w1798 w1829 _ _ _ _ w1932 w1977 w2015 w2044 _ _ _ _ _ _ _ _ _ _ _ _ _ _ _ _ _ _ _ _ _ _ _ _ _ _ _ _ _ _ _ _ _ _ _ _ _ _ _ _] -> w981
            tunnel: [_ _ _ _ _ _ _ _ _ _ _ _ _ _ _ _ w1663 w1688 w1706 w1735 w1771 w1797 w1830 _ _ _ _ w1931 w1976 w2014 w2043 _ _ _ _ _ _ _ _ _ _ _ _ _ _ _ _ _ _ _ _ _ _ _ _ _ _ _ _ _ _ _ _ _ _ _ _ _ _ _ _] -> w980
            tunnel: [_ _ _ _ _ _ _ _ _ _ _ _ _ _ _ _ _ _ _ _ w1770 _ _ _ _ _ _ _ w1981 _ _ _ _ _ _ _ _ _ _ _ _ _ _ _ _ _ _ _ _ _ _ _ _ _ _ _ _ _ _ _ _ _ _ _ _ _ _ _ _ _ _] -> w977
            tunnel: [_ _ _ _ _ _ _ _ _ _ _ _ _ _ _ _ _ _ _ _ w1769 _ _ _ _ _ _ _ w1982 _ _ _ _ _ _ _ _ _ _ _ _ _ _ _ _ _ _ _ _ _ _ _ _ _ _ _ _ _ _ _ _ _ _ _ _ _ _ _ _ _ _] -> w979
            tunnel: w974 -> [_ _ _ _ _ _ _ _ _ _ _ _ _ _ _ _ _ _ _ w1734 w1768 w1799 w1828 _ _ _ _ w1934 w1978 w2017 _ _ _ _ _ _ _ _ _ _ _ _ _ _ _ _ _ _ _ _ _ _ _ _ _ _ _ _ _ _ _ _ _ _ _ _ _ _ _ _ _]
            tunnel: [_ _ _ _ _ _ _ _ _ _ _ _ _ _ _ _ _ _ _ w1734 w1768 w1799 w1828 _ _ _ _ w1934 w1980 w2017 _ _ _ _ _ _ _ _ _ _ _ _ _ _ _ _ _ _ _ _ _ _ _ _ _ _ _ _ _ _ _ _ _ _ _ _ _ _ _ _ _] -> w973
            frame "Start1", Default {
            }
            frame "Start2" {
            }
            frame "Start3" {
            }
            frame "saveSettings1" {
              n547 = call "myRIO_BRig_RT_dataExp_Audio_freq__L.vi"() -> ("output_Audio_freq__L"=w1165:i32)  [unwired: 11 in]
              n548 = call "myRIO_BRig_RT_dataExp_Audio_freq__R.vi"() -> ("output_Audio_freq__R"=w1162:i32)  [unwired: 11 in]
              n549 = call "myRIO_BRig_RT_dataExp_Audio_amp__L.vi"() -> ("output_Audio_amp__L"=w1159:i32)  [unwired: 11 in]
              n550 = call "myRIO_BRig_RT_dataExp_Audio_amp__R.vi"() -> ("output_Audio_amp__R"=w1157:i32)  [unwired: 11 in]
              n551 = call "myRIO_BRig_RT_dataExp_TPB_min__L.vi"() -> ("output_TPB_min__L"=w1175:i32)  [unwired: 11 in]
              n552 = call "myRIO_BRig_RT_dataExp_TPB_min__R.vi"() -> ("output_TPB_min__R"=w1173:i32)  [unwired: 11 in]
              n553 = call "myRIO_BRig_RT_dataExp_TPB_max__L.vi"() -> ("output_TPB_max__L"=w1171:i32)  [unwired: 11 in]
              n554 = call "myRIO_BRig_RT_dataExp_TPB_max__R.vi"() -> ("output_TPB_max__R"=w1169:i32)  [unwired: 11 in]
              n555 = call "myRIO_BRig_RT_dataExp_ItrialUntilReward.vi"() -> ("output_I_trialUntilReward"=w1188:i32)  [unwired: 11 in]
              n556 = call "myRIO_BRig_RT_dataExp_IblockUntilReward.vi"() -> ("output_I_blockUntilReward"=w1184:i32)  [unwired: 11 in]
              n557 = call "myRIO_BRig_RT_dataExp_CueCycles.vi"() -> ("output_CueCycles"=w1183:i32)  [unwired: 11 in]
              n558 = call "myRIO_BRig_RT_dataExp_ENL_min.vi"() -> ("output_ENL_min"=w1181:i32)  [unwired: 11 in]
              n559 = call "myRIO_BRig_RT_dataExp_ENL_max.vi"() -> ("output_ENL_max"=w1179:i32)  [unwired: 11 in]
              n560 = call "myRIO_BRig_RT_dataExp_ENL_penalty.vi"() -> ("output_ENL_penalty"=w1177:i32)  [unwired: 11 in]
              n561 = local read "Audio_Freq__L"() -> (w1166:u16)
              n562 = local read "Audio_Freq__R"() -> (w1161:u16)
              n563 = local read "Audio_Amp__L"() -> (w1158:u16)
              n564 = local read "TpB_Min_L"() -> (w1174:u16)
              n565 = local read "TpB_Min_R"() -> (w1172:u16)
              n566 = local read "TpB_Max_L"() -> (w1170:u16)
              n567 = local read "TpB_Max_R"() -> (w1168:u16)
              n568 = local read "Audio_Amp__R"() -> (w1156:u16)
              n569 = local read "TrialUntilReward"() -> (w1187:bool)
              n570 = local read "CueCycles"() -> (w1182:u16)
              n571 = local read "Tcycle_ENL_min"() -> (w1180:u16)
              n572 = local read "Tcycle_ENL_max"() -> (w1178:u16)
              n573 = local read "Tcycle_ENLPenalty"() -> (w1176:u16)
              n574 = Multiply(x=w1166, y=u16 1000) -> (x*y=w1164:u16)
              n575 = Multiply(x=w1161, y=u16 1000) -> (x*y=w1160:u16)
              n576 = Boolean To (0,1)(Boolean=w1187) -> (0, 1=w1186:i16)
              n577 = To Unsigned Word Integer(number=w1186) -> (unsigned 16bit integer=w1185:u16)
              n578 = local read "BUR_min"() -> (w1150:u16)
              n579 = local read "BUR_max"() -> (w1151:u16)
              n580 = Not Equal To 0?(x=w1150) -> (x != 0?=w1149:bool)
              n581 = Not Equal To 0?(x=w1151) -> (x != 0?=w1148:bool)
              n582 = And(x=w1149, y=w1148) -> (x .and. y?=w1147:bool)
              n583 = Boolean To (0,1)(Boolean=w1147) -> (0, 1=w1152:i16)
              n584 = To Unsigned Word Integer(number=w1152) -> (unsigned 16bit integer=w1146:u16)
              n585 = Replace Array Subset(array=w1190, new element #1=w1185, index #1=w1188, new element #2=w1146, index #2=w1184, new element #3=w1182, index #3=w1183, new element #4=w1180, index #4=w1181, new element #5=w1178, index #5=w1179, new element #6=w1176, index #6=w1177, new element #7=w1174, index #7=w1175, new element #8=w1172, index #8=w1173, new element #9=w1170, index #9=w1171, new element #10=w1168, index #10=w1169, new element #11=w1164, index #11=w1165, new element #12=w1160, index #12=w1162, new element #13=w1158, index #13=w1159, new element #14=w1156, index #14=w1157) -> (w1189:u16[])
            }
            frame "saveSettings2" {
              n586 = call "myRIO_BRig_RT_dataExp_Tcycle_RewardPost.vi"() -> ("output_Tcycle_RewardPost"=w1223:i32)  [unwired: 11 in]
              n587 = call "myRIO_BRig_RT_dataExp_Tcycle_Wrong.vi"() -> ("output_Tcycle_Wrong"=w1221:i32)  [unwired: 11 in]
              n588 = call "myRIO_BRig_RT_dataExp_Tcycle_Timeout.vi"() -> ("output_Tcycle_Timeout"=w1219:i32)  [unwired: 11 in]
              n589 = call "myRIO_BRig_RT_dataExp_Tcycle_Cue_min.vi"() -> ("output_Tcycle_Cue_min"=w1217:i32)  [unwired: 11 in]
              n590 = call "myRIO_BRig_RT_dataExp_Tcycle_Cue_max.vi"() -> ("output_Tcycle_Cue_max"=w1216:i32)  [unwired: 11 in]
              n591 = call "myRIO_BRig_RT_dataExp_Tcycle_CuePenalty.vi"() -> ("output_Tcycle_CuePenalty"=w1215:i32)  [unwired: 11 in]
              n592 = call "myRIO_BRig_RT_dataExp_nBlock.vi"() -> ("output_nBlock"=w1232:i32)  [unwired: 11 in]
              n593 = call "myRIO_BRig_RT_dataExp_nTrial.vi"() -> ("output_nTrial"=w1231:i32)  [unwired: 11 in]
              n594 = call "myRIO_BRig_RT_dataExp_runTime_seconds.vi"() -> ("output_RunTime_minutes"=w1230:i32)  [unwired: 11 in]
              n595 = call "myRIO_BRig_RT_dataExp_Tcycle_Selection.vi"() -> ("output_Tcycle_Selection"=w1229:i32)  [unwired: 11 in]
              n596 = call "myRIO_BRig_RT_dataExp_Tcycle_Reward__L.vi"() -> ("output_Tcycle_Reward__L"=w1227:i32)  [unwired: 11 in]
              n597 = call "myRIO_BRig_RT_dataExp_Tcycle_Reward__R.vi"() -> ("output_Tcycle_Reward__R"=w1225:i32)  [unwired: 11 in]
              n598 = local read "Tcycle_RewardPost"() -> (w1222:u16)
              n599 = local read "Tcycle_Wrong"() -> (w1220:u16)
              n600 = local read "Tcycle_Timeout"() -> (w1218:u16)
              n601 = local read "Tcycle_CuePenalty"() -> (w1208:u16)
              n602 = local read "Tcycle_Cue_max"() -> (w1196:u16)
              n603 = local read "Tcycle_Cue_min"() -> (w1197:u16)
              n604 = local read "Tcycle_Selection"() -> (w1228:u16)
              n605 = local read "Tcycle_Reward_L"() -> (w1226:u16)
              n606 = local read "Tcycle_Reward_R"() -> (w1224:u16)
              n607 = Replace Array Subset(array=w1234, new element #1=u16 0, index #1=w1232, new element #2=u16 0, index #2=w1231, new element #3=u16 0, index #3=w1230, new element #4=w1228, index #4=w1229, new element #5=w1226, index #5=w1227, new element #6=w1224, index #6=w1225, new element #7=w1222, index #7=w1223, new element #8=w1220, index #8=w1221, new element #9=w1218, index #9=w1219, new element #10=w1197, index #10=w1217, new element #11=w1196, index #11=w1216, new element #12=w1208, index #12=w1215) -> (w1233:u16[])
            }
            frame "saveSettings3" {
              w1243 = 100.0 ("y")
              n608 = call "myRIO_BRig_RT_dataExp_laser_Freq.vi"() -> ("output_laser_Freq"=w1267:i32)  [unwired: 11 in]
              n609 = call "myRIO_BRig_RT_dataExp_laser_Tpeak.vi"() -> ("output_laser_Tpeak"=w1262:i32)  [unwired: 11 in]
              n610 = call "myRIO_BRig_RT_dataExp_laser_Tshutter.vi"() -> ("output_laser_Tshutter"=w1257:i32)  [unwired: 11 in]
              n611 = call "myRIO_BRig_RT_dataExp_laser_f_millisec2count.vi"() -> ("output_laser_f_millisec2count"=w1252:i32)  [unwired: 11 in]
              n612 = call "myRIO_BRig_RT_dataExp_laser_Power_min.vi"() -> ("output_laser_Power_min"=w1247:i32)  [unwired: 11 in]
              n613 = call "myRIO_BRig_RT_dataExp_laser_duration.vi"() -> ("output_laser_duration"=w1241:i32)  [unwired: 11 in]
              n614 = call "myRIO_BRig_RT_dataExp_BUR_min.vi"() -> ("output_BUR_min"=w1289:i32)  [unwired: 11 in]
              n615 = call "myRIO_BRig_RT_dataExp_BUR_max.vi"() -> ("output_BUR_max"=w1287:i32)  [unwired: 11 in]
              n616 = call "myRIO_BRig_RT_dataExp_Audio_sp__L.vi"() -> ("output_Audio_sp__L"=w1284:i32)  [unwired: 11 in]
              n617 = call "myRIO_BRig_RT_dataExp_Audio_sp__R.vi"() -> ("output_Audio_sp__R"=w1283:i32)  [unwired: 11 in]
              n618 = local read "laser_Tshutter"() -> (w1254:dbl)
              n619 = local read "f_millisec2count"() -> (w1249:dbl)
              n620 = local read "laser_power"() -> (w1244:dbl)
              n621 = local read "laser_Tpeak"() -> (w1259:dbl)
              n622 = local read "laser_Freq"() -> (w1266:dbl)
              n623 = local read "sp_LeftSpout"() -> (w1282:u16)
              n624 = local read "BUR_max"() -> (w1286:u16)
              n625 = local read "sp_RightSpout"() -> (w1281:u16)
              n626 = local read "BUR_min"() -> (w1288:u16)
              n627 = Multiply(x=w1259, y=w1243) -> (x*y=w1261:dbl)
              n628 = Multiply(x=w1254, y=w1243) -> (x*y=w1256:dbl)
              n629 = Multiply(x=w1249, y=w1243) -> (x*y=w1251:dbl)
              n630 = Multiply(x=w1244, y=w1243) -> (x*y=w1246:dbl)
              n631 = Multiply(x=w1266, y=w1243) -> (x*y=w1265:dbl)
              n632 = Round To Nearest(number=w1261) -> (nearest integer value=w1260:dbl)
              n633 = Round To Nearest(number=w1256) -> (nearest integer value=w1255:dbl)
              n634 = Round To Nearest(number=w1251) -> (nearest integer value=w1250:dbl)
              n635 = Round To Nearest(number=w1246) -> (nearest integer value=w1245:dbl)
              n636 = Round To Nearest(number=w1265) -> (nearest integer value=w1264:dbl)
              n637 = To Unsigned Word Integer(number=w1260) -> (unsigned 16bit integer=w1258:u16)
              n638 = To Unsigned Word Integer(number=w1255) -> (unsigned 16bit integer=w1253:u16)
              n639 = To Unsigned Word Integer(number=w1250) -> (unsigned 16bit integer=w1248:u16)
              n640 = To Unsigned Word Integer(number=w1245) -> (unsigned 16bit integer=w1242:u16)
              n641 = To Unsigned Word Integer(number=w1264) -> (unsigned 16bit integer=w1263:u16)
              n642 = local read "laser_duration"() -> (w1240:u16)
              n643 = call "myRIO_BRig_RT_dataCurrent_LaserPulse_duration.vi"() -> ("output_LaserPulse_duration"=w1268:i32)  [unwired: 11 in]
              n644 = Replace Array Subset(array=w1290, new element #1=w1288, index #1=w1289, new element #2=w1286, index #2=w1287, new element #3=w1282, index #3=w1284, new element #4=w1281, index #4=w1283, new element #5=w1263, index #5=w1267, new element #6=w1258, index #6=w1262, new element #7=w1253, index #7=w1257, new element #8=w1248, index #8=w1252, new element #9=w1242, index #9=w1247, new element #10=w1240, index #10=w1241) -> (w1285:u16[])
              n645 = Replace Array Subset(array=w1270, new element=w1240, index=w1268) -> (w1269:u16[])
            }
            frame "saveSettings4_LC_ENL" {
              # "delayOpt"
              # "Count"
              # "Tdelay"
              # "Probability"
              # "OnOff"
              # "Block"
              # "ENL1 All"
              # "delayOpt"
              # "Count"
              # "Tdelay"
              # "Probability"
              # "OnOff"
              # "Block"
              # "ENL1 First"
              n646 = call "myRIO_BRig_RT_dataLC_ENL1_All_Block.vi"() -> ("output_ENL1_All_Block"=w1313:i32)  [unwired: 11 in]
              n647 = call "myRIO_BRig_RT_dataLC_ENL1_All_OnOff.vi"() -> ("output_ENL1_All_OnOff"=w1302:i32)  [unwired: 11 in]
              n648 = call "myRIO_BRig_RT_dataLC_ENL1_All_Probability.vi"() -> ("output_ENL1_All_Probability"=w1301:i32)  [unwired: 11 in]
              n649 = call "myRIO_BRig_RT_dataLC_ENL1_All_Tdelay.vi"() -> ("output_ENL1_All_Tdelay"=w1300:i32)  [unwired: 11 in]
              n650 = call "myRIO_BRig_RT_dataLC_ENL1_All_Count.vi"() -> ("output_ENL1_All_Count"=w1299:i32)  [unwired: 11 in]
              n651 = call "myRIO_BRig_RT_dataLC_ENL1_All_delayOpt.vi"() -> ("output_ENL1_All_delayOpt"=w1298:i32)  [unwired: 11 in]
              n652 = call "myRIO_BRig_RT_dataLC_ENL1_First_Block.vi"() -> ("output_ENL1_First_Block"=w1339:i32)  [unwired: 11 in]
              n653 = call "myRIO_BRig_RT_dataLC_ENL1_First_OnOff.vi"() -> ("output_ENL1_First_OnOff"=w1337:i32)  [unwired: 11 in]
              n654 = call "myRIO_BRig_RT_dataLC_ENL1_First_Probability.vi"() -> ("output_ENL1_First_Probability"=w1333:i32)  [unwired: 11 in]
              n655 = call "myRIO_BRig_RT_dataLC_ENL1_First_Tdelay.vi"() -> ("output_ENL1_First_Tdelay"=w1331:i32)  [unwired: 11 in]
              n656 = call "myRIO_BRig_RT_dataLC_ENL1_First_Count.vi"() -> ("output_ENL1_First_Count"=w1329:i32)  [unwired: 11 in]
              n657 = call "myRIO_BRig_RT_dataLC_ENL1_First_delayOpt.vi"() -> ("output_ENL1_First_delayOpt"=w1315:i32)  [unwired: 11 in]
              n658 = local read "LC_ENL1_First_delayOpt"() -> (w1316:bool)
              n659 = local read "LC_ENL1_First_Count"() -> (w1328:u16)
              n660 = local read "LC_ENL1_First_Probability"() -> (w1332:u16)
              n661 = local read "LC_ENL1_First_Block"() -> (w1338:u16)
              n662 = local read "LC_ENL1_First_Tdelay"() -> (w1330:u16)
              n663 = local read "LC_ENL1_First_OnOff"() -> (w1336:bool)
              n664 = local read "LC_ENL1_All_OnOff"() -> (w1309:bool)
              n665 = local read "LC_ENL1_All_Probability"() -> (w1307:u16)
              n666 = local read "LC_ENL1_All_delayOpt"() -> (w1304:bool)
              n667 = local read "LC_ENL1_All_Tdelay"() -> (w1306:u16)
              n668 = local read "LC_ENL1_All_Block"() -> (w1310:u16)
              n669 = local read "LC_ENL1_All_Count"() -> (w1305:u16)
              n670 = Boolean To (0,1)(Boolean=w1316) -> (0, 1=w1317:i16)
              n671 = Boolean To (0,1)(Boolean=w1336) -> (0, 1=w1335:i16)
              n672 = Boolean To (0,1)(Boolean=w1309) -> (0, 1=w1312:i16)
              n673 = To Unsigned Word Integer(number=w1317) -> (unsigned 16bit integer=w1314:u16)
              n674 = To Unsigned Word Integer(number=w1335) -> (unsigned 16bit integer=w1334:u16)
              n675 = Boolean To (0,1)(Boolean=w1304) -> (0, 1=w1311:i16)
              n676 = To Unsigned Word Integer(number=w1312) -> (unsigned 16bit integer=w1308:u16)
              n677 = To Unsigned Word Integer(number=w1311) -> (unsigned 16bit integer=w1303:u16)
              n678 = Replace Array Subset(array=w1340, new element #1=w1338, index #1=w1339, new element #2=w1334, index #2=w1337, new element #3=w1332, index #3=w1333, new element #4=w1330, index #4=w1331, new element #5=w1328, index #5=w1329, new element #6=w1314, index #6=w1315, new element #7=w1310, index #7=w1313, new element #8=w1308, index #8=w1302, new element #9=w1307, index #9=w1301, new element #10=w1306, index #10=w1300, new element #11=w1305, index #11=w1299, new element #12=w1303, index #12=w1298) -> (w1341:u16[])
            }
            frame "saveSettings5_LC_Cue" {
              # "delayOpt"
              # "Count"
              # "Tdelay"
              # "Probability"
              # "OnOff"
              # "Block"
              # "Cue1 All"
              # "delayOpt"
              # "Count"
              # "Tdelay"
              # "Probability"
              # "OnOff"
              # "Block"
              # "Cue1 First"
              n679 = call "myRIO_BRig_RT_dataLC_Cue1_First_delayOpt.vi"() -> ("output_Cue1_First_delayOpt"=w1368:i32)  [unwired: 11 in]
              n680 = call "myRIO_BRig_RT_dataLC_Cue1_First_Block.vi"() -> ("output_Cue1_First_Block"=w1391:i32)  [unwired: 11 in]
              n681 = call "myRIO_BRig_RT_dataLC_Cue1_First_OnOff.vi"() -> ("output_Cue1_First_OnOff"=w1389:i32)  [unwired: 11 in]
              n682 = call "myRIO_BRig_RT_dataLC_Cue1_First_Probability.vi"() -> ("output_Cue1_First_Probability"=w1385:i32)  [unwired: 11 in]
              n683 = call "myRIO_BRig_RT_dataLC_Cue1_First_Tdelay.vi"() -> ("output_Cue1_First_Tdelay"=w1383:i32)  [unwired: 11 in]
              n684 = call "myRIO_BRig_RT_dataLC_Cue1_First_Count.vi"() -> ("output_Cue1_First_Count"=w1381:i32)  [unwired: 11 in]
              n685 = call "myRIO_BRig_RT_dataLC_Cue1_All_Block.vi"() -> ("output_Cue1_All_Block"=w1365:i32)  [unwired: 11 in]
              n686 = call "myRIO_BRig_RT_dataLC_Cue1_All_OnOff.vi"() -> ("output_Cue1_All_OnOff"=w1364:i32)  [unwired: 11 in]
              n687 = call "myRIO_BRig_RT_dataLC_Cue1_All_Probability.vi"() -> ("output_Cue1_All_Probability"=w1363:i32)  [unwired: 11 in]
              n688 = call "myRIO_BRig_RT_dataLC_Cue1_All_Tdelay.vi"() -> ("output_Cue1_All_Tdelay"=w1362:i32)  [unwired: 11 in]
              n689 = call "myRIO_BRig_RT_dataLC_Cue1_All_Count.vi"() -> ("output_Cue1_All_Count"=w1361:i32)  [unwired: 11 in]
              n690 = call "myRIO_BRig_RT_dataLC_Cue1_All_delayOpt.vi"() -> ("output_Cue1_All_delayOpt"=w1360:i32)  [unwired: 11 in]
              n691 = local read "LC_Cue1_First_delayOpt"() -> (w1367:bool)
              n692 = local read "LC_Cue1_First_Count"() -> (w1380:u16)
              n693 = local read "LC_Cue1_First_Probability"() -> (w1384:u16)
              n694 = local read "LC_Cue1_First_Block"() -> (w1390:u16)
              n695 = local read "LC_Cue1_First_Tdelay"() -> (w1382:u16)
              n696 = local read "LC_Cue1_First_OnOff"() -> (w1388:bool)
              n697 = local read "LC_Cue1_All_OnOff"() -> (w1356:bool)
              n698 = local read "LC_Cue1_All_delayOpt"() -> (w1357:bool)
              n699 = local read "LC_Cue1_All_Probability"() -> (w1353:u16)
              n700 = local read "LC_Cue1_All_Tdelay"() -> (w1352:u16)
              n701 = local read "LC_Cue1_All_Count"() -> (w1351:u16)
              n702 = local read "LC_Cue1_All_Block"() -> (w1355:u16)
              n703 = Boolean To (0,1)(Boolean=w1367) -> (0, 1=w1369:i16)
              n704 = Boolean To (0,1)(Boolean=w1388) -> (0, 1=w1387:i16)
              n705 = Boolean To (0,1)(Boolean=w1356) -> (0, 1=w1359:i16)
              n706 = To Unsigned Word Integer(number=w1369) -> (unsigned 16bit integer=w1366:u16)
              n707 = To Unsigned Word Integer(number=w1387) -> (unsigned 16bit integer=w1386:u16)
              n708 = To Unsigned Word Integer(number=w1359) -> (unsigned 16bit integer=w1354:u16)
              n709 = Boolean To (0,1)(Boolean=w1357) -> (0, 1=w1358:i16)
              n710 = To Unsigned Word Integer(number=w1358) -> (unsigned 16bit integer=w1350:u16)
              n711 = Replace Array Subset(array=w1392, new element #1=w1390, index #1=w1391, new element #2=w1386, index #2=w1389, new element #3=w1384, index #3=w1385, new element #4=w1382, index #4=w1383, new element #5=w1380, index #5=w1381, new element #6=w1366, index #6=w1368, new element #7=w1355, index #7=w1365, new element #8=w1354, index #8=w1364, new element #9=w1353, index #9=w1363, new element #10=w1352, index #10=w1362, new element #11=w1351, index #11=w1361, new element #12=w1350, index #12=w1360) -> (w1393:u16[])
            }
            frame "saveSettings6_LC_Other" {
              # "Trial"
              # "Tdelay"
              # "Probability"
              # "OnOff"
              # "Block"
              # "Wrong"
              # "Trial"
              # "Tdelay"
              # "Probability"
              # "OnOff"
              # "Block"
              # "Reward"
              n712 = call "myRIO_BRig_RT_dataLC_Wrong_Block.vi"() -> ("output_Wrong_Block"=w1423:i32)  [unwired: 11 in]
              n713 = call "myRIO_BRig_RT_dataLC_Wrong_OnOff.vi"() -> ("output_Wrong_OnOff"=w1422:i32)  [unwired: 11 in]
              n714 = call "myRIO_BRig_RT_dataLC_Wrong_Probability.vi"() -> ("output_Wrong_Probability"=w1421:i32)  [unwired: 11 in]
              n715 = call "myRIO_BRig_RT_dataLC_Wrong_Tdelay.vi"() -> ("output_Wrong_Tdelay"=w1420:i32)  [unwired: 11 in]
              n716 = call "myRIO_BRig_RT_dataLC_Wrong_Trial.vi"() -> ("output_Wrong_Trial"=w1419:i32)  [unwired: 11 in]
              n717 = call "myRIO_BRig_RT_dataLC_Reward_Block.vi"() -> ("output_Reward_Block"=w1435:i32)  [unwired: 11 in]
              n718 = call "myRIO_BRig_RT_dataLC_Reward_OnOff.vi"() -> ("output_Reward_OnOff"=w1433:i32)  [unwired: 11 in]
              n719 = call "myRIO_BRig_RT_dataLC_Reward_Probability.vi"() -> ("output_Reward_Probability"=w1429:i32)  [unwired: 11 in]
              n720 = call "myRIO_BRig_RT_dataLC_Reward_Tdelay.vi"() -> ("output_Reward_Tdelay"=w1427:i32)  [unwired: 11 in]
              n721 = call "myRIO_BRig_RT_dataLC_Reward_Trial.vi"() -> ("output_Reward_Trial"=w1425:i32)  [unwired: 11 in]
              n722 = local read "LC_Wrong_OnOff"() -> (w1417:bool)
              n723 = local read "LC_Wrong_Probability"() -> (w1414:u16)
              n724 = local read "LC_Wrong_Block"() -> (w1416:u16)
              n725 = local read "LC_Wrong_Tdelay"() -> (w1413:u16)
              n726 = local read "LC_Wrong_Trial"() -> (w1412:u16)
              n727 = local read "LC_Reward_Probability"() -> (w1428:u16)
              n728 = local read "LC_Reward_Block"() -> (w1434:u16)
              n729 = local read "LC_Reward_Tdelay"() -> (w1426:u16)
              n730 = local read "LC_Reward_OnOff"() -> (w1432:bool)
              n731 = local read "LC_Reward_Trial"() -> (w1424:u16)
              n732 = Boolean To (0,1)(Boolean=w1417) -> (0, 1=w1418:i16)
              n733 = Boolean To (0,1)(Boolean=w1432) -> (0, 1=w1431:i16)
              n734 = To Unsigned Word Integer(number=w1418) -> (unsigned 16bit integer=w1415:u16)
              n735 = To Unsigned Word Integer(number=w1431) -> (unsigned 16bit integer=w1430:u16)
              n736 = Replace Array Subset(array=w1436, new element #1=w1434, index #1=w1435, new element #2=w1430, index #2=w1433, new element #3=w1428, index #3=w1429, new element #4=w1426, index #4=w1427, new element #5=w1424, index #5=w1425, new element #6=w1416, index #6=w1423, new element #7=w1415, index #7=w1422, new element #8=w1414, index #8=w1421, new element #9=w1413, index #9=w1420, new element #10=w1412, index #10=w1419) -> (w1437:u16[])
            }
            frame "setSettings_Audio" {
              # "amp_L"
              # "amp_R"
              # "freq_L"
              # "freq_R"
              n737 = call "myRIO_BRig_RT_dataExp_Audio_amp__L.vi"() -> ("output_Audio_amp__L"=w1460:i32)  [unwired: 11 in]
              n738 = call "myRIO_BRig_RT_dataExp_Audio_amp__R.vi"() -> ("output_Audio_amp__R"=w1459:i32)  [unwired: 11 in]
              n739 = call "myRIO_BRig_RT_dataExp_Audio_freq__L.vi"() -> ("output_Audio_freq__L"=w1458:i32)  [unwired: 11 in]
              n740 = call "myRIO_BRig_RT_dataExp_Audio_freq__R.vi"() -> ("output_Audio_freq__R"=w1457:i32)  [unwired: 11 in]
              n741 = Index Array(array=w1456, index #1=w1460, index #2=w1459, index #3=w1458, index #4=w1457) -> (element #1=w1455:u16, element #2=w1453:u16, element #3=w1454:u16, element #4=w1452:u16)
            }
            frame "setSettings_Laser" {
              (unwired) u32 0 ("tDelay_laser_rew")
              # "Wrong tDelay"
              # "Reward tDelay"
              n742 = call "myRIO_BRig_RT_dataLC_Reward_Tdelay.vi"() -> ("output_Reward_Tdelay"=w1486:i32)  [unwired: 11 in]
              n743 = call "myRIO_BRig_RT_dataLC_Wrong_Tdelay.vi"() -> ("output_Wrong_Tdelay"=w1487:i32)  [unwired: 11 in]
              n744 = Index Array(array=w1483, index #1=w1486, index #2=w1487) -> (element #1=w1485:u16, element #2=w1484:u16)
              n745 = call "myRIO_Brig_RT__covert_Voltage_to_FPGAvalue.vi"("input_voltage"="laser_power") -> ("output_PortC"=w1488:i16)  [unwired: 9 in, 1 out]
              n746 = call "myRIO_BRig_RT__calc_Tvalley.vi"("input_peakWidth"="laser_Tpeak", "input_freq"="laser_Freq") -> ("output_Tvalley"=w1494:dbl)  [unwired: 9 in]
              n747 = To Double Precision Float(number=w1485) -> (double precision float=w1480:dbl)
              n748 = To Double Precision Float(number=w1484) -> (double precision float=w1477:dbl)
              n749 = Multiply(x="f_millisec2count", y="laser_Tpeak") -> (x*y=w1503:dbl)
              n750 = Multiply(x="f_millisec2count", y=w1494) -> (x*y=w1500:dbl)
              n751 = Multiply(x="f_millisec2count", y="laser_Tshutter") -> (x*y=w1498:dbl)
              n752 = Round Toward +Infinity(x="laser_Tshutter") -> (ceil(x): smallest int >= x=w1489:dbl)
              n753 = Multiply(x="f_millisec2count", y=w1480) -> (x*y=w1481:dbl)
              n754 = Multiply(x="f_millisec2count", y=w1477) -> (x*y=w1478:dbl)
              n755 = Round Toward +Infinity(x=w1503) -> (ceil(x): smallest int >= x=w1504:dbl)
              n756 = Round Toward +Infinity(x=w1500) -> (ceil(x): smallest int >= x=w1501:dbl)
              n757 = Round Toward +Infinity(x=w1498) -> (ceil(x): smallest int >= x=w1493:dbl)
              n758 = Round Toward +Infinity(x=w1481) -> (ceil(x): smallest int >= x=w1482:dbl)
              n759 = Round Toward +Infinity(x=w1478) -> (ceil(x): smallest int >= x=w1479:dbl)
              n760 = To Unsigned Long Integer(number=w1504) -> (unsigned 32bit integer=w1502:u32)
              n761 = To Unsigned Long Integer(number=w1501) -> (unsigned 32bit integer=w1499:u32)
              n762 = To Unsigned Long Integer(number=w1493) -> (unsigned 32bit integer=w1497:u32)
              n763 = To Unsigned Word Integer(number=w1489) -> (unsigned 16bit integer=w1492:u16)
              n764 = To Unsigned Long Integer(number=w1482) -> (unsigned 32bit integer=w1476:u32)
              n765 = To Unsigned Long Integer(number=w1479) -> (unsigned 32bit integer=w1475:u32)
              n766 = Add(x="laser_duration", y=w1492) -> (x+y=w1471:u16)
              n767 = To Double Precision Float(number=w1471) -> (double precision float=w1470:dbl)
              n768 = Multiply(x=w1470, y="f_millisec2count") -> (x*y=w1473:dbl)
              n769 = call "myRIO_BRig_RT_dataCurrent_LaserPulse_duration.vi"() -> ("output_LaserPulse_duration"=w1505:i32)  [unwired: 11 in]
              n770 = Round Toward +Infinity(x=w1473) -> (ceil(x): smallest int >= x=w1474:dbl)
              n771 = To Unsigned Long Integer(number=w1474) -> (unsigned 32bit integer=w1469:u32)
              n772 = xnode "Read/Write Control"("FPGA VI Reference In"=w1507, "error in"=w1508, "laser_Npeak"=w1502, "laser_Nvalley"=w1499, "AnaOut_0"=w1488, "laser_Nshutter"=w1497, "laser_selRew_Ndelay"=w1476, "laser_selWro_NDelay"=w1475, "laser_selRew_Ntotal"=w1469, "laser_selWro_Ntotal"=w1469) -> ("error out"=→"error out":errorcluster)  [unwired: 1 out]
              n773 = Replace Array Subset(array=w1483, new element=w1471, index=w1505) -> (w1506:u16[])
            }
            frame "initBlock" {
              n774 = call "myRIO_Brig_RT__Case_Exp_State_initBlock.vi"("input_spout"=w1552, "input_dataExp"=w1550, "input_dataCurrent"=w1551) -> ("output_spout"=w1529:enum16{"Left", "Right"}, "output_state"=w1553:T2, "output_dataExp"=w1549:u16[], "output_dataCurrent"=w1535:u16[], "output_TpB_target"=→"TpB_target":u16)  [unwired: 4 in]
              "cSpout" <- w1529
              n775 = call "myRIO_BRig_RT_dataCurrent_iBlock.vi"() -> ("output_iBlock"=w1534:i32)  [unwired: 11 in]
              n776 = Index Array(array=w1535, index=w1534) -> (element=→"iBlock":u16)
            }
            frame "initBlock2" {
              n777 = local write "nRewards_cur"(u16 0 ("nRewards_cur")) -> ()
              n778 = call "myRIO_BRig_RT__Case_Exp_State_initBlock2.vi"("input_spout"=w1561, "input_dataBlock"=w1562, "input_dataCurrent"=w1560) -> ("idxDataBlock"=w1557:i32, "output_dataBlock"=w1559:u16[][])  [unwired: 7 in]
            }
            frame "initTrial" {
              n779 = call "myRIO_Brig_RT__Case_Exp_State_initTrial.vi"("input_dataExp"=w1591, "input_dataCurrent"=w1592) -> ("output_state"=w1593:T2, "output_dataExp"=w1590:u16[], "output_dataCurrent"=w1580:u16[])  [unwired: 7 in]
              n780 = call "myRIO_BRig_RT_dataCurrent_iTrial.vi"() -> ("output_iTrial"=w1579:i32)  [unwired: 11 in]
              n781 = Index Array(array=w1580, index=w1579) -> (element=→"iTrial":u16)
            }
            frame "initTrial2" {
              # "trialUntilReward"
              n782 = call "myRIO_BRig_RT__Case_Exp_subState_LC__initTrial.vi"("input_dataTrial"=w1601, "input_spout"=w1610, "input_dataCurrent"=w1599, "input_dataLC"=w1598) -> ("output_LC_Wrong"=w1611:bool, "output_LC_led_Wrong"=w1603:bool, "output_LC_Reward"=w1612:bool, "output_LC_led_Reward"=w1602:bool, "output_dataTrial"=w1600:u16[][])  [unwired: 2 in]
              n783 = Equal?(x=w1610, y=enum16{"Left", "Right"}."Right") -> (x = y?=w1608:bool)
              n784 = call "myRIO_BRig_RT_dataExp_ItrialUntilReward.vi"() -> ("output_I_trialUntilReward"=w1606:i32)  [unwired: 11 in]
              n785 = Index Array(array=w1607, index=w1606) -> (element=w1605:u16)
              n786 = Not Equal To 0?(x=w1605) -> (x != 0?=w1604:bool)
              n787 = xnode "Read/Write Control"("FPGA VI Reference In"=w1625, "error in"=w1624, "SelectionState"=FALSE, "laserResponse_reward"=w1612, "laserResponse_wrong"=w1611, "laserResponse_reward_LED"=w1602, "laserResponse_wrong_LED"=w1603, "Left(F)_or_Right(T)"=w1608, "ignoreWrong"=w1604) -> ("error out"=→"error_initTrial":errorcluster)  [unwired: 1 out]
            }
            frame "initTrial3" {
              n788 = call "myRIO_BRig_RT__Case_Exp_State_initTrial_dataTrial.vi"("input_spout"=w1631, "input_dataCurrent"=w1632, "input_dataTrial"=w1634) -> ("output_dataTrial"=w1633:u16[][])  [unwired: 7 in, 1 out]
            }
            frame "initTrial4" {
              n789 = call "myRIO_BRig_RT_dataCurrent_idxDataTrial.vi"() -> ("output_idxDataTrial"=w1658:i32)  [unwired: 11 in]
              n790 = call "myRIO_BRig_RT_dataTrial_activeRecording.vi"() -> ("output_activeRecording"=w1655:i32)  [unwired: 11 in]
              n791 = Index Array(array=w1660, index=w1658) -> (element=w1657:u16)
              n792 = Boolean To (0,1)(Boolean="Recording") -> (0, 1=w1654:i16)
              n793 = To Long Integer(number=w1657) -> (32bit integer=w1656:i32)
              n794 = To Unsigned Word Integer(number=w1654) -> (unsigned 16bit integer=w1653:u16)
              n795 = Replace Array Subset(array=w1659, new element=w1653, index (row)=w1656, index (col)=w1655) -> (w1652:u16[][])
              n796 = local write "Recording_p2"("Recording") -> ()
            }
            frame "initTrial_LC_ENL1" {
              n797 = call "myRIO_BRig_RT__Case_Exp_State_initTrial_LC_ENL1__v2.vi"("input_dataTrial"=w1684, "input_spout"=w1689, "input_dataBlock"=w1682, "input_dataLC"=w1690, "input_dataCurrent"=w1686) -> ("output_LC__ENL1"=w1688:bool, "output_LC_led__ENL1"=w1687:bool, "output_dataTrial"=w1683:u16[][], "output_dataCurrent"=w1685:u16[])  [unwired: 3 in]
            }
            frame "initTrial_LC_Cue1" {
              n798 = local write "Recording_p2"(FALSE ("Recording_p2")) -> ()
              n799 = call "myRIO_BRig_RT__Case_Exp_State_initTrial_LC_Cue1__v2.vi"("input_dataTrial"=w1712, "input_spout"=w1715, "input_dataBlock"=w1710, "input_dataLC"=w1716, "input_dataCurrent"=w1714) -> ("output_LC__Cue1"=w1708:bool, "output_LC_led__Cue1"=w1709:bool, "output_dataTrial"=w1711:u16[][], "output_dataCurrent"=w1713:u16[])  [unwired: 3 in]
            }
            frame "ENL1_pre" {
              # "ENL1_n"
              # "Tcycle"
              # "counter"
              n800 = call "myRIO_BRig_RT_dataCurrent_Tcycle_generic.vi"() -> ("output_Tcycle_generic"=w1762:i32)  [unwired: 11 in]
              n801 = call "myRIO_BRig_RT_dataCurrent_count_generic.vi"() -> ("output_count_generic"=w1764:i32)  [unwired: 11 in]
              n802 = call "myRIO_BRig_RT_dataCurrent_ENL.vi"() -> ("output_ENL"=w1761:i32)  [unwired: 11 in]
              n803 = call "myRIO_BRig_RT_dataCurrent_ENL1_n.vi"() -> ("output_ENL1_n"=w1733:i32)  [unwired: 11 in]
              n804 = Index Array(array=w1755, index #1=w1761, index #2=w1733) -> (element #1=w1760:u16, element #2=w1732:u16)
              n805 = Increment(x=w1732) -> (x+1=w1731:u16)
              n806 = Replace Array Subset(array=w1755, new element #1=u16 0 ("new element/subarray"), index #1=w1764, new element #2=w1760, index #2=w1762, new element #3=w1731, index #3=w1733) -> (w1759:u16[])
              n807 = Select(t=myRIO_BRig_RT__Case_Exp_stateList."ENL1Penalty_pre" ("Enum"), s=w1743, f=myRIO_BRig_RT__Case_Exp_stateList."ENL1" ("Enum")) -> (s? t:f=w1740:T2)
            }
            frame "ENL1" {
              n808 = call "myRIO_BRig_RT__Case_Exp_State_ENL1__v2.vi"("input_LC"=w1771, "I_lick"=w1775, "input_LC_led"=w1772, "input_laserOccurred"=w1767, "input_state"=w1781, "input_dataCurrent"=w1780) -> ("output_trigger_laser_led"=w1770:bool, "output_state"=w1778:T2, "output_dataCurrent"=w1779:u16[], "output_trigger_laser"=w1769:bool)  [unwired: 2 in]
              n809 = Or(x=w1770, y=w1767) -> (x .or. y?=w1773:bool)
            }
            frame "ENL1Penalty_pre" {
              # "Tcycle"
              # "counter"
              n810 = call "myRIO_BRig_RT_dataCurrent_Tcycle_generic.vi"() -> ("output_Tcycle_generic"=w1821:i32)  [unwired: 11 in]
              n811 = call "myRIO_BRig_RT_dataCurrent_count_generic.vi"() -> ("output_count_generic"=w1823:i32)  [unwired: 11 in]
              n812 = call "myRIO_BRig_RT_dataExp_ENL_penalty.vi"() -> ("output_ENL_penalty"=w1816:i32)  [unwired: 11 in]
              n813 = Index Array(array=w1817, index=w1816) -> (element=w1820:u16)
              n814 = Replace Array Subset(array=w1818, new element #1=u16 0 ("new element/subarray"), index #1=w1823, new element #2=w1820, index #2=w1821) -> (w1819:u16[])
            }
            frame "ENL1Penalty" {
              n815 = call "myRIO_BRig_RT__Case_Exp_State_ENL1Penalty.vi"("input_state"=w1846, "input_dataCurrent"=w1850) -> ("output_state"=w1847:T2, "output_dataCurrent"=w1849:u16[])  [unwired: 8 in]
            }
            frame "ENL2_pre" {
            }
            frame "ENL2" {
            }
            frame "ENL2Penalty_pre" {
            }
            frame "ENL2Penalty" {
            }
            frame "Cue1_pre" {
              # "Cue1_n"
              # "Tcycle_Cue1"
              # "0 = L, 1 = R, 2 = both"
              # "sp_R"
              # "sp_L"
              # "Tcycle"
              # "counter"
              n816 = Equal?(x=w1961, y=enum16{"Left", "Right"}."Left") -> (x = y?=w1960:bool)
              n817 = call "myRIO_BRig_RT_dataExp_Audio_sp__L.vi"() -> ("output_Audio_sp__L"=w1959:i32)  [unwired: 11 in]
              n818 = call "myRIO_BRig_RT_dataExp_Audio_sp__R.vi"() -> ("output_Audio_sp__R"=w1958:i32)  [unwired: 11 in]
              n819 = call "myRIO_BRig_RT_dataCurrent_Tcycle_generic.vi"() -> ("output_Tcycle_generic"=w1971:i32)  [unwired: 11 in]
              n820 = call "myRIO_BRig_RT_dataCurrent_count_generic.vi"() -> ("output_count_generic"=w1973:i32)  [unwired: 11 in]
              n821 = Select(t=w1959, s=w1960, f=w1958) -> (s? t:f=w1957:i32)
              n822 = call "myRIO_BRig_RT_dataCurrent_Cue1_n.vi"() -> ("output_Cue1_n"=w1935:i32)  [unwired: 11 in]
              n823 = call "myRIO_BRig_RT_dataCurrent_Tcycle_cue.vi"() -> ("output_Tcycle_cue"=w1944:i32)  [unwired: 11 in]
              n824 = Index Array(array=w1963, index=w1957) -> (element=w1955:u16)
              n825 = Index Array(array=w1945, index #1=w1944, index #2=w1935) -> (element #1=w1946:u16, element #2=w1937:u16)
              n826 = Increment(x=w1937) -> (x+1=w1936:u16)
              n827 = Not Equal To 0?(x=w1955) -> (x != 0?=w1953:bool)
              n828 = Not Equal?(x=w1955, y=u16 1) -> (x != y?=w1954:bool)
              n829 = Replace Array Subset(array=w1945, new element #1=u16 0 ("new element/subarray"), index #1=w1973, new element #2=w1946, index #2=w1971, new element #3=w1936, index #3=w1935) -> (w1970:u16[])
              n830 = Select(t=myRIO_BRig_RT__Case_Exp_stateList."Cue1Penalty_pre" ("Enum"), s=w1941, f=myRIO_BRig_RT__Case_Exp_stateList."Cue1" ("Enum")) -> (s? t:f=w1942:T2)
            }
            frame "Cue1" {
              n831 = call "myRIO_BRig_RT__Case_Exp_State_Cue1__v2.vi"("input_LC"=w1983, "I_lick"=w1986, "input_LC_led"=w1984, "input_laserOccurred"=w1978, "input_state"=w1988, "input_dataCurrent"=w2006) -> ("output_trigger_laser_led"=w1981:bool, "output_state"=w1987:T2, "output_dataCurrent"=w2005:u16[], "output_trigger_laser"=w1982:bool)  [unwired: 2 in]
              n832 = Or(x=w1981, y=w1978) -> (x .or. y?=w1980:bool)
              n833 = Equal?(x=myRIO_BRig_RT__Case_Exp_stateList."Selection_pre", y=w1987) -> (x = y?=w1991:bool)
              n834 = xnode "Read/Write Control"("FPGA VI Reference In"=w1990, "error in"=w1989, "SelectionState"=w1991) -> ()  [unwired: 2 out]
            }
            frame "Cue1Penalty_pre" {
              # "Tcycle"
              # "counter"
              n835 = call "myRIO_BRig_RT_dataCurrent_Tcycle_generic.vi"() -> ("output_Tcycle_generic"=w2037:i32)  [unwired: 11 in]
              n836 = call "myRIO_BRig_RT_dataCurrent_count_generic.vi"() -> ("output_count_generic"=w2039:i32)  [unwired: 11 in]
              n837 = call "myRIO_BRig_RT_dataExp_Tcycle_CuePenalty.vi"() -> ("output_Tcycle_CuePenalty"=w2036:i32)  [unwired: 11 in]
              n838 = Index Array(array=w2031, index=w2036) -> (element=w2035:u16)
              n839 = Replace Array Subset(array=w2033, new element #1=u16 0 ("new element/subarray"), index #1=w2039, new element #2=w2035, index #2=w2037) -> (w2032:u16[])
            }
            frame "Cue1Penalty" {
              # "reset laserOccurred"
              n840 = call "myRIO_BRig_RT__Case_Exp_State_Cue1Penalty.vi"("input_state"=w2063, "input_dataCurrent"=w2064) -> ("output_state"=w2061:T2, "output_dataCurrent"=w2062:u16[])  [unwired: 8 in]
            }
            frame "Cue2_pre" {
              n841 = call "myRIO_BRig_RT__Case_Exp_subState_LC__Cue2.vi"("input_spout"=w2081, "input_dataCurrent"=w2082, "input_dataLC"=w2080) -> ()  [unwired: 6 in, 2 out]
            }
            frame "Cue2" {
            }
            frame "Cue2Penalty_pre" {
            }
            frame "Cue2Penalty" {
            }
            frame "Selection_pre" {
              # "Tcycle"
              # "counter"
              n842 = xnode "Read/Write Control"("FPGA VI Reference In"=w2153, "error in"=w2154) -> ("error out"=→"error_Selection_pre":errorcluster, "SelectReward"=w2146:bool, "SelectWrong"=w2148:bool)  [unwired: 1 out]
              n843 = call "myRIO_BRig_RT_dataCurrent_Tcycle_generic.vi"() -> ("output_Tcycle_generic"=w2175:i32)  [unwired: 11 in]
              n844 = call "myRIO_BRig_RT_dataCurrent_count_generic.vi"() -> ("output_count_generic"=w2177:i32)  [unwired: 11 in]
              n845 = call "myRIO_BRig_RT_dataExp_Tcycle_Selection.vi"() -> ("output_Tcycle_Selection"=w2174:i32)  [unwired: 11 in]
              n846 = Index Array(array=w2171, index=w2174) -> (element=w2173:u16)
              n847 = Replace Array Subset(array=w2169, new element #1=u16 0 ("new element/subarray"), index #1=w2177, new element #2=w2173, index #2=w2175) -> (w2172:u16[])
              n848 = Or(x=w2146, y=w2148) -> (x .or. y?=w2147:bool)
              n849 = Select(t=myRIO_BRig_RT__Case_Exp_stateList."SelectReward_pre" ("Enum"), s=w2146, f=myRIO_BRig_RT__Case_Exp_stateList."SelectWrong_pre" ("Enum")) -> (s? t:f=w2152:T2)
              n850 = Select(t=w2152, s=w2147, f=myRIO_BRig_RT__Case_Exp_stateList."Selection" ("Enum")) -> (s? t:f=w2149:T2)
            }
            frame "Selection" {
              # "counter\nSelection"
              # "increment"
              # "get Tcycle"
              # "get count"
              n851 = xnode "Read/Write Control"("FPGA VI Reference In"=w2202, "error in"=w2201) -> ("error out"=→"error_Selection":errorcluster, "SelectReward"=w2198:bool, "SelectWrong"=w2199:bool)  [unwired: 1 out]
              n852 = call "myRIO_BRig_RT_dataCurrent_Tcycle_generic.vi"() -> ("output_Tcycle_generic"=w2195:i32)  [unwired: 11 in]
              n853 = call "myRIO_BRig_RT_dataCurrent_count_generic.vi"() -> ("output_count_generic"=w2188:i32)  [unwired: 11 in]
              n854 = Index Array(array=w2196, index #1=w2195, index #2=w2188) -> (element #1=w2187:u16, element #2=w2194:u16)
              n855 = call "myRIO_BRig_RT__increment_u16.vi"() -> ("output_increment__u16"=w2193:u16)  [unwired: 11 in]
              n856 = Add(x=w2194, y=w2193) -> (x+y=w2189:u16)
              n857 = Greater?(x=w2187, y=w2189) -> (0:w2181:bool)
              n858 = Select(t=w2192, s=w2181, f=myRIO_BRig_RT__Case_Exp_stateList."SelectTimeout_pre" ("Enum")) -> (s? t:f=w2182:T2)
              n859 = Select(t=w2189, s=w2181, f=w2187) -> (s? t:f=w2185:u16)
              n860 = call "myRIO_BRig_RT_dataCurrent_count_selection.vi"() -> ("output_count_generic"=w2186:i32)  [unwired: 11 in]
              n861 = Select(t=myRIO_BRig_RT__Case_Exp_stateList."SelectReward_pre" ("Enum"), s=w2198, f=myRIO_BRig_RT__Case_Exp_stateList."SelectWrong_pre" ("Enum")) -> (s? t:f=w2197:T2)
              n862 = Replace Array Subset(array=w2196, new element #1=w2185, index #1=w2188, new element #2=w2185, index #2=w2186) -> (w2191:u16[])
              n863 = Or(x=w2198, y=w2199) -> (x .or. y?=w2180:bool)
              n864 = Select(t=w2197, s=w2180, f=w2182) -> (s? t:f=w2200:T2)
            }
            frame "SelectReward_pre" {
              # "iState"
              # "Tcycle\nReward"
              # "nRewTrials"
              # "Tcycle\nGeneric"
              # "counter"
              n865 = call "myRIO_BRig_RT_dataCurrent_nRewTrials.vi"() -> ("output_nRewTrials"=w2234:i32)  [unwired: 11 in]
              n866 = Equal?(x=w2243, y=enum16{"Left", "Right"}."Left") -> (x = y?=w2244:bool)
              n867 = Index Array(array=w2235, index=w2234) -> (element=w2233:u16)
              n868 = call "myRIO_BRig_RT_dataExp_Tcycle_Reward__L.vi"() -> ("output_Tcycle_Reward__L"=w2247:i32)  [unwired: 11 in]
              n869 = call "myRIO_BRig_RT_dataExp_Tcycle_Reward__R.vi"() -> ("output_Tcycle_Reward__R"=w2248:i32)  [unwired: 11 in]
              n870 = Increment(x=w2233) -> (x+1=w2232:u16)
              n871 = Select(t=w2247, s=w2244, f=w2248) -> (s? t:f=w2246:i32)
              n872 = call "myRIO_BRig_RT__Case_Exp_subState_LC__Reward.vi"("input_spout"=w2243, "input_dataCurrent"=w2235, "input_dataLC"=w2242) -> ()  [unwired: 6 in, 2 out]
              n873 = call "myRIO_BRig_RT_dataCurrent_count_generic.vi"() -> ("output_count_generic"=w2237:i32)  [unwired: 11 in]
              n874 = call "myRIO_BRig_RT_dataCurrent_Tcycle_generic.vi"() -> ("output_Tcycle_generic"=w2238:i32)  [unwired: 11 in]
              n875 = Index Array(array=w2249, index=w2246) -> (element=w2239:u16)
              n876 = call "myRIO_BRig_RT_dataCurrent_iState.vi"() -> ("output_iState"=w2227:i32)  [unwired: 11 in]
              n877 = Replace Array Subset(array=w2235, new element #1=w2232, index #1=w2234, new element #2=u16 0 ("new element/subarray"), index #2=w2237, new element #3=w2239, index #3=w2238, new element #4=u16 1 ("new element/subarray"), index #4=w2227) -> (w2250:u16[])
            }
            frame "SelectReward" {
              n878 = call "myRIO_BRig_RT__Case_Exp_State_Reward.vi"("input_dataCurrent"=w2272, "input_state"=w2269, "input_spout"=w2266, "input_LC"=w2267, "input_dataLC"=w2268) -> ("output_dataCurrent"=w2271:u16[], "output_state"=w2270:T2, "output__L"=w2264:bool, "output__R"=w2265:bool)  [unwired: 6 in, 1 out]
            }
            frame "SelectRewardPost_pre" {
              # "nRewards"
              # "nRewTrials"
              # "Tcycle"
              # "counter"
              n879 = call "myRIO_BRig_RT_dataBlock_nRewards__L.vi"() -> ("output_nRewards__L"=w2288:i32)  [unwired: 11 in]
              n880 = call "myRIO_BRig_RT_dataBlock_nRewards__R.vi"() -> ("output_nRewards__R"=w2287:i32)  [unwired: 11 in]
              n881 = call "myRIO_BRig_RT_dataCurrent_Tcycle_generic.vi"() -> ("output_Tcycle_generic"=w2307:i32)  [unwired: 11 in]
              n882 = call "myRIO_BRig_RT_dataCurrent_count_generic.vi"() -> ("output_count_generic"=w2309:i32)  [unwired: 11 in]
              n883 = case shown="\"Left\", Default" w2281 {
                tunnel: w2293 -> [w2314 w2318]
                tunnel: [w2313 w2318] -> w2292
                tunnel: [w2315 w2316] -> w2291
                tunnel: w2290 -> [w2315 w2317]
                frame "Left", Default {
                  n884 = Increment(x=w2314) -> (x+1=w2313:u16)
                }
                frame "Right" {
                  n885 = Increment(x=w2317) -> (x+1=w2316:u16)
                }
              }
              "nRewards_Left" <- w2292
              "nRewards_Right" <- w2291
              n886 = Equal?(x=w2281, y=enum16{"Left", "Right"}."Left") -> (x = y?=w2280:bool)
              n887 = Select(t=w2288, s=w2280, f=w2287) -> (s? t:f=w2286:i32)
              n888 = call "myRIO_BRig_RT_dataExp_Tcycle_RewardPost.vi"() -> ("output_Tcycle_RewardPost"=w2303:i32)  [unwired: 11 in]
              n889 = call "myRIO_BRig_RT_dataCurrent_nRewTrials.vi"() -> ("output_nRewTrials"=w2289:i32)  [unwired: 11 in]
              n890 = Index Array(array=w2304, index=w2303) -> (element=w2306:u16)
              n891 = Index Array(array=w2283, index=w2289) -> (element=w2278:u16)
              n892 = Replace Array Subset(array=w2283, new element #1=u16 0 ("new element/subarray"), index #1=w2309, new element #2=w2306, index #2=w2307) -> (w2305:u16[])
              n893 = Replace Array Subset(array=w2285, new element=w2278, index (row)=w2279, index (col)=w2286) -> (w2284:u16[][])
              n894 = local write "nRewards_cur"(w2278) -> ()
            }
            frame "SelectRewardPost" {
              n895 = call "myRIO_BRig_RT__Case_Exp_State_RewardPost.vi"("input_state"=w2333, "input_dataCurrent"=w2336) -> ("output_state"=w2334:T2, "output_dataCurrent"=w2335:u16[])  [unwired: 8 in]
            }
            frame "SelectWrong_pre" {
              # "iState"
              # "Tcycle"
              # "counter"
              n896 = call "myRIO_BRig_RT_dataCurrent_Tcycle_generic.vi"() -> ("output_Tcycle_generic"=w2361:i32)  [unwired: 11 in]
              n897 = call "myRIO_BRig_RT_dataCurrent_count_generic.vi"() -> ("output_count_generic"=w2363:i32)  [unwired: 11 in]
              n898 = call "myRIO_BRig_RT_dataExp_Tcycle_Wrong.vi"() -> ("output_Tcycle_Wrong"=w2359:i32)  [unwired: 11 in]
              n899 = call "myRIO_BRig_RT__Case_Exp_subState_LC__Wrong.vi"("input_spout"=w2355, "input_dataCurrent"=w2356, "input_dataLC"=w2353) -> ()  [unwired: 6 in, 2 out]
              n900 = Index Array(array=w2357, index=w2359) -> (element=w2360:u16)
              n901 = call "myRIO_BRig_RT_dataCurrent_iState.vi"() -> ("output_iState"=w2347:i32)  [unwired: 11 in]
              n902 = Replace Array Subset(array=w2356, new element #1=u16 0 ("new element/subarray"), index #1=w2363, new element #2=w2360, index #2=w2361, new element #3=u16 2 ("new element/subarray"), index #3=w2347) -> (w2358:u16[])
            }
            frame "SelectWrong" {
              n903 = call "myRIO_BRig_RT__Case_Exp_State_Wrong.vi"("input_dataLC"=w2384, "input_LC"=w2383, "input_state"=w2377, "input_dataCurrent"=w2387) -> ("output_state"=w2374:T2, "output_dataCurrent"=w2386:u16[])  [unwired: 5 in, 1 out]
              n904 = Not Equal?(x=w2377, y=w2374) -> (x != y?=w2376:bool)
              n905 = Select(t=myRIO_BRig_RT__Case_Exp_stateList."SelectWrong_post" ("Enum"), s=w2376, f=w2374) -> (s? t:f=w2373:T2)
            }
            frame "SelectWrong_post" {
            }
            frame "SelectTimeout_pre" {
              # "iState"
              # "Tcycle"
              # "counter"
              n906 = xnode "Read/Write Control"("FPGA VI Reference In"=w2414, "error in"=w2413, "SelectionState"=FALSE) -> ("error out"=→"error out 3":errorcluster)  [unwired: 1 out]
              n907 = call "myRIO_BRig_RT_dataCurrent_Tcycle_generic.vi"() -> ("output_Tcycle_generic"=w2436:i32)  [unwired: 11 in]
              n908 = call "myRIO_BRig_RT_dataCurrent_count_generic.vi"() -> ("output_count_generic"=w2434:i32)  [unwired: 11 in]
              n909 = call "myRIO_BRig_RT_dataExp_Tcycle_Timeout.vi"() -> ("output_Tcycle_Timeout"=w2438:i32)  [unwired: 11 in]
              n910 = call "myRIO_BRig_RT__Case_Exp_subState_LC__Timeout.vi"("input_spout"=w2429, "input_dataCurrent"=w2430, "input_dataLC"=w2428) -> ()  [unwired: 6 in, 2 out]
              n911 = Index Array(array=w2432, index=w2438) -> (element=w2437:u16)
              n912 = call "myRIO_BRig_RT_dataCurrent_iState.vi"() -> ("output_iState"=w2422:i32)  [unwired: 11 in]
              n913 = Replace Array Subset(array=w2430, new element #1=u16 0 ("new element/subarray"), index #1=w2434, new element #2=w2437, index #2=w2436, new element #3=u16 3 ("new element/subarray"), index #3=w2422) -> (w2433:u16[])
            }
            frame "SelectTimeout" {
              n914 = call "myRIO_BRig_RT__Case_Exp_State_Timeout.vi"("input_dataLC"=w2457, "input_LC"=w2458, "input_state"=w2448, "input_dataCurrent"=w2463) -> ("output_state"=w2449:T2, "output_dataCurrent"=w2462:u16[])  [unwired: 5 in, 1 out]
              n915 = Not Equal?(x=w2448, y=w2449) -> (x != y?=w2452:bool)
              n916 = Select(t=myRIO_BRig_RT__Case_Exp_stateList."SelectTimeout_post" ("Enum"), s=w2452, f=w2449) -> (s? t:f=w2450:T2)
            }
            frame "SelectTimeout_post" {
            }
            frame "endTrial1" {
              # "Update dataBlock"
              n917 = call "myRIO_BRig_RT__Case_Exp_State_endTrial1.vi"("input_spout"=w2496, "input_dataBlock"=w2495, "input_dataCurrent"=w2493) -> ("output_dataBlock"=w2494:u16[][], "output_dataCurrent"=w2492:u16[])  [unwired: 7 in]
            }
            frame "endTrial2" {
              # "update dataTrial"
              n918 = call "myRIO_BRig_RT__Case_Exp_State_endTrial2.vi"("input_spout"=w2515, "input_dataTrial"=w2519, "input_dataCurrent"=w2517) -> ("output_dataTrial"=w2518:u16[][], "output_dataCurrent"=w2516:u16[])  [unwired: 7 in]
            }
            frame "endTrial3" {
              w2545 = myRIO_BRig_RT__Case_Exp_stateList."endBlock" ("Enum")
              # "nRewTrials"
              # "iTrial"
              # "I_blockUntilReward"
              # "TPB"
              # "end block?"
              n919 = local read "STOP_endTrial"() -> (w2543:bool)
              n920 = local read "STOP_abort"() -> (w2542:bool)
              n921 = xnode "Read/Write Control"("FPGA VI Reference In"=w2531, "error in"=w2530, "SelectionState"=FALSE) -> ("error out"=→"error out 2":errorcluster)  [unwired: 1 out]
              n922 = local read "START"() -> (w2540:bool)
              n923 = call "myRIO_BRig_RT_dataExp_IblockUntilReward.vi"() -> ("output_I_blockUntilReward"=w2552:i32)  [unwired: 11 in]
              n924 = Index Array(array=w2536, index=w2552) -> (element=w2532:u16)
              n925 = Not(x=w2540) -> (.not. x?=w2541:bool)
              n926 = Not Equal To 0?(x=w2532) -> (x != 0?=w2550:bool)
              n927 = Compound Arithmetic op=OR(w2543, w2541, w2542) -> (w2544:bool)
              n928 = call "myRIO_BRig_RT_dataCurrent_nRewTrials.vi"() -> ("output_nRewTrials"=w2548:i32)  [unwired: 11 in]
              n929 = call "myRIO_BRig_RT_dataCurrent_iTrial.vi"() -> ("output_iTrial"=w2549:i32)  [unwired: 11 in]
              n930 = Select(t=w2548, s=w2550, f=w2549) -> (s? t:f=w2547:i32)
              n931 = call "myRIO_BRig_RT_dataCurrent_TpB.vi"() -> ("output_TpB"=w2551:i32)  [unwired: 11 in]
              n932 = Index Array(array=w2537, index #1=w2551, index #2=w2547) -> (element #1=w2538:u16, element #2=w2539:u16)
              n933 = Less Or Equal?(x=w2538, y=w2539) -> (x <= y?=w2535:bool)
              n934 = Select(t=w2545, s=w2535, f=myRIO_BRig_RT__Case_Exp_stateList."empty_endTrial1" ("Enum")) -> (s? t:f=w2546:T2)
              n935 = Select(t=w2545, s=w2544, f=w2546) -> (s? t:f=w2533:T2)
            }
            frame "endBlock" {
              # "R"
              # "L"
              # "idxDataBlock"
              n936 = Equal?(x=w2576, y=enum16{"Left", "Right"}."Left") -> (x = y?=w2575:bool)
              n937 = call "myRIO_BRig_RT_dataCurrent_idxDataBlockL.vi"() -> ("output_idxDataBlock__L"=w2579:i32)  [unwired: 11 in]
              n938 = call "myRIO_BRig_RT_dataCurrent_idxDataBlockR.vi"() -> ("output_idxDataBlock__R"=w2578:i32)  [unwired: 11 in]
              n939 = Increment(x=w2570) -> (x+1=w2569:i32)
              n940 = Select(t=w2579, s=w2575, f=w2578) -> (s? t:f=w2573:i32)
              n941 = To Unsigned Word Integer(number=w2569) -> (unsigned 16bit integer=w2571:u16)
              n942 = local read "START"() -> (w2599:bool)
              n943 = local read "STOP_endBlock"() -> (w2594:bool)
              n944 = local read "STOP_endTrial"() -> (w2597:bool)
              n945 = local read "STOP_abort"() -> (w2596:bool)
              n946 = Replace Array Subset(array=w2574, new element=w2571, index=w2573) -> (w2572:u16[])
              n947 = Not(x=w2599) -> (.not. x?=w2598:bool)
              n948 = Compound Arithmetic op=OR(w2598, w2594, w2597, w2596) -> (w2595:bool)
              n949 = Select(t=myRIO_BRig_RT__Case_Exp_stateList."endExp" ("Enum"), s=w2595, f=myRIO_BRig_RT__Case_Exp_stateList."empty_endBlock1" ("Enum")) -> (s? t:f=w2603:T2)
            }
            frame "endExp" {
            }
            frame "commConnect" {
              n950 = call "myRIO_BRig_RT_comm_webdav_connect.vi"("input_password"="Host Password", "input_username"="Host UserName") -> ("output_Iconnected"=w2624:bool, "output_hSession"=w2642:T6)  [unwired: 7 in, 1 out]
              "Connected To Host?" <- w2624
              n951 = case shown="False" w2624 {
                frame False {
                  n952 = One Button Dialog(message="Connection Failed!\nData not being saved!") -> ()  [unwired: 1 in, 1 out]
                }
                frame True {
                }
              }
            }
            frame "commUpload_pre" {
              n953 = Select(t=myRIO_BRig_RT__Case_Exp_stateList."commUpload_dataBlock" ("Enum"), s=w2649, f=myRIO_BRig_RT__Case_Exp_stateList."endTrial3") -> (s? t:f=w2647:T2)
            }
            frame "commUpload_dataBlock" {
              n954 = call "myRIO_BRig_RT_comm_webdav_uploadFile__data.vi"("input_fileName_prefix"=w2670, "input_fileName"="dataBlock" ("input_filename"), "input_hSession"=w2672) -> ()  [unwired: 8 in, 1 out]
            }
            frame "commUpload_dataCurrent" {
              n955 = call "myRIO_BRig_RT_comm_webdav_uploadFile__data.vi"("input_fileName_prefix"=w2691, "input_fileName"="dataCurrent" ("input_filename"), "input_hSession"=w2693) -> ()  [unwired: 8 in, 1 out]
            }
            frame "commUpload_dataExp" {
              n956 = call "myRIO_BRig_RT_comm_webdav_uploadFile__data.vi"("input_fileName_prefix"=w2712, "input_fileName"="dataExp" ("input_filename"), "input_hSession"=w2714) -> ()  [unwired: 8 in, 1 out]
            }
            frame "commUpload_dataLC" {
              n957 = call "myRIO_BRig_RT_comm_webdav_uploadFile__data.vi"("input_fileName_prefix"=w2733, "input_fileName"="dataLC" ("input_filename"), "input_hSession"=w2735) -> ()  [unwired: 8 in, 1 out]
            }
            frame "commUpload_dataTrial" {
              n958 = call "myRIO_BRig_RT_comm_webdav_uploadFile__data.vi"("input_fileName_prefix"=w2757, "input_fileName"="dataTrial" ("input_filename"), "input_hSession"=w2759) -> ()  [unwired: 8 in, 1 out]
            }
            frame "saveData_dataBlock" {
              # "idxDataBlockR"
              # "idxDataBlockL"
              n959 = call "myRIO_BRig_RT_dataCurrent_idxDataBlockL.vi"() -> ("output_idxDataBlock__L"=w2783:i32)  [unwired: 11 in]
              n960 = call "myRIO_BRig_RT_dataCurrent_idxDataBlockR.vi"() -> ("output_idxDataBlock__R"=w2784:i32)  [unwired: 11 in]
              n961 = Index Array(array=w2785, index #1=w2783, index #2=w2784) -> (element #1=w2782:u16, element #2=w2781:u16)
              n962 = Greater?(x=w2782, y=w2781) -> (0:w2780:bool)
              n963 = Select(t=w2782, s=w2780, f=w2781) -> (s? t:f=w2778:u16)
              n964 = Increment(x=w2778) -> (x+1=w2777:u16)
              n965 = To Long Integer(number=w2777) -> (32bit integer=w2776:i32)
              n966 = Array Subset(array=w2779, length (row)=w2776) -> (w2775:u16[][])  [unwired: 3 in]
              n967 = call "myRIO_BRig_RT_comm_webdav_saveArrayToFile__2D_u16.vi"("Array"=w2775, "input_filename"="dataBlock") -> ()  [unwired: 10 in]
            }
            frame "saveData_dataCurrent" {
              n968 = call "myRIO_BRig_RT_comm_webdav_saveArrayToFile__1D_u16.vi"("Array"=w2804, "input_filename"="dataCurrent") -> ()  [unwired: 10 in]
            }
            frame "saveData_dataExp" {
              # "runTime"
              n969 = Get Date/Time In Seconds() -> (seconds since 1Jan1904=w2832:timestamp)
              n970 = To Double Precision Float(number=w2832) -> (double precision float=w2831:dbl)
              n971 = call "myRIO_BRig_RT_dataExp_runTime_seconds.vi"() -> ("output_RunTime_minutes"=w2830:i32)  [unwired: 11 in]
              n972 = Subtract(x=w2831, y=w2829) -> (x-y=w2826:dbl)
              n973 = To Unsigned Word Integer(number=w2826) -> (unsigned 16bit integer=w2825:u16)
              n974 = Replace Array Subset(array=w2824, new element=w2825, index=w2830) -> (w2827:u16[])
              n975 = call "myRIO_BRig_RT_comm_webdav_saveArrayToFile__1D_u16.vi"("Array"=w2827, "input_filename"="dataExp") -> ()  [unwired: 10 in]
            }
            frame "saveData_dataLC" {
              n976 = call "myRIO_BRig_RT_comm_webdav_saveArrayToFile__1D_u16.vi"("Array"=w2851, "input_filename"="dataLC") -> ()  [unwired: 10 in]
            }
            frame "saveData_dataTrial" {
              # "idxTrial"
              n977 = call "myRIO_BRig_RT_dataCurrent_idxDataTrial.vi"() -> ("output_idxDataTrial"=w2876:i32)  [unwired: 11 in]
              n978 = Index Array(array=w2877, index=w2876) -> (element=w2873:u16)
              n979 = Increment(x=w2873) -> (x+1=w2872:u16)
              n980 = To Long Integer(number=w2872) -> (32bit integer=w2871:i32)
              n981 = Array Subset(array=w2874, length (row)=w2871) -> (w2875:u16[][])  [unwired: 3 in]
              n982 = call "myRIO_BRig_RT_comm_webdav_saveArrayToFile__2D_u16.vi"("Array"=w2875, "input_filename"="dataTrial") -> ()  [unwired: 10 in]
            }
            frame "empty_endBlock1" {
            }
            frame "empty_endBlock2" {
            }
            frame "empty_endTrial1" {
            }
            frame "empty_endTrial2" {
            }
            frame "empty_endTrial3" {
            }
            frame "empty_endTrial4" {
            }
            frame "empty_endTrial5" {
            }
          }
          n983 = case shown="True" w1047 {
            tunnel: w1043 -> [w1070 w1078]
            tunnel: w1046 -> [_ w1074]
            tunnel: w1045 -> [_ w1073]
            tunnel: w1044 -> [_ w1072]
            tunnel: w1013 -> [_ w1071]
            tunnel: [w1070 w1077] -> w1042
            tunnel: w1041 -> [w1069 w1076]
            tunnel: [w1069 w1075] -> w1040
            frame False {
            }
            frame True {
              n984 = call "myRIO_BRig_RT__Case_Exp__recordLick.vi"("intput_state__trialEnd"=w1071, "intput_state__trialStart"=w1072, "input_lick__R"=w1073, "input_lick__L"=w1074, "input_dataCurrent"=w1076, "input_dataLick"=w1078) -> ("output_dataCurrent"=w1075:u16[], "output_dataLick"=w1077:u16[][])  [unwired: 4 in]
            }
          }
          n985 = Or(x=w1015, y=w1016) -> (x .or. y?=w1002:bool)
          n986 = Or(x=w1019, y=w999) -> (x .or. y?=w988:bool)
          n987 = Or(x=w998, y=w1020) -> (x .or. y?=w1014:bool)
          n988 = Or(x=w1018, y=w1017) -> (x .or. y?=w1003:bool)
          n989 = Or(x=w1048, y="STOP_abort") -> (x .or. y?=w1050:bool)
          n990 = Or(x=w977, y=w978) -> (x .or. y?=w975:bool)
          n991 = Or(x=w979, y=w978) -> (x .or. y?=w976:bool)
          n992 = xnode "Read/Write Control"("FPGA VI Reference In"=w990, "error in"=w989, "A1_SR"=w1003, "A3_SL"=w1002, "A6_Act"="Recording_p2", "audioTrigger_L"=w988, "audioAmp_L"=w1029, "audioFreq_L_Hz"=w997, "audioTrigger_R"=w1014, "audioAmp_R"=w1030, "audioFreq_R_Hz"=w1031, "laserledMTrig"=w975, "laserMTrig"=w976) -> ("FPGA VI Reference Out"=w1039:refnum<k20>, "error out"=w1038:errorcluster)
          n993 = node-c288() -> ()  [unwired: 1 in, 1 out]
          "cState" <- w1044
        }
        n994 = node-c288(w934) -> ()  [unwired: 1 out]
        n995 = flat-sequence {
          tunnel: w930 -> [w966]
          tunnel: w929 -> [w965]
          tunnel: [w964] -> w922
          tunnel: [w963] -> w921
          tunnel: [w970] -> w923
          tunnel: [w971] -> w928
          tunnel: w922 -> [w971]
          tunnel: w921 -> [w970]
          frame #0 {
            w967 = u16 0 ("AudioLeft_phase_inc")
            w962 = FALSE
            n996 = xnode "Read/Write Control"("FPGA VI Reference In"=w966, "error in"=w965, "Counts_Reset"=TRUE, "audioTrigger_L"=w962, "audioFreq_L_Hz"=w967, "audioAmp_L"=w967, "audioTrigger_R"=w962, "audioFreq_R_Hz"=w967, "audioAmp_R"=w967, "A3_SL"=w962, "A1_SR"=w962, "A6_Act"=w962) -> ("FPGA VI Reference Out"=w964:refnum<k20>, "error out"=w963:errorcluster)
          }
          frame #1 {
            w969 = FALSE ("START")
            n997 = local write "START"(w969) -> ()
            n998 = local write "STOP_endTrial"(w969) -> ()
            n999 = local write "STOP_endBlock"(w969) -> ()
          }
        }
        n1000 = stacked-sequence {
          tunnel: w906 -> [w942 _]
          tunnel: w904 -> [w943 _]
          tunnel: w903 -> [_ w948]
          tunnel: w902 -> [_ w947]
          tunnel: w901 -> [_ w946]
          tunnel: w900 -> [w936 _]
          frame #0 {
            n1001 = call "myRIO_BRig_RT_dataCurrent_idxDataLick.vi"() -> ("output_idxDataLick"=w937:i32)  [unwired: 11 in]
            n1002 = Index Array(array=w936, index=w937) -> (element=w939:u16)
            n1003 = Increment(x=w939) -> (x+1=w940:u16)
            n1004 = call "myRIO_BRig_RT_comm_webdav_saveArrayToFile__1D_u16.vi"("Array"=w943, "input_filename"="dataMTrig") -> ()  [unwired: 10 in]
            n1005 = To Long Integer(number=w940) -> (32bit integer=w938:i32)
            n1006 = Array Subset(array=w942, length (row)=w938) -> (w941:u16[][])  [unwired: 3 in]
            n1007 = call "myRIO_BRig_RT_comm_webdav_saveArrayToFile__2D_u16.vi"("Array"=w941, "input_filename"="dataLick") -> ()  [unwired: 10 in]
          }
          frame #1 {
            n1008 = case shown="True" w948 {
              tunnel: w947 -> [_ w950]
              tunnel: w946 -> [_ w949]
              frame False {
              }
              frame True {
                n1009 = stacked-sequence {
                  tunnel: w950 -> [w952 w959 w961]
                  tunnel: w949 -> [w953 w958 _]
                  frame #0 {
                    n1010 = call "myRIO_BRig_RT_comm_webdav_uploadFile__announce.vi"("input_addText"=TRUE, "input_fileName_prefix"=w953, "intput_fileName"="curExp_end", "intput_hSession"=w952) -> ("output_Isuccess"=w951:bool)  [unwired: 6 in, 1 out]
                    n1011 = case shown="True" w951 {
                      frame False {
                        n1012 = One Button Dialog(message="!!! Warning !!! Your data is located at C:\\BehaviorRig\\commTransfer") -> ()  [unwired: 1 in, 1 out]
                      }
                      frame True {
                        n1013 = Wait (ms)(milliseconds to wait=u32 20) -> ()  [unwired: 1 out]
                      }
                    }
                  }
                  frame #1 {
                    n1014 = call "myRIO_BRig_RT__endExp_sendData.vi"("input_fileName_prefix"=w958, "input_hSession"=w959) -> ()  [unwired: 8 in, 2 out]
                  }
                  frame #2 {
                    n1015 = local write "Connected To Host?"(FALSE ("Connected To Host?")) -> ()
                    n1016 = call <vilib>:"Close Session.vi"("session handle"=w961) -> ()  [unwired: 14 in, 1 out]
                  }
                }
              }
            }
          }
        }
      }
    }
    n1017 = local read "STOP_abort"() -> (w30:bool)
  }
  n1018 = xnode "Read/Write Control"("FPGA VI Reference In"=w8, "error in"=w7, "FPGA_Stop"=TRUE) -> ("FPGA VI Reference Out"=w13:refnum<k20>, "error out"=w14:errorcluster)
  n1019 = xnode "Close FPGA VI Reference"("FPGA VI Reference In"=w13, "error in"=w14) -> ("error out"=w12:errorcluster)
  n1020 = call <vilib>:"Reset myRIO.vi"("error in (no error)"=w12) -> ()  [unwired: 10 in, 1 out]
